vi "Autonomous Independent.vi"() -> ()   [LabVIEW 2016]
doc: "This VI is called when autonomous begins, and will automatically be terminated when autonomous ends. You can carry out timed or sensor driven robot movement independently without needing to return to the caller."
uses:
  <vilib>/Rock Robotics/WPI/Solenoid/WPI_SolenoidValue.ctl
  <vilib>/Rock Robotics/WPI/ThirdParty/CanMotor/TalonSRX/WPI_CANTalonSRX_APIControlMode.ctl
  <vilib>/Rock Robotics/Network Tables/NT Read String.vi
  <vilib>/Rock Robotics/WPI/Utilities/WPI_GetSetVariantRefNum.vi
  <vilib>/Rock Robotics/WPI/Solenoid/WPI_SolenoidSetEnum.vi
  <vilib>/Rock Robotics/Network Tables/NT Read Number.vi
  <vilib>/addons/control/pid/pid.llb/PID (DBL).vi
  Robot Global Data.vi
  <vilib>/Rock Robotics/Network Tables/NT Read Boolean.vi
  <vilib>/addons/control/pid/NI_PID_pid.lvlib
  navX Library v2/navX Library v2.lvlib
panel:
  out "DriveStraight 11":T1(graph)
  in  "ForwardPID 9":T2={"proportional gain (Kc)"=0.001, "integral time (Ti, min)"=0.1, "derivative time (Td, min)"=0.0}
  out "DriveStraight 10":T1(graph)
  in  "ForwardPID 8":T2={"proportional gain (Kc)"=0.001, "integral time (Ti, min)"=0.1, "derivative time (Td, min)"=0.0}
  out "DriveStraight 5":T1(graph)
  in  "ForwardPID 5":T2={"proportional gain (Kc)"=0.001, "integral time (Ti, min)"=0.1, "derivative time (Td, min)"=0.0}
  out "DriveStraight 4":T1(graph)
  in  "ForwardPID 4":T2={"proportional gain (Kc)"=0.001, "integral time (Ti, min)"=0.1, "derivative time (Td, min)"=0.0}
  in  "PID gains R 5":T2={"proportional gain (Kc)"=0.65, "integral time (Ti, min)"=0.01, "derivative time (Td, min)"=0.0} {"derivative time (Td, min)" format="%.3f"; "integral time (Ti, min)" format="%.6f"; "proportional gain (Kc)" format="%.6f"}
  in  "Range 5":cluster{"output high":dbl, "output low":dbl}={"output high"=1.0, "output low"=-0.5} {"output low" format="%.2f"; "output high" format="%.2f"}
  in  "PID gains L 5":T2={"proportional gain (Kc)"=0.65, "integral time (Ti, min)"=0.01, "derivative time (Td, min)"=0.0} {"derivative time (Td, min)" format="%.3f"; "integral time (Ti, min)" format="%.6f"; "proportional gain (Kc)" format="%.6f"}
  in  "PID gains R 4":T2={"proportional gain (Kc)"=0.65, "integral time (Ti, min)"=0.01, "derivative time (Td, min)"=0.0} {"derivative time (Td, min)" format="%.3f"; "integral time (Ti, min)" format="%.6f"; "proportional gain (Kc)" format="%.6f"}
  in  "Range 4":cluster{"output high":dbl, "output low":dbl}={"output high"=1.0, "output low"=-0.5} {"output low" format="%.2f"; "output high" format="%.2f"}
  in  "PID gains L 4":T2={"proportional gain (Kc)"=0.65, "integral time (Ti, min)"=0.01, "derivative time (Td, min)"=0.0} {"derivative time (Td, min)" format="%.3f"; "integral time (Ti, min)" format="%.6f"; "proportional gain (Kc)" format="%.6f"}
  in  "PID gains R 3":T2={"proportional gain (Kc)"=0.65, "integral time (Ti, min)"=0.01, "derivative time (Td, min)"=0.0} {"derivative time (Td, min)" format="%.3f"; "integral time (Ti, min)" format="%.6f"; "proportional gain (Kc)" format="%.6f"}
  in  "Range 3":cluster{"output high":dbl, "output low":dbl}={"output high"=1.0, "output low"=-0.5} {"output low" format="%.2f"; "output high" format="%.2f"}
  in  "PID gains L 3":T2={"proportional gain (Kc)"=0.65, "integral time (Ti, min)"=0.01, "derivative time (Td, min)"=0.0} {"derivative time (Td, min)" format="%.3f"; "integral time (Ti, min)" format="%.6f"; "proportional gain (Kc)" format="%.6f"}
  in  "PID gains R 2":T2={"proportional gain (Kc)"=0.65, "integral time (Ti, min)"=0.01, "derivative time (Td, min)"=0.0} {"derivative time (Td, min)" format="%.3f"; "integral time (Ti, min)" format="%.6f"; "proportional gain (Kc)" format="%.6f"}
  in  "Range 2":cluster{"output high":dbl, "output low":dbl}={"output high"=1.0, "output low"=-0.5} {"output low" format="%.2f"; "output high" format="%.2f"}
  in  "PID gains L 2":T2={"proportional gain (Kc)"=0.65, "integral time (Ti, min)"=0.01, "derivative time (Td, min)"=0.0} {"derivative time (Td, min)" format="%.3f"; "integral time (Ti, min)" format="%.6f"; "proportional gain (Kc)" format="%.6f"}
  in  "Fizone":dbl=3000.0
  in  "FI":dbl=0.001
  in  "FP":dbl=0.2
  in  "FrontSpeed":dbl=-22000.0
  out "DriveStraight 7":T1(graph)
  out "DriveStraight 6":T1(graph)
  in  "ForwardPID 3":T2={"proportional gain (Kc)"=0.001, "integral time (Ti, min)"=0.1, "derivative time (Td, min)"=0.0}
  in  "Hizone":dbl=3000.0
  in  "sizone":dbl=3000.0
  in  "ShootSpeed":dbl=-20000.0
  in  "SI":dbl=0.001
  in  "SP":dbl=0.2
  in  "HI":dbl=0.001
  in  "HP":dbl=0.2
  in  "HopperSpeed":dbl=-22000.0
  out "DriveStraight 3":T1(graph)
  out "DriveStraight 2":T1(graph)
  in  "ForwardPID 2":T2={"proportional gain (Kc)"=0.001, "integral time (Ti, min)"=0.1, "derivative time (Td, min)"=0.0}
  in  "RightPID":T2
  in  "ForwardPID":T2={"proportional gain (Kc)"=0.001, "integral time (Ti, min)"=0.1, "derivative time (Td, min)"=0.0}
  out "DriveStraight":T1(graph)
  in  "Center":dbl=160.0 format="%#_13g"
  in  "MOE":dbl=25.0 format="%#_13g"
  in  "Speed 2":dbl=0.45 format="%#_13g"
  in  "PID gains L":T2={"proportional gain (Kc)"=0.65, "integral time (Ti, min)"=0.01, "derivative time (Td, min)"=0.0} {"derivative time (Td, min)" format="%.3f"; "integral time (Ti, min)" format="%.6f"; "proportional gain (Kc)" format="%.6f"}
  in  "PID gains R":T2={"proportional gain (Kc)"=0.65, "integral time (Ti, min)"=0.01, "derivative time (Td, min)"=0.0} {"derivative time (Td, min)" format="%.3f"; "integral time (Ti, min)" format="%.6f"; "proportional gain (Kc)" format="%.6f"}
  in  "Range":cluster{"output high":dbl, "output low":dbl}={"output high"=1.0, "output low"=-0.5} {"output low" format="%.2f"; "output high" format="%.2f"}
  in  "Speed":dbl=1.0 format="%#_13g"
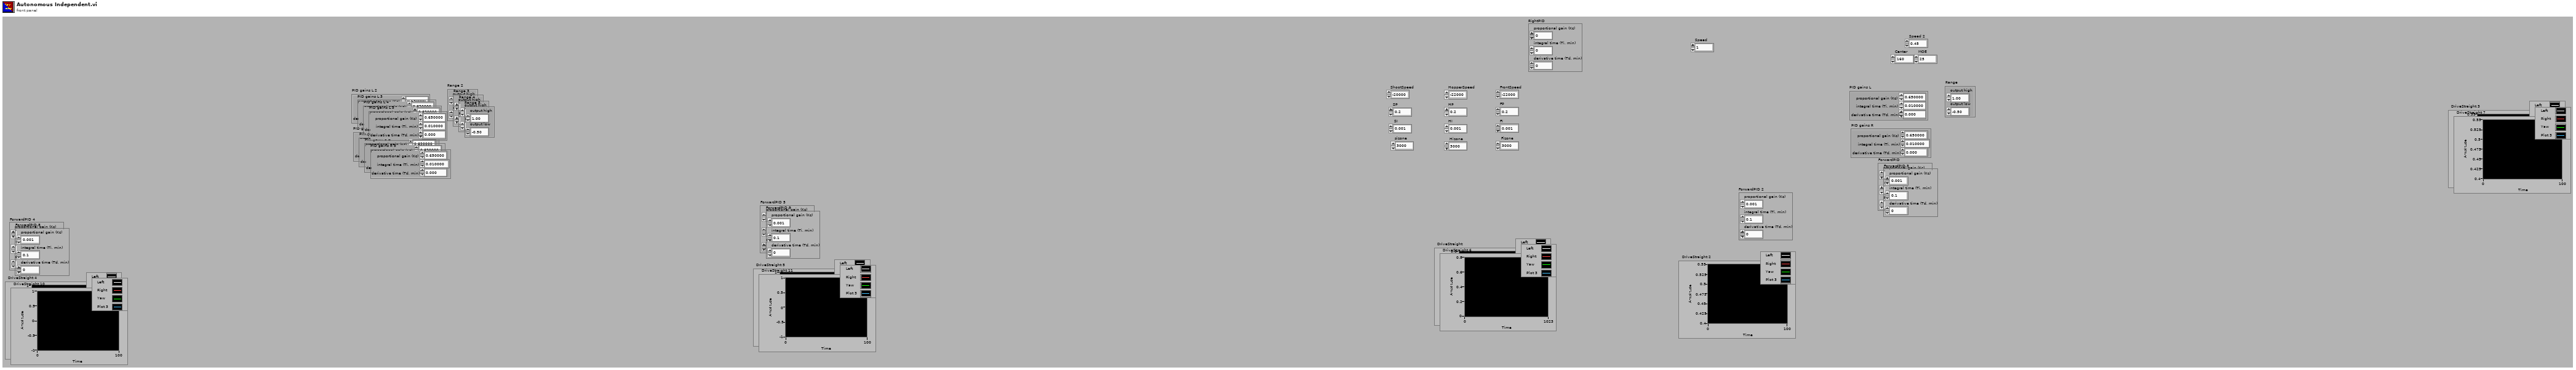
[diagram p1: front panel]
types:
  T1 = cluster{"[0]":dbl, "[1]":dbl, "[2]":dbl, "[3]":dbl, "[4]":dbl, "[5]":dbl, "[6]":dbl, "[7]":dbl, "[8]":dbl}
  T2 = cluster{"proportional gain (Kc)":dbl, "integral time (Ti, min)":dbl, "derivative time (Td, min)":dbl}
  T3 = typedef "WPI_SolenoidValue.ctl" = enum16{"Off", "On", "Forward", "Reverse"}
  T4 = typedef "WPI_CANTalonSRX_APIControlMode.ctl" = enum8{"Percent VBus", "Speed", "Position", "Slave", "Unchanged / Invalid", "Voltage Compensation", "Current", "Motion Profile", "Motion Magic"}
  T5 = typedef "WPI_RobotDriveDevRef.ctl" = cluster{"DevStatus":errorcluster, "Motors[]":T6[], "Square Inputs":bool, "Max Output":dbl}
  T6 = typedef "WPI_MotorControlDeviceRef.ctl" = cluster{"DeviceStatus":errorcluster, "Type":T7, "PWM":cluster{"PWM Channel":T8, "DeadBand":T9}, "CAN":cluster{"Device Number":u8, "SetOutput VI Ref":variant, "GetOutput VI Ref":variant, "Enable VI Ref":variant, "Disable VI Ref":variant, "Data":variant}, "Invert":bool}
  T7 = typedef "WPI_MotorControlType.ctl" = enum16{"PWM", "CAN"}
  T8 = typedef "FPGA_DIOPWMChannel.ctl" = enum8{"PWM 0", "PWM 1", "PWM 2", "PWM 3", "PWM 4", "PWM 5", "PWM 6", "PWM 7", "PWM 8", "PWM 9", "PWM MXP 0", "PWM MXP 1", "PWM MXP 2", "PWM MXP 3", "PWM MXP 4", "PWM MXP 5", "PWM MXP 6", "PWM MXP 7", "PWM MXP 8", "PWM MXP 9", "Invalid"}
  T9 = typedef "WPI_PWMDeadband.ctl" = cluster{"Name":string, "maxPositivePwm":i32, "minPositivePwm":i32, "centerPwm":i32, "maxNegativePwm":i32, "minNegativePwm":i32, "angularRange":u16}
  T10 = typedef "WPI_SolenoidDevRef.ctl" = cluster{"DevStatus":errorcluster, "Pneumatics Control Module":u8, "Forward Solenoid Channel":T11, "Reverse Solenoid Channel":T11}
  T11 = typedef "WPI_SolenoidChannel.ctl" = enum8{"Solenoid 0", "Solenoid 1", "Solenoid 2", "Solenoid 3", "Solenoid 4", "Solenoid 5", "Solenoid 6", "Solenoid 7", "Invalid"}
  T12 = typedef "navX Library v2.lvlib/Z900_navX_DeviceTypeDef.ctl" = cluster{"Interface":cluster{"Protocol":T13, "Update Rate (4Hz-100Hz)":u8, "navX Open TypeDef":variant}, "Notify Packet":refnum<notifier>, "Loop VI Refnum":refnum<vi>, "Ready to Close Occurrence Refnum":refnum<k4>}
  T13 = typedef "navX Library v2.lvlib/Z900_navX_ProtocolTypeDef.ctl" = enum16{"SERIAL", "I2C", "SPI"}
  T14 = typedef "WPI_EncoderDevRef.ctl" = cluster{"DevStatus":errorcluster, "EncoderIndex":T15, "CounterIndex":T16, "DistancePerCount":dbl, "Decoding Type":T17}
  T15 = typedef "FPGA_EncoderIdx.ctl" = enum8{"Enc 0", "Enc 1", "Enc 2", "Enc 3", "Enc 4", "Enc 5", "Enc 6", "Enc 7", "Invalid"}
  T16 = typedef "FPGA_CounterCtrSystemIndex.ctl" = enum8{"Ctr 0", "Ctr 1", "Ctr 2", "Ctr 3", "Ctr 4", "Ctr 5", "Ctr 6", "Ctr 7", "Invalid"}
  T17 = typedef "WPI_EncoderType.ctl" = enum16{"1x", "2x", "4x"}
  T18 = cluster{"Yaw":dbl, "Roll":dbl, "Pitch":dbl, "Heading":dbl, "Fused Heading":dbl}
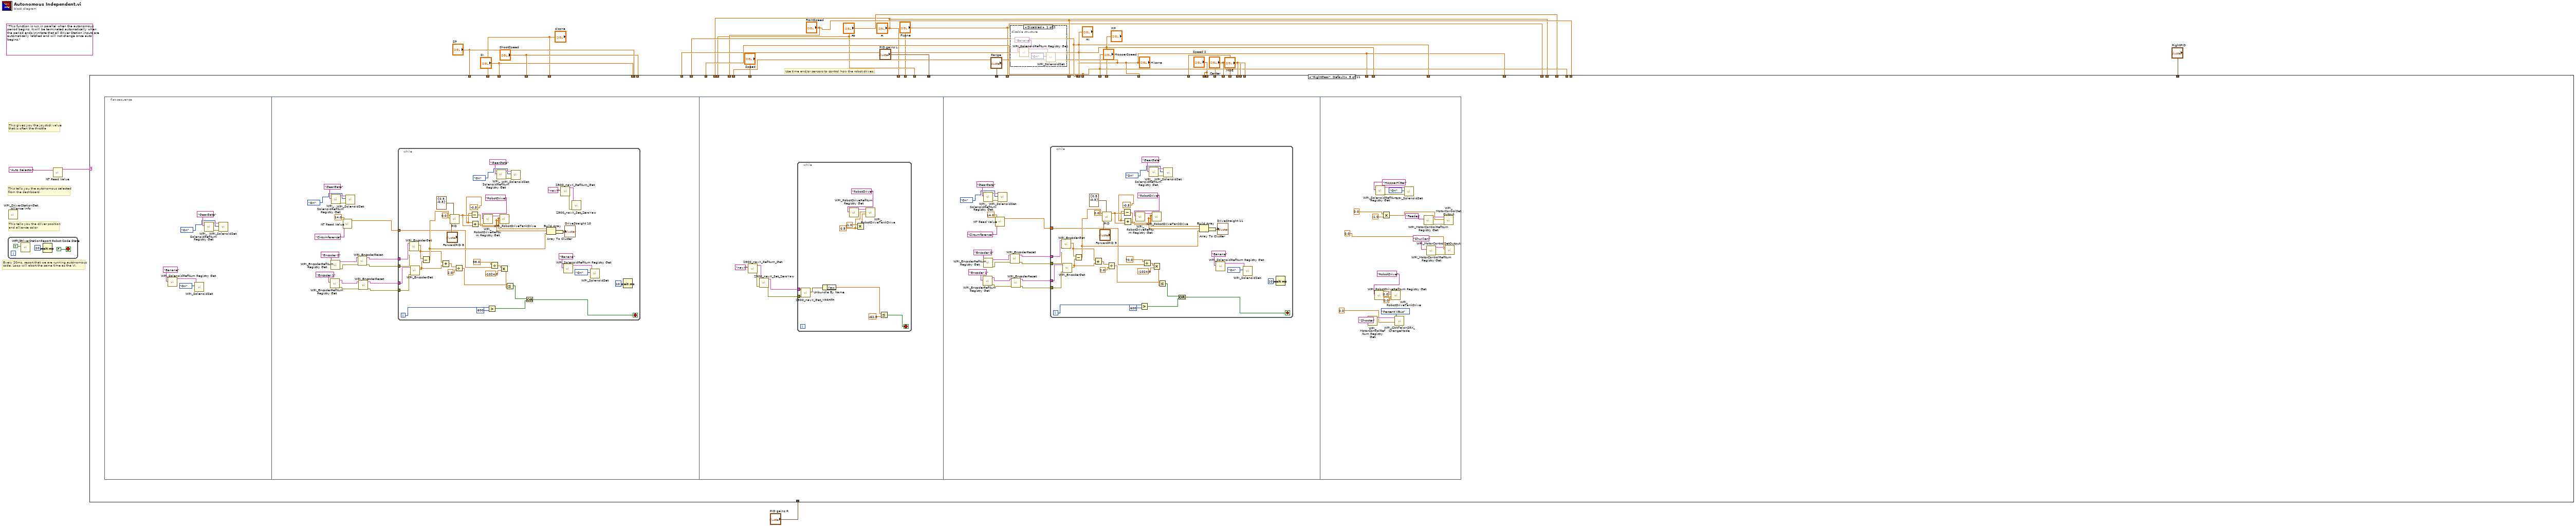
[diagram p0: block diagram]
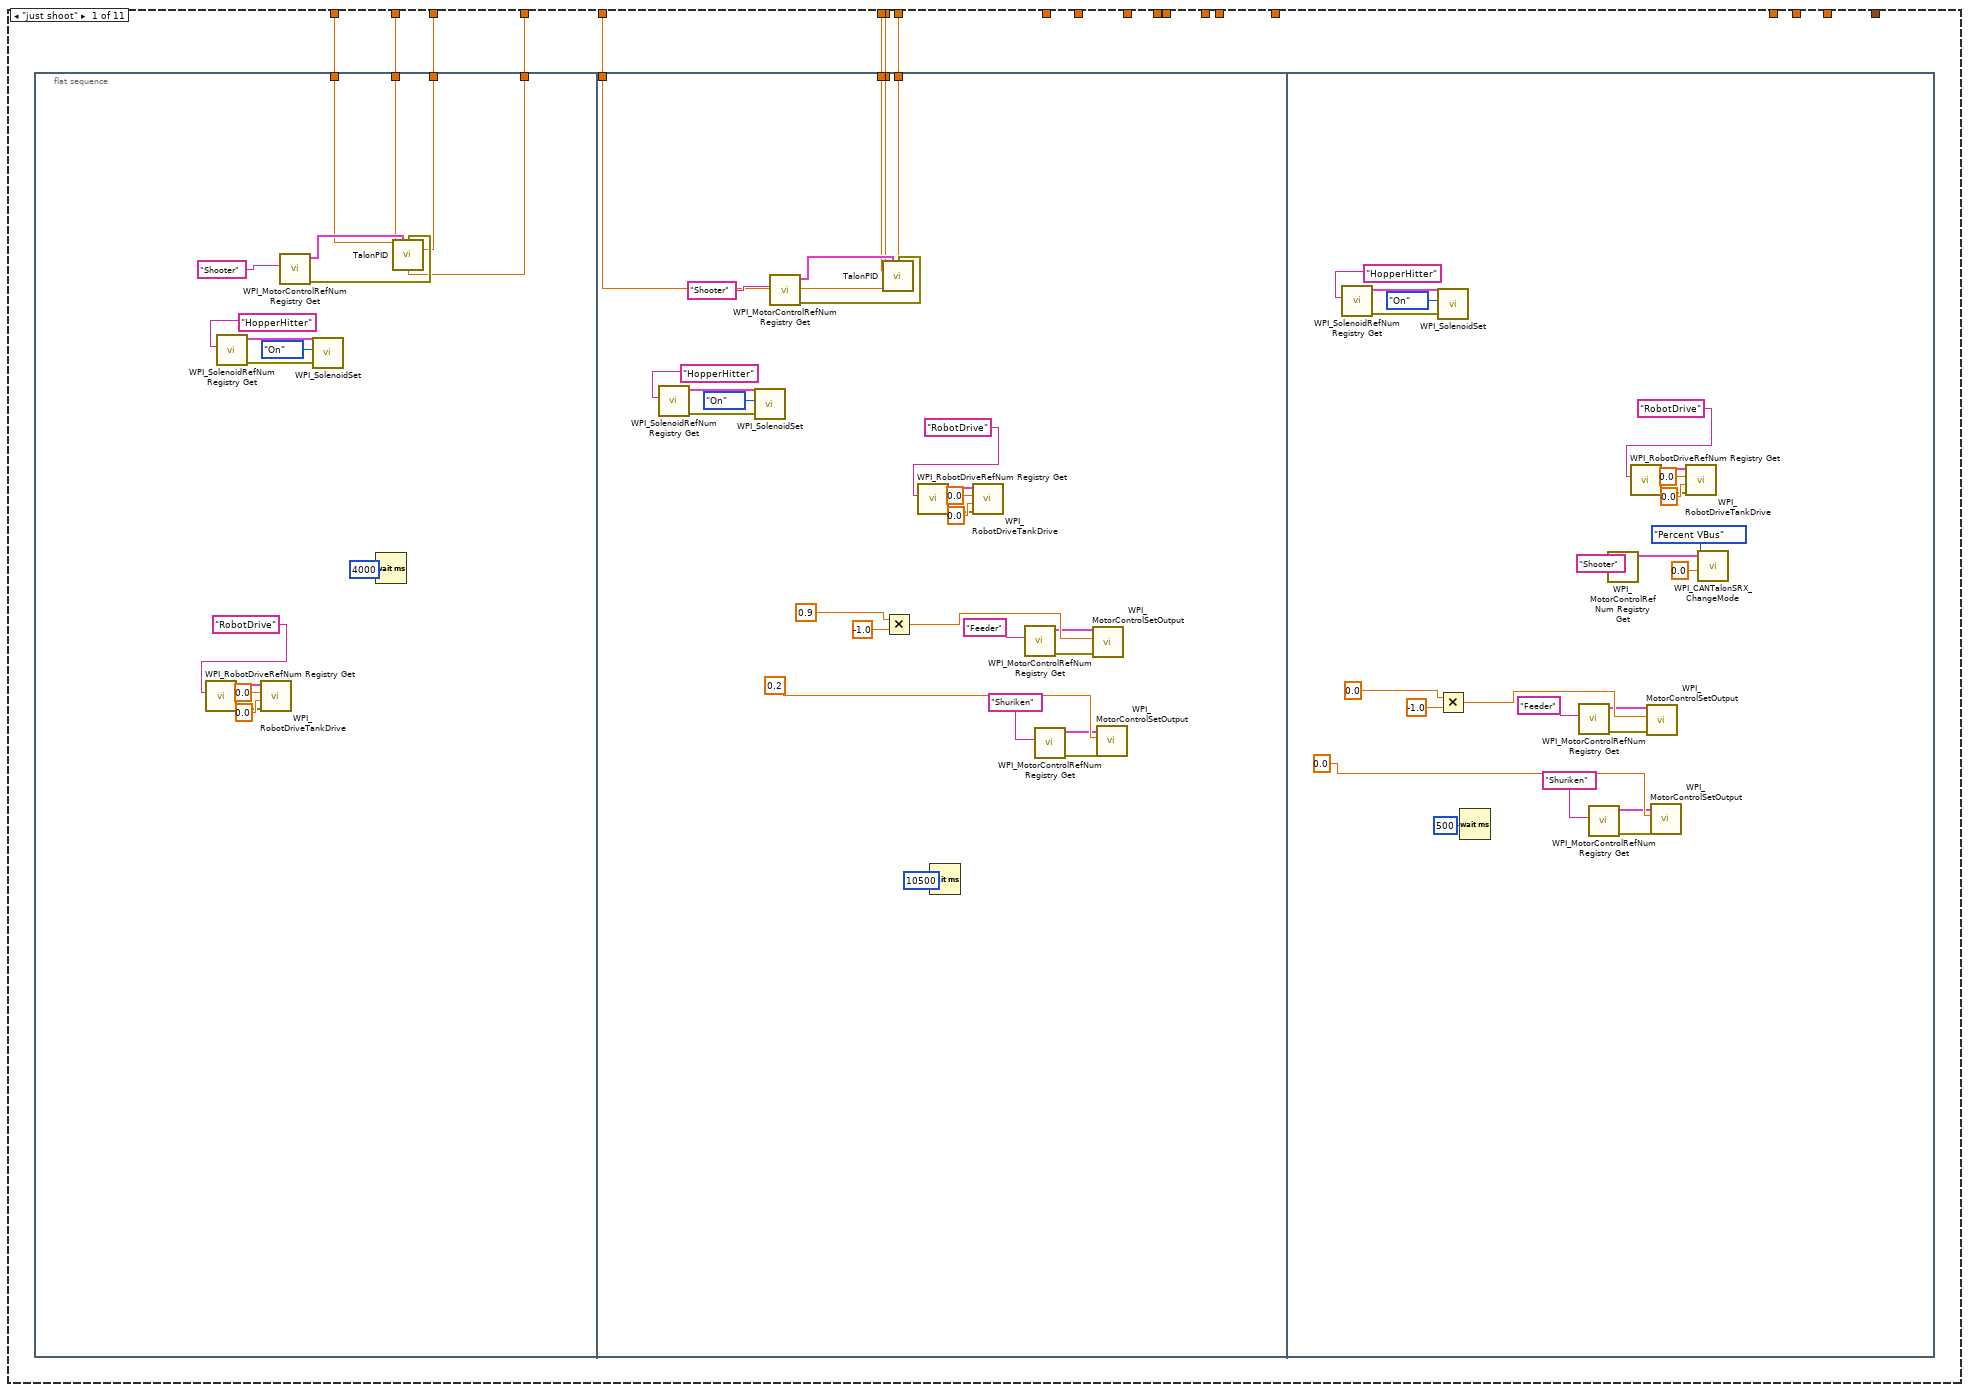
[diagram p3: hidden frame]
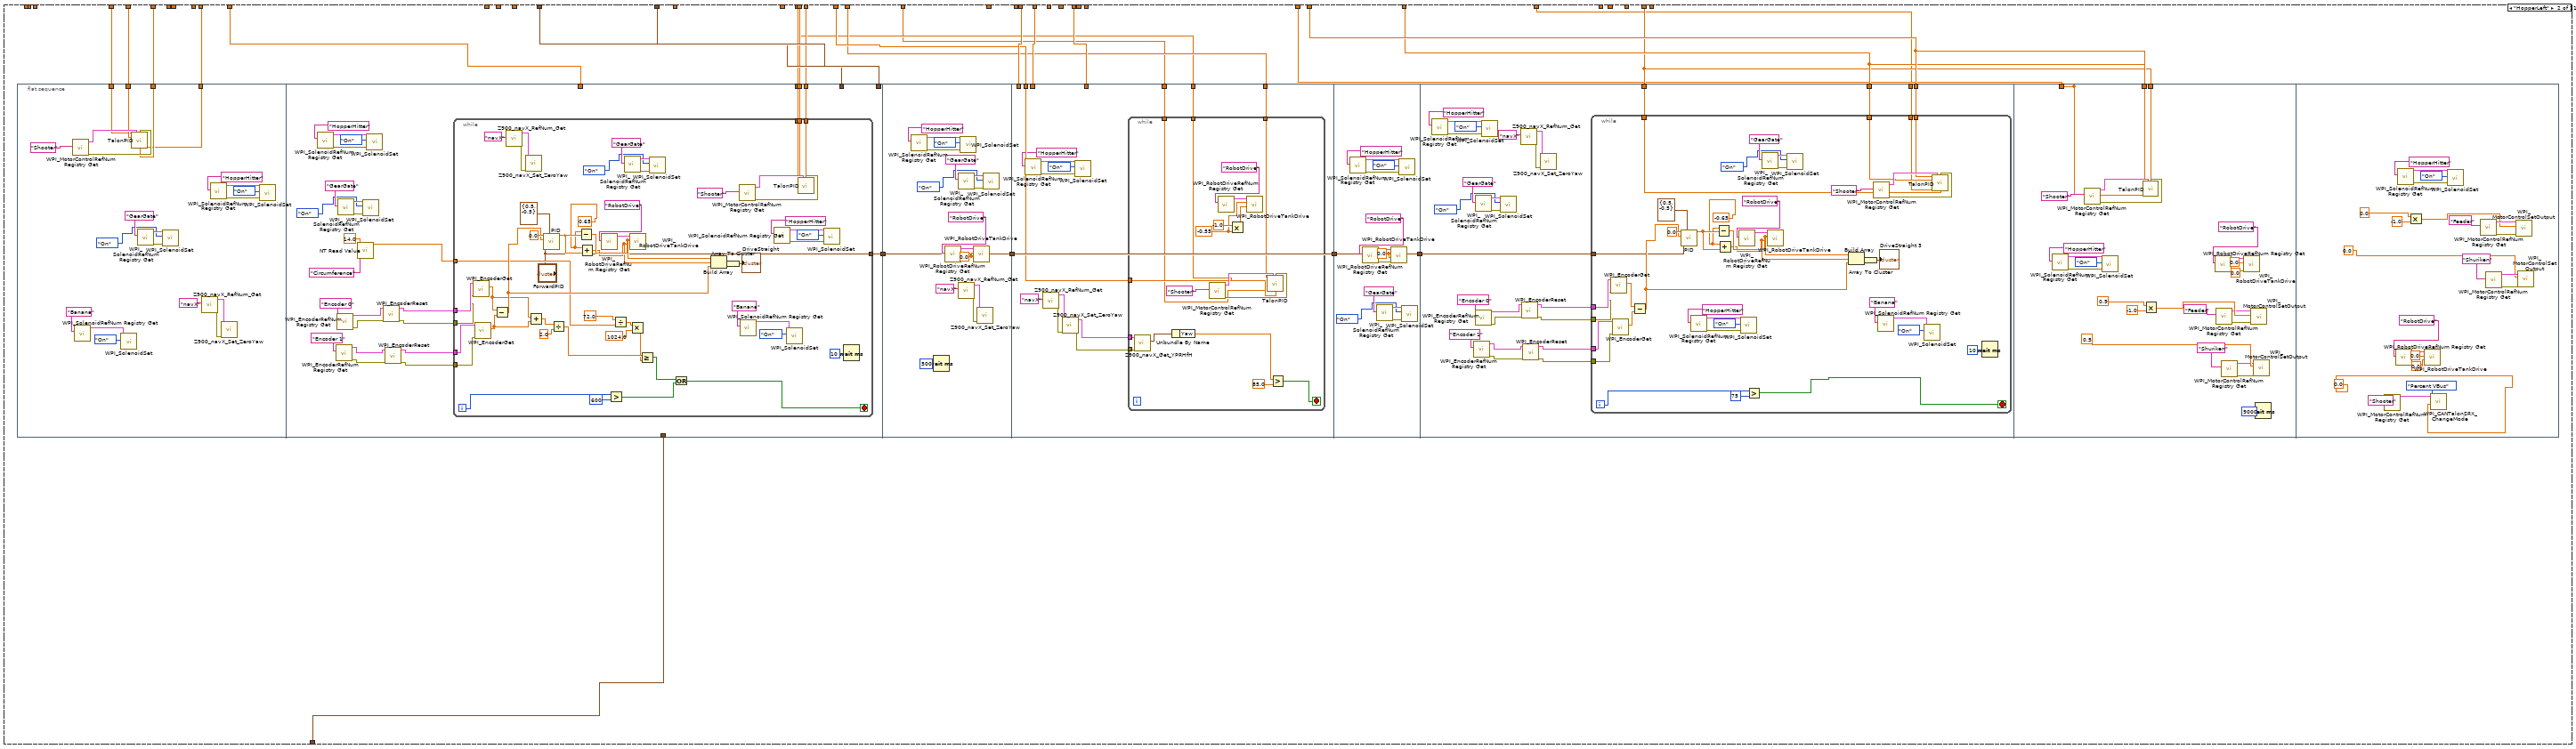
[diagram p4: hidden frame]
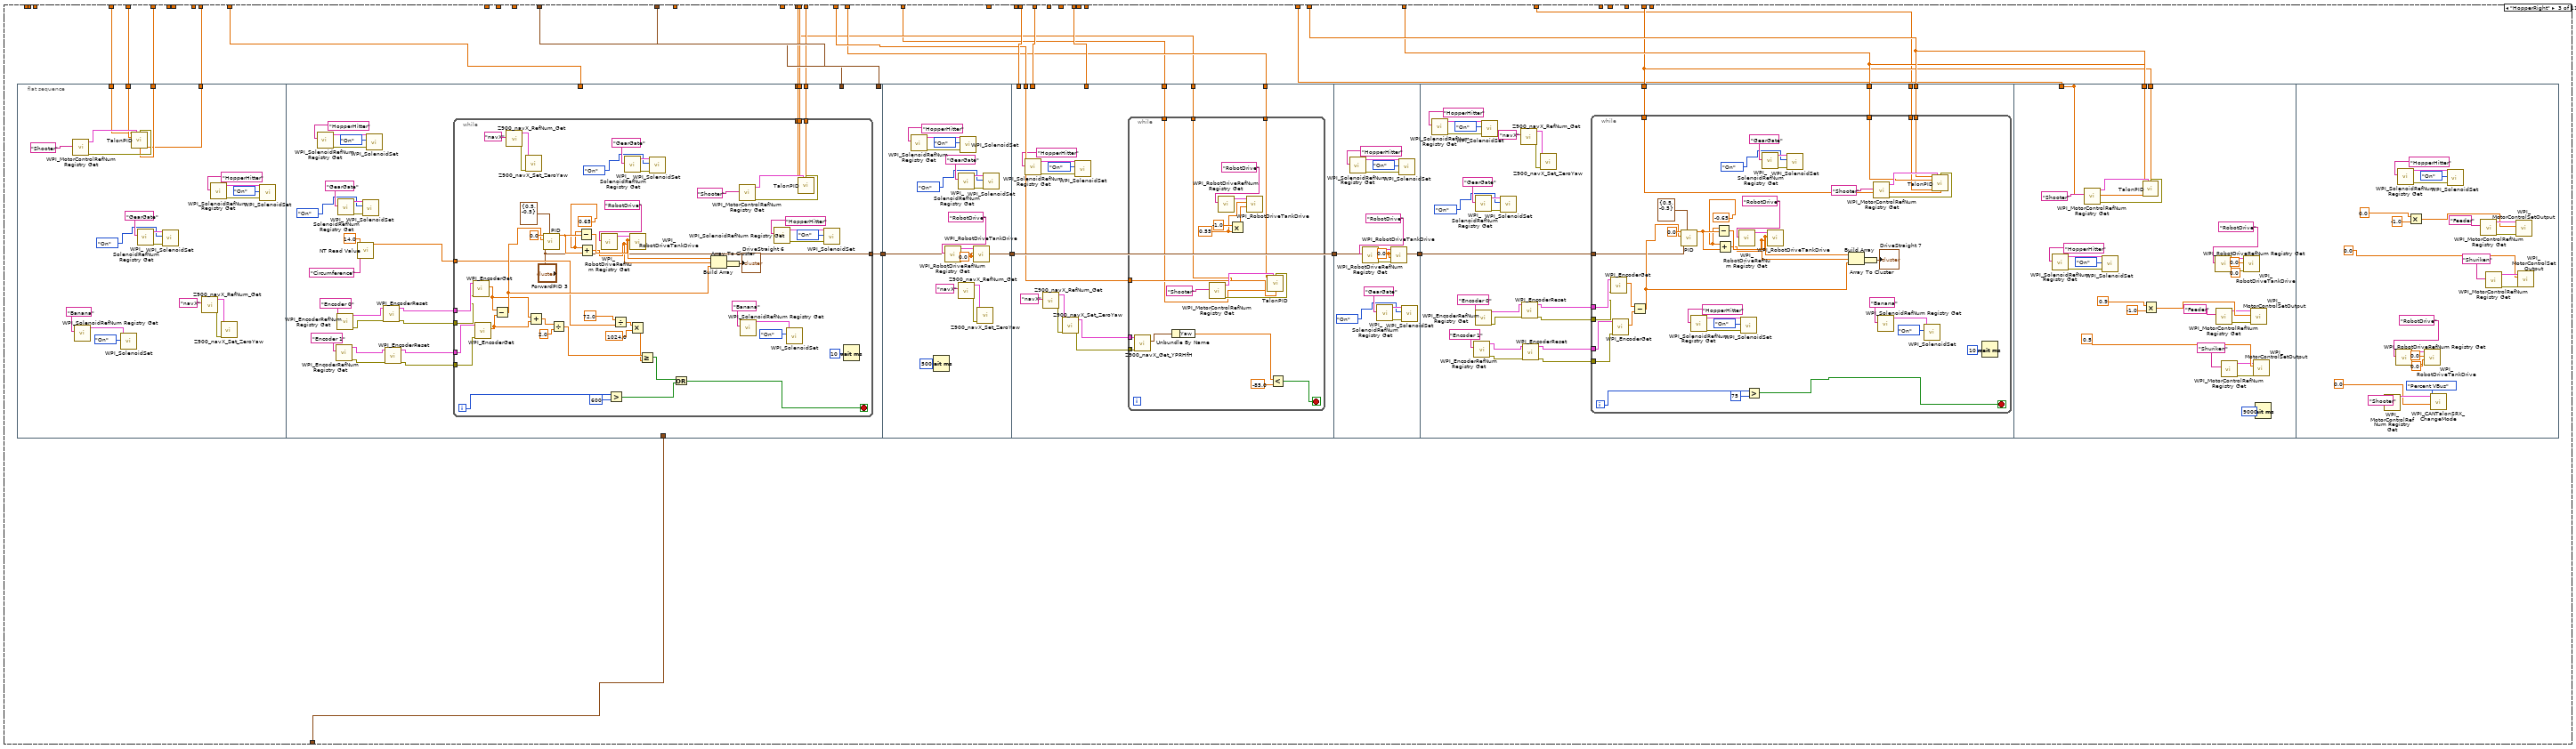
[diagram p5: hidden frame]
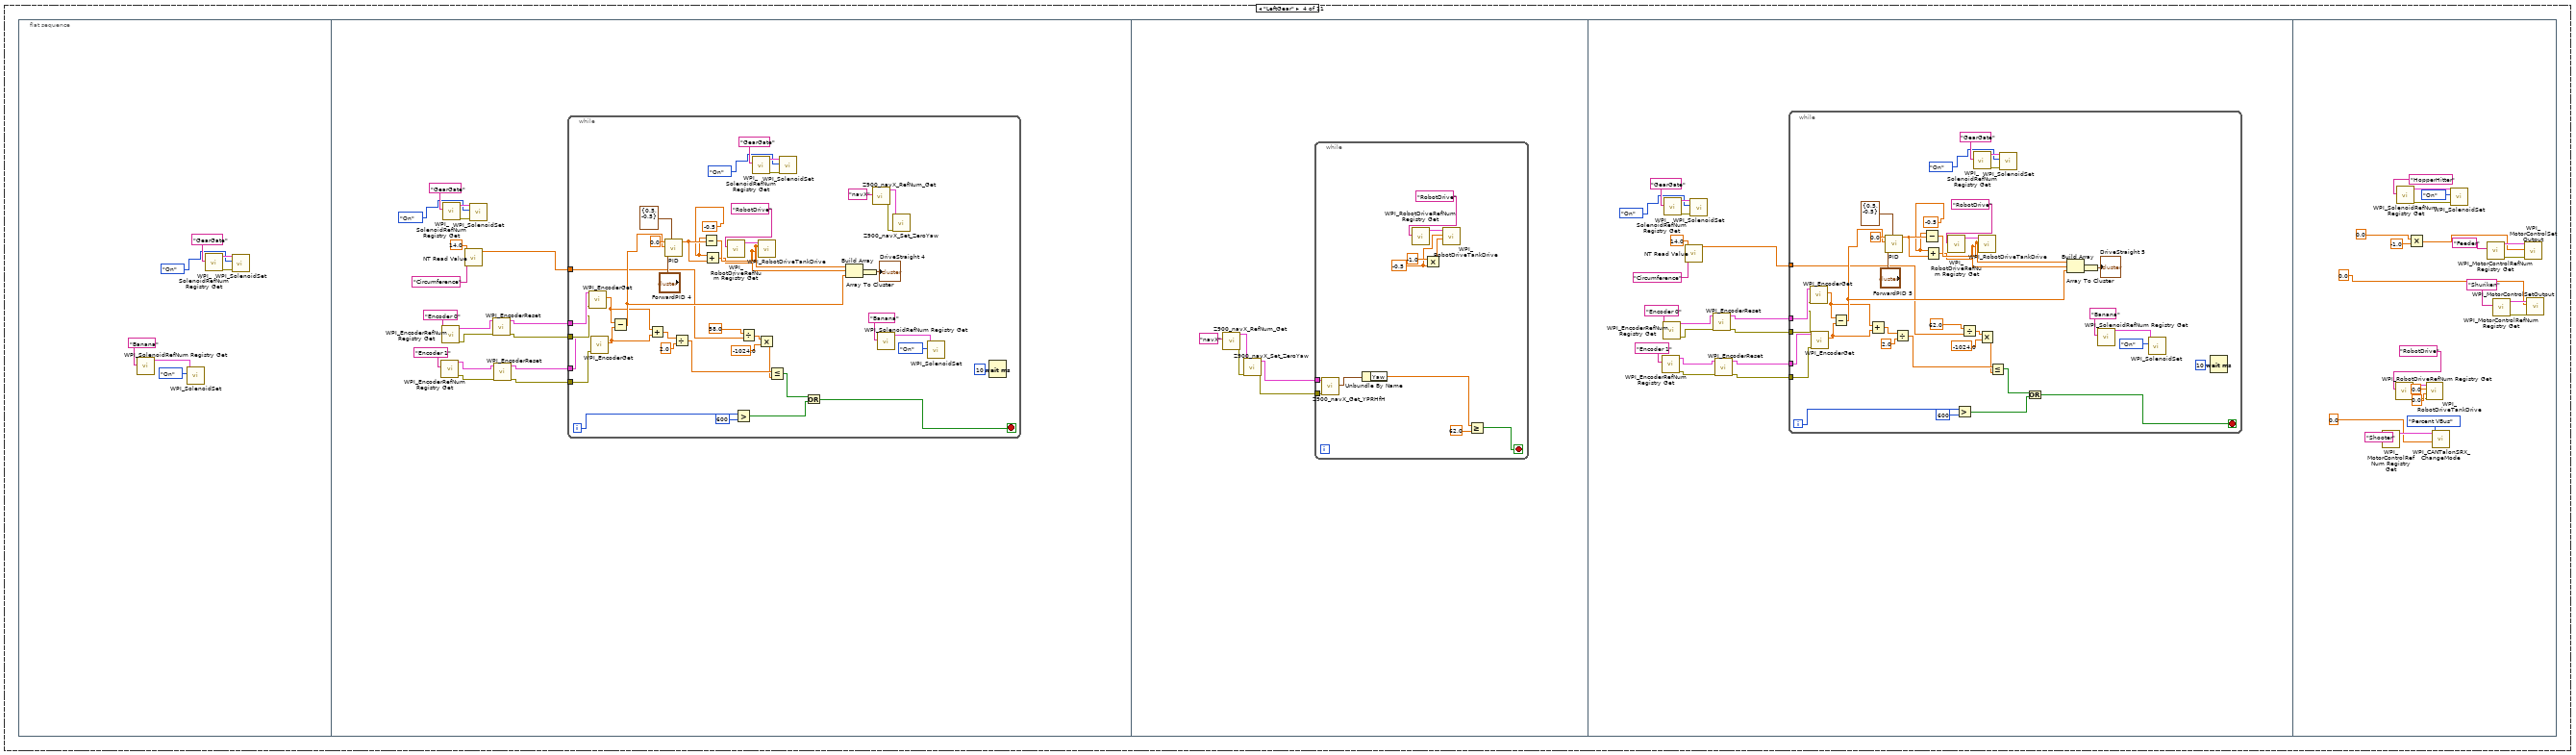
[diagram p6: hidden frame]
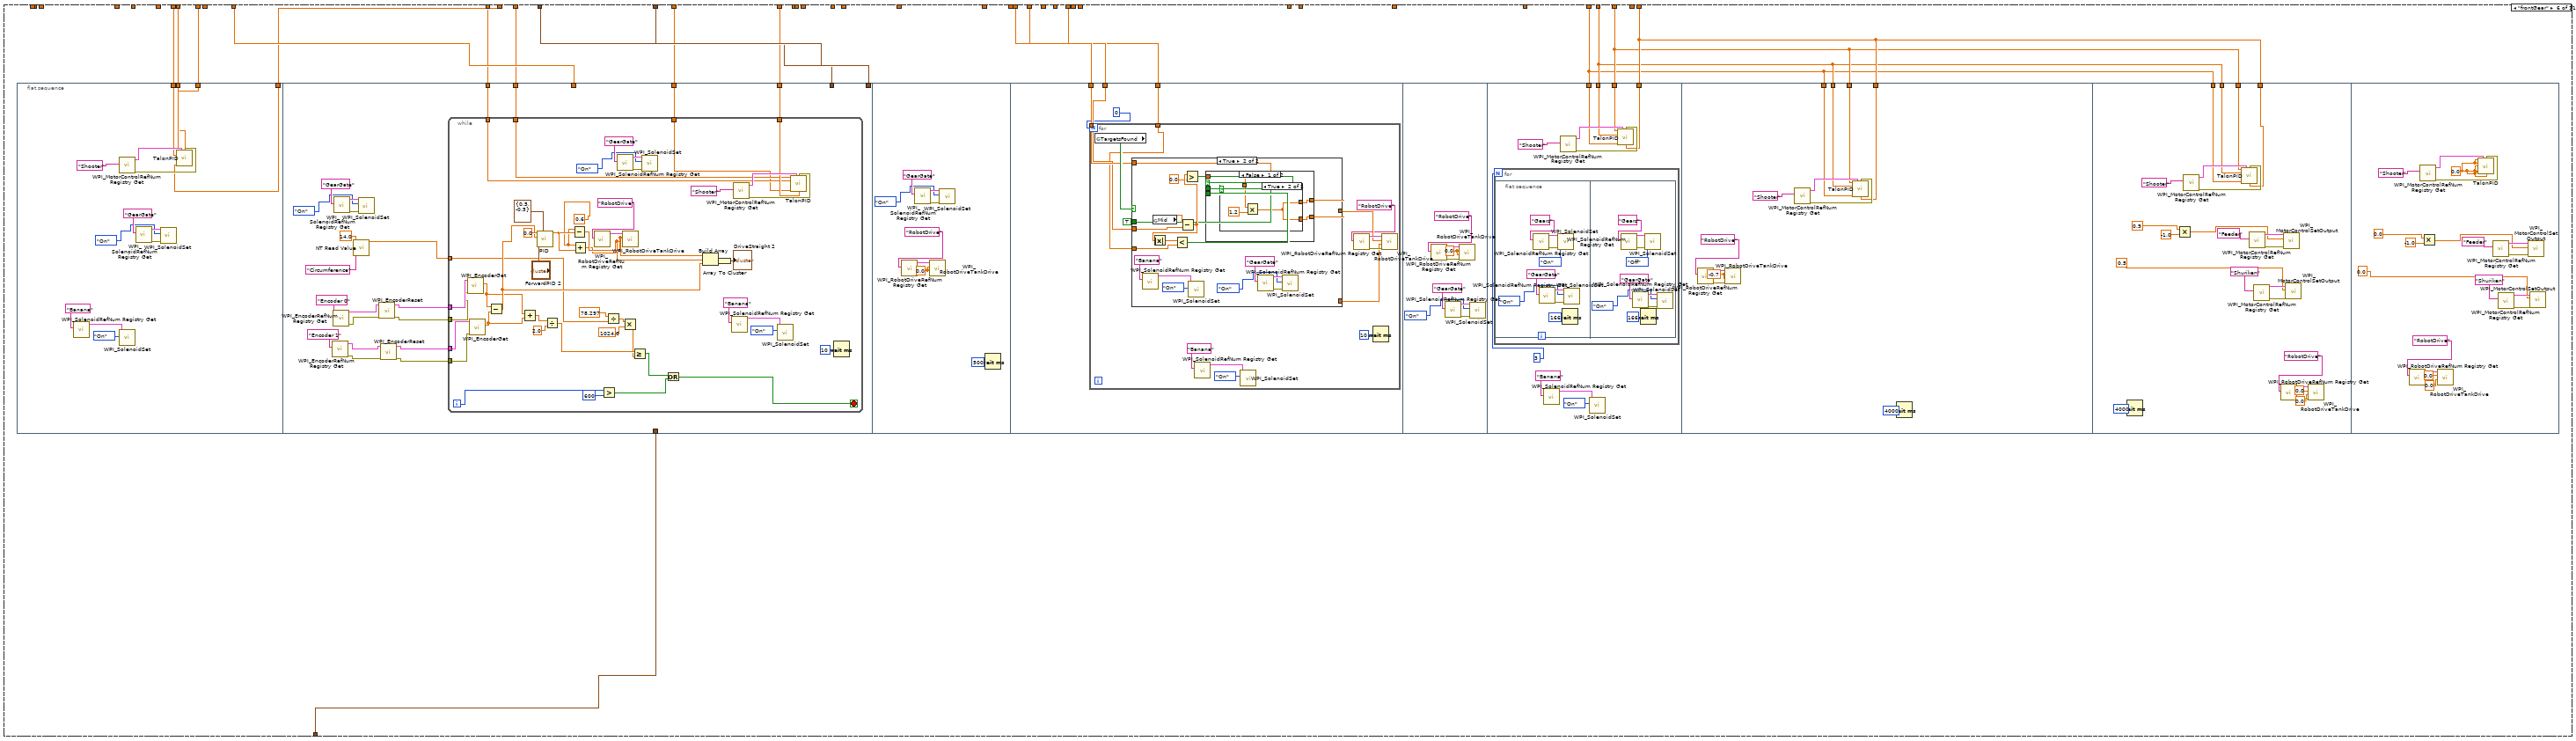
[diagram p7: hidden frame]
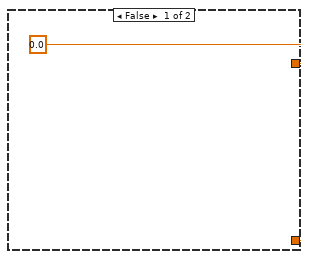
[diagram p8: hidden frame]
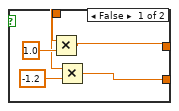
[diagram p9: hidden frame]
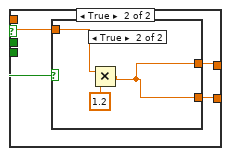
[diagram p10: hidden frame]
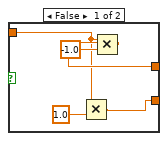
[diagram p11: hidden frame]
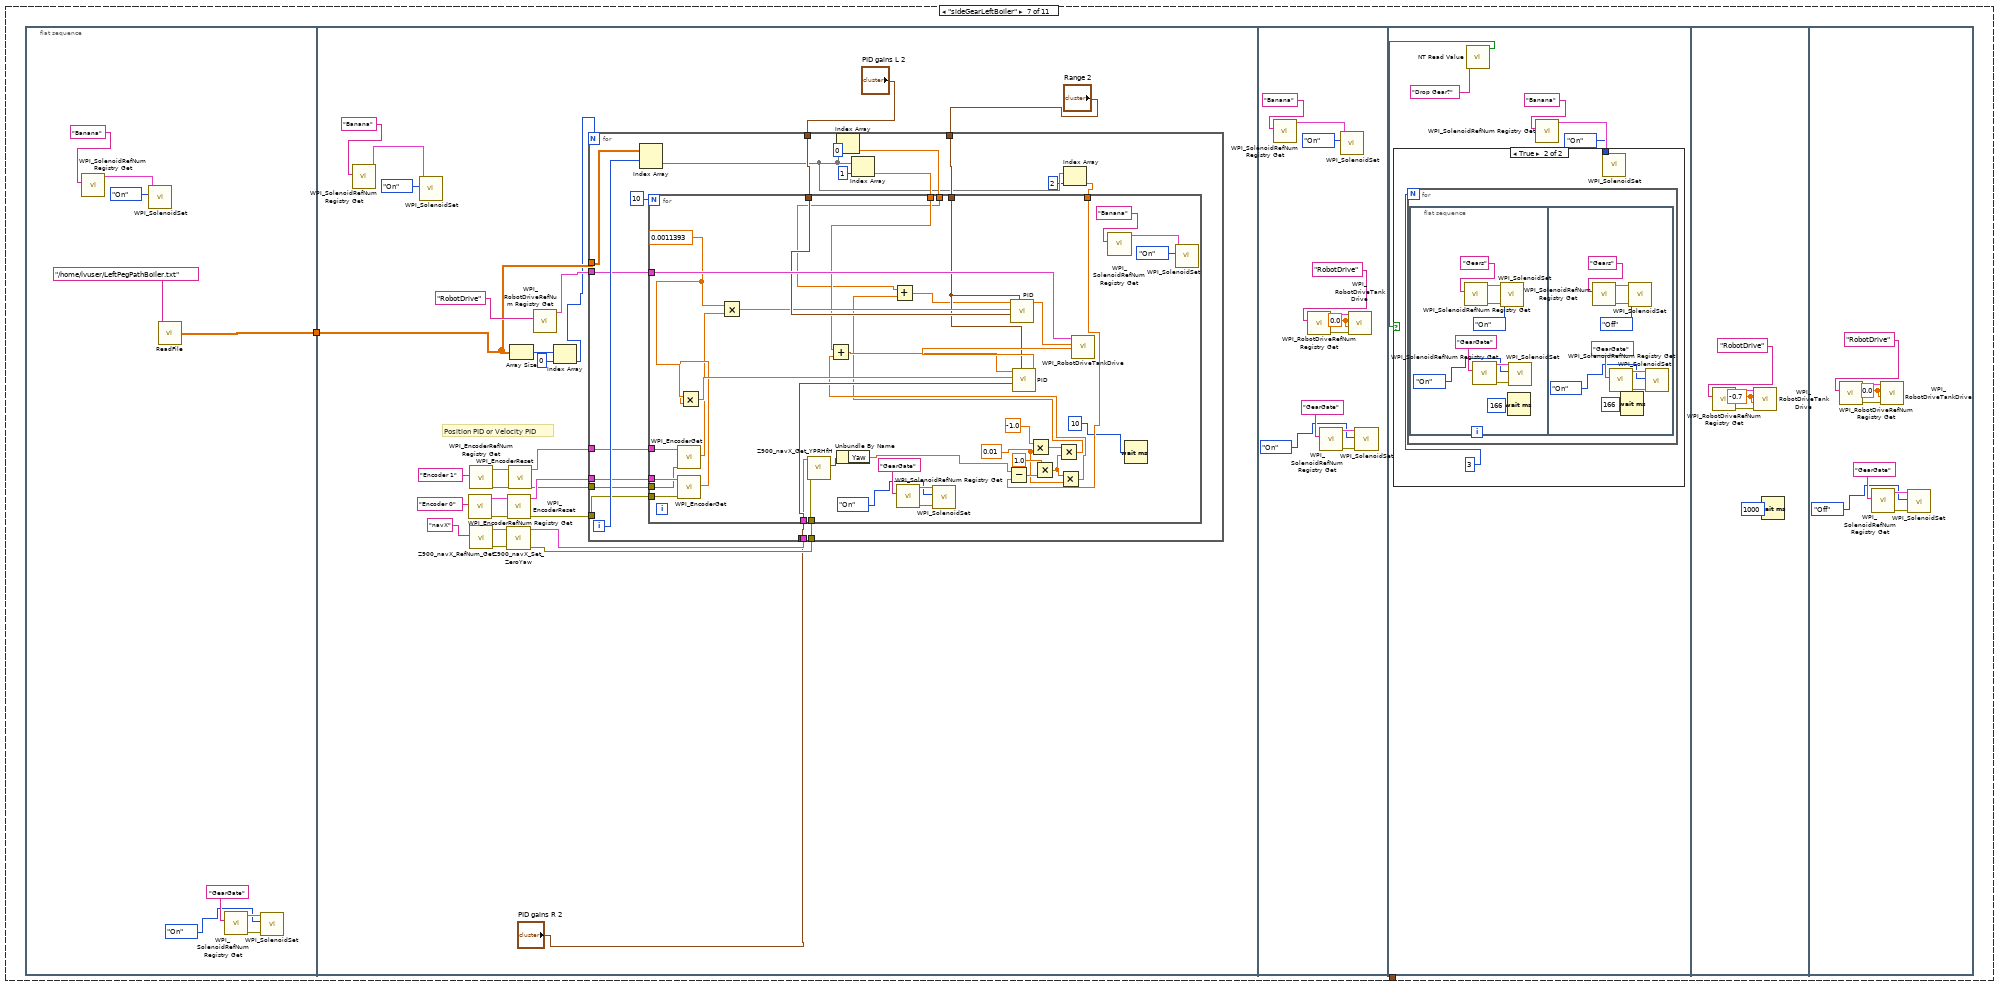
[diagram p12: hidden frame]
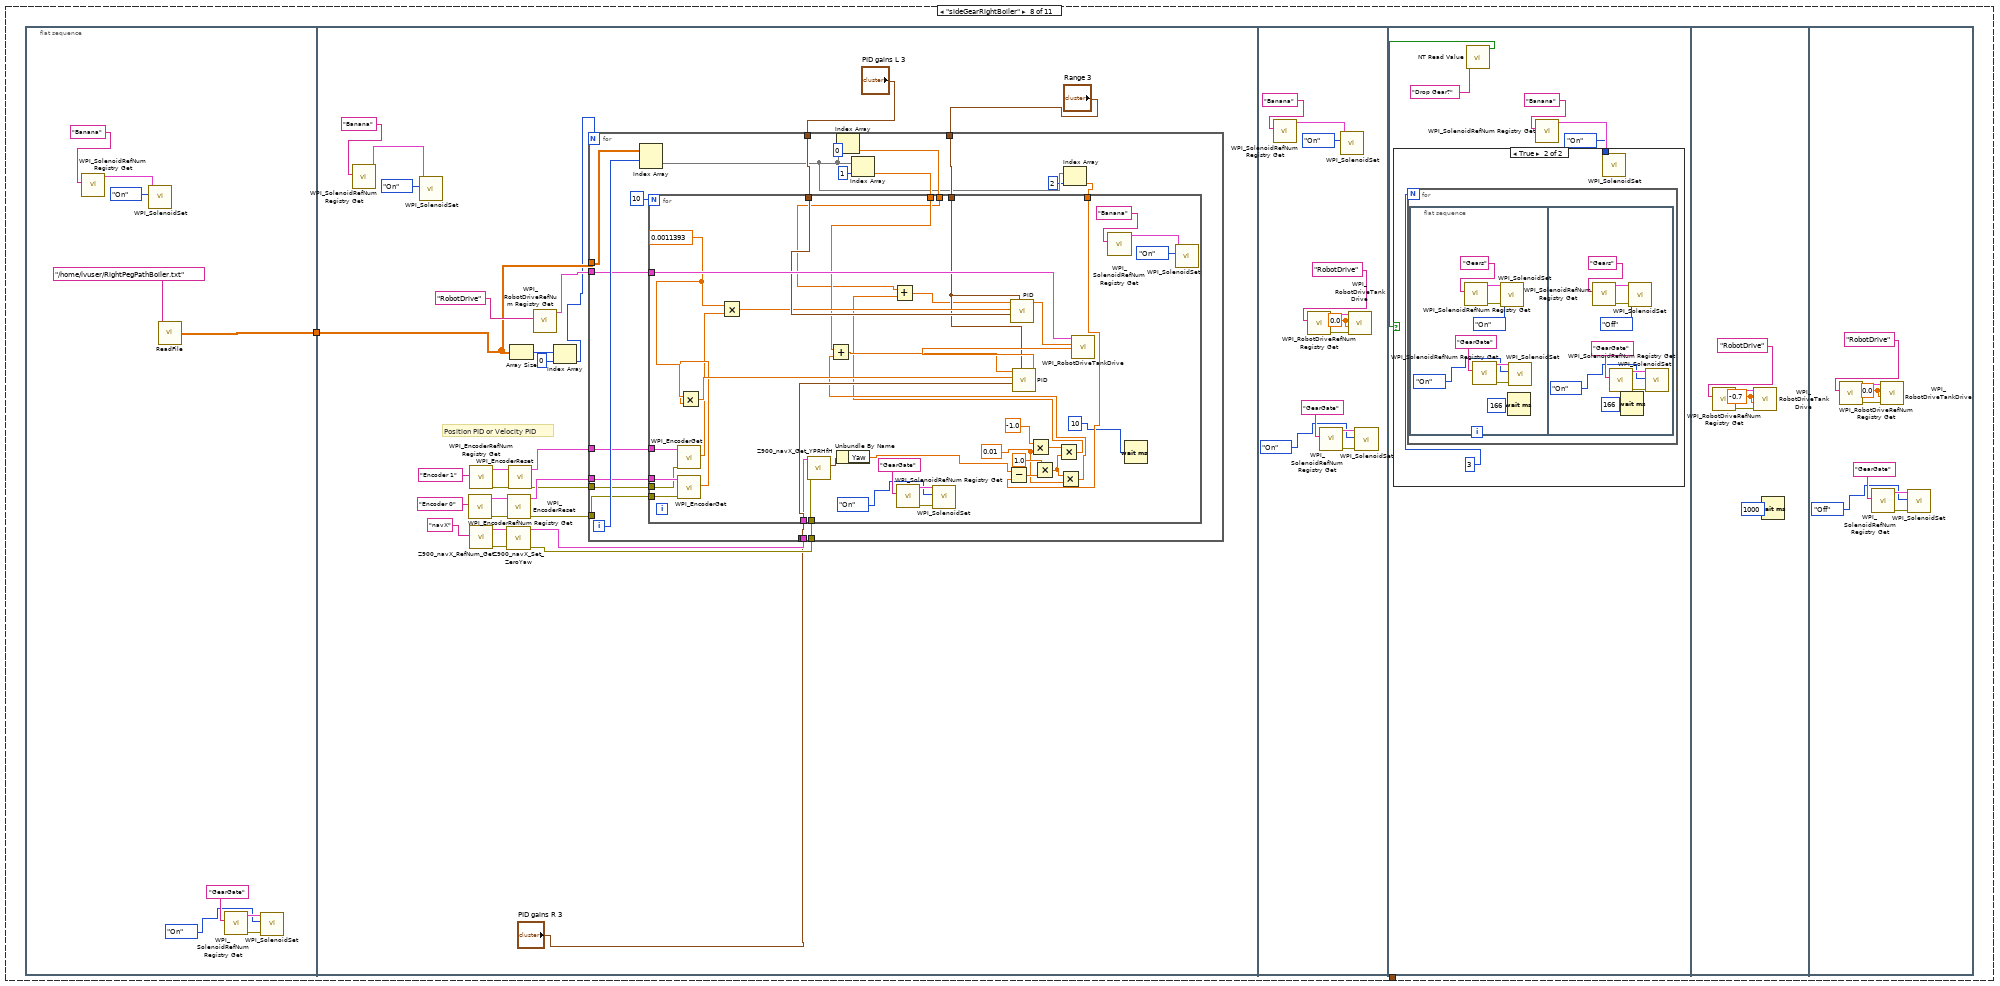
[diagram p14: hidden frame]
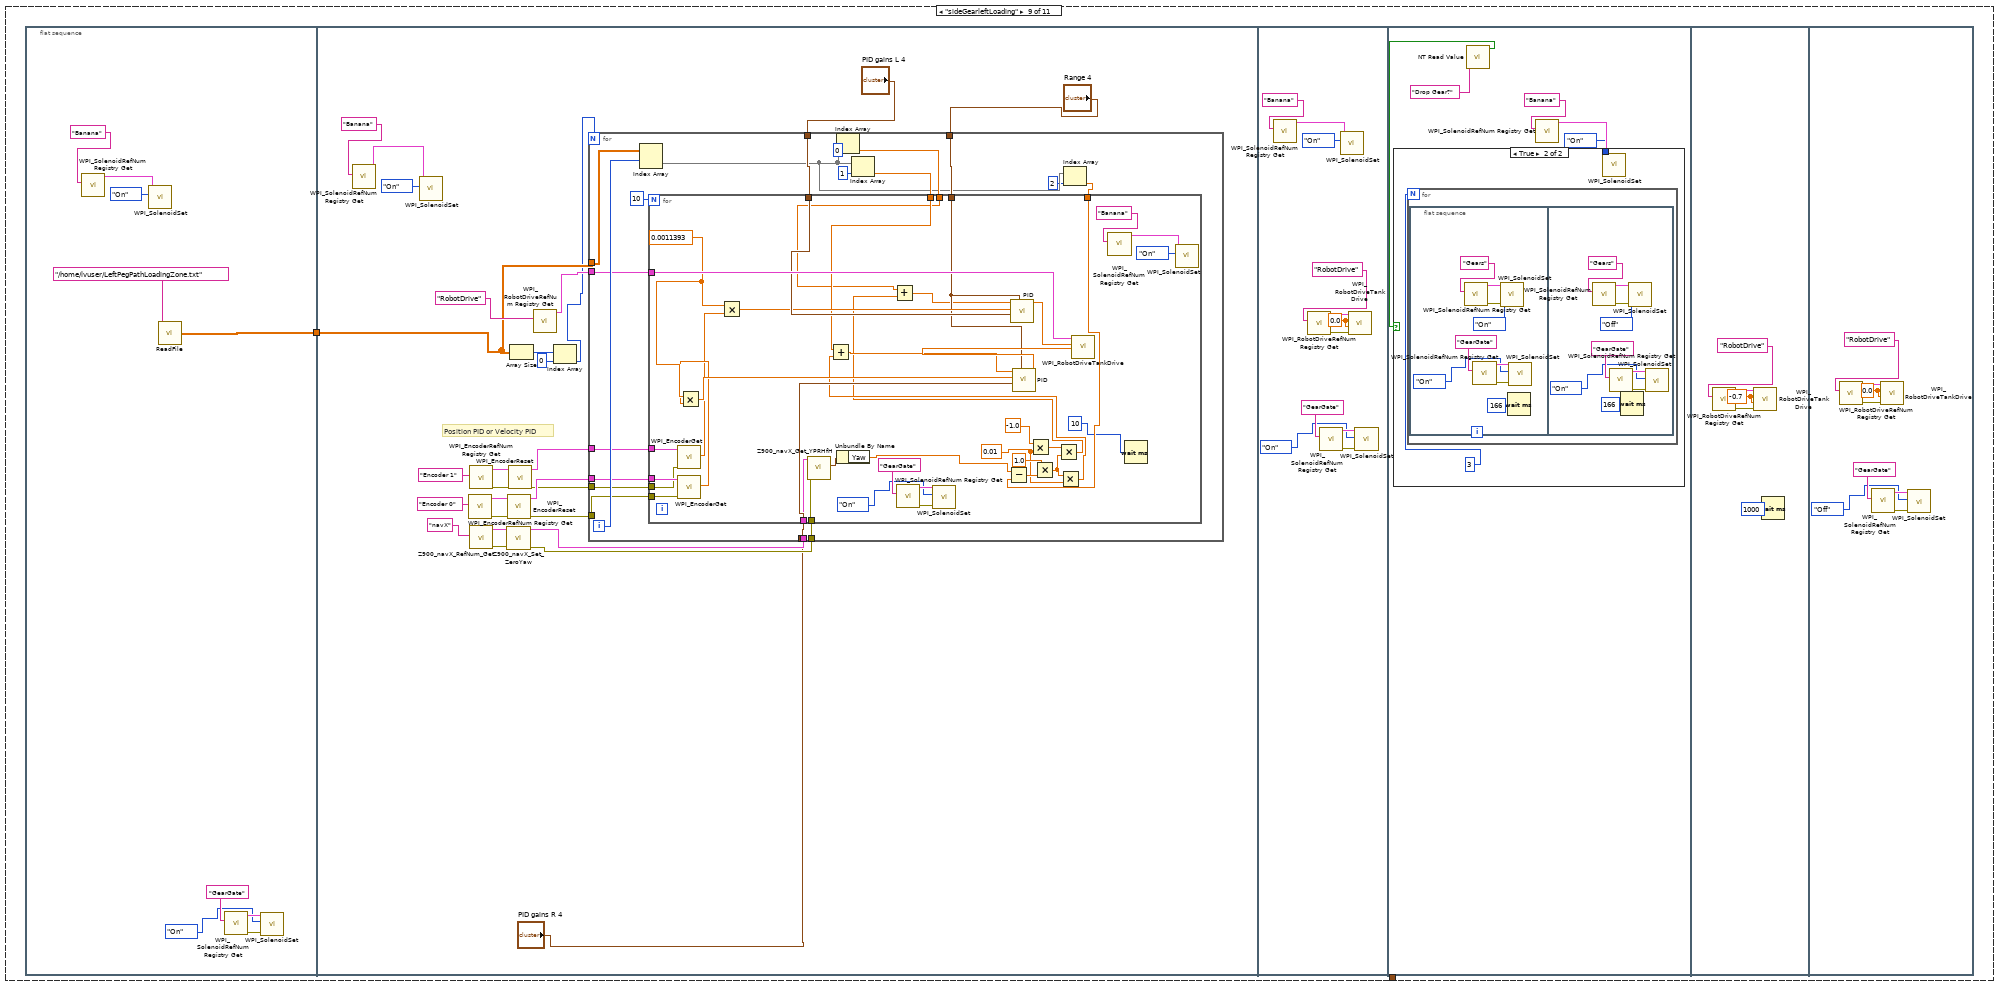
[diagram p16: hidden frame]
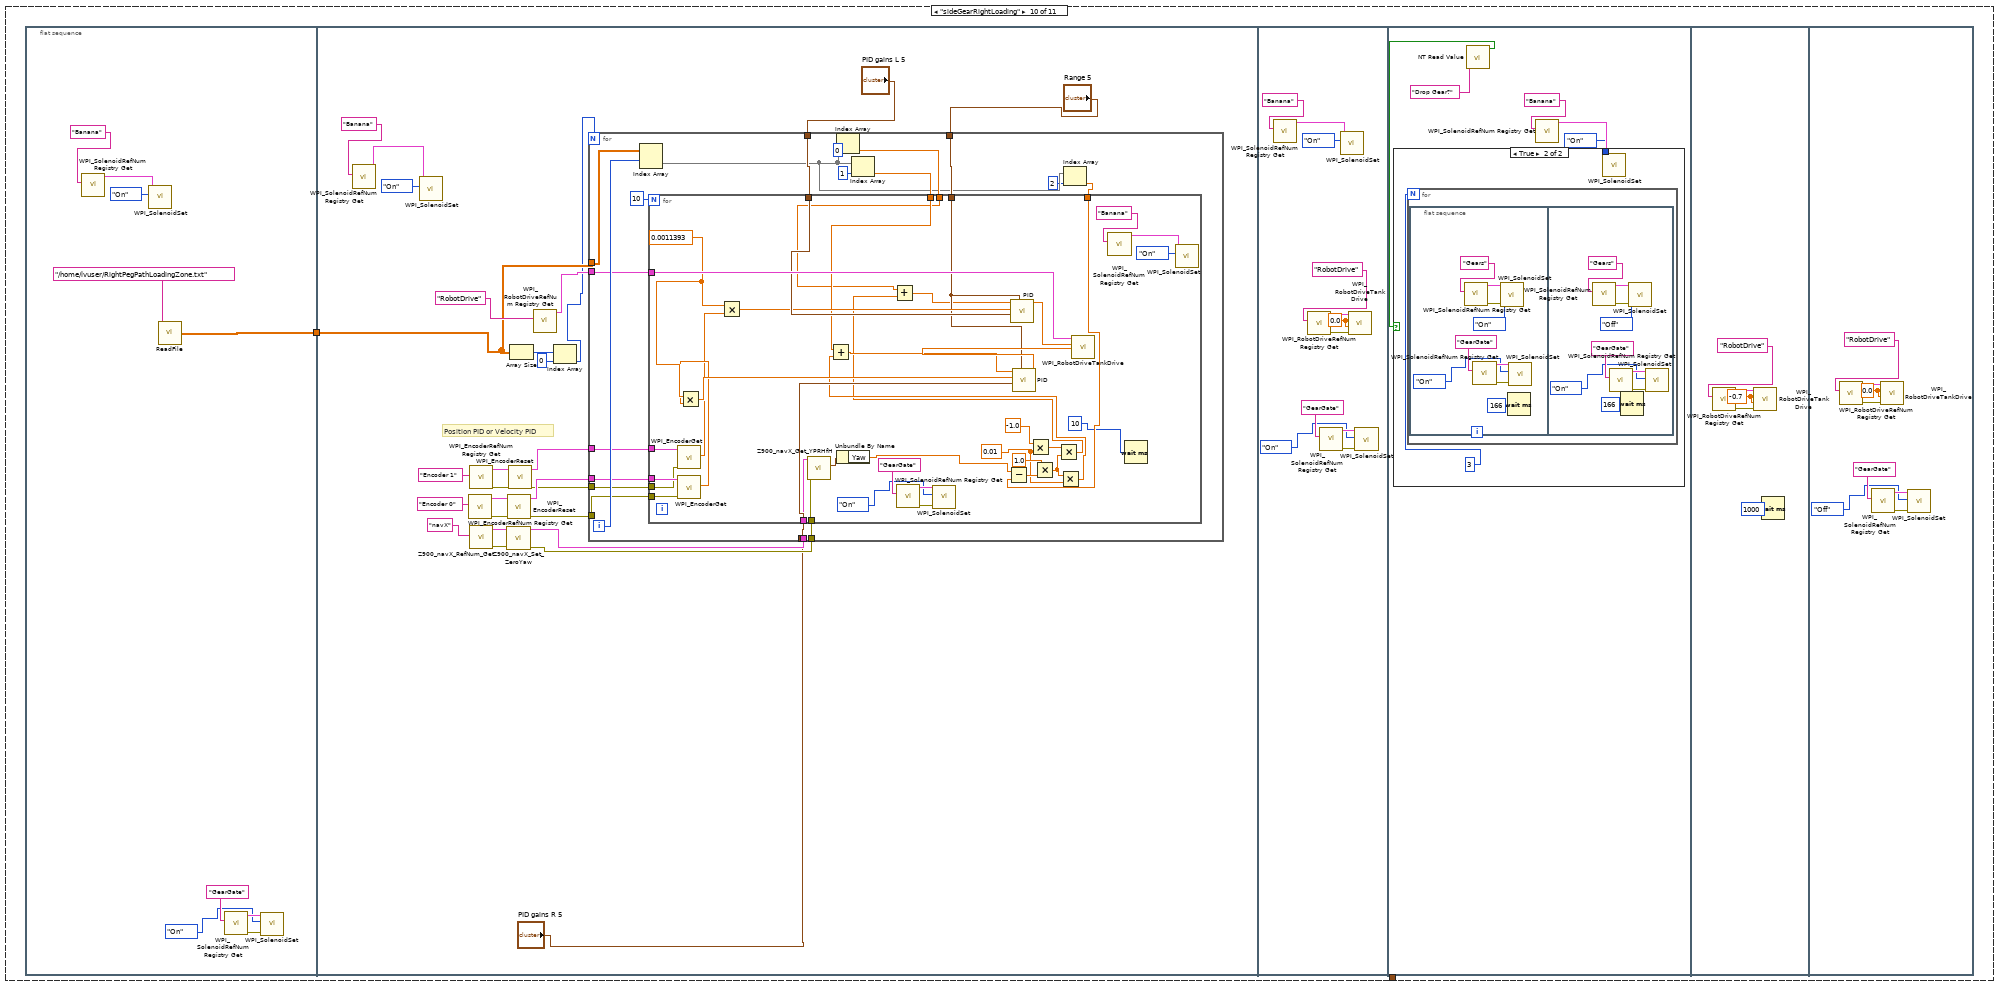
[diagram p18: hidden frame]
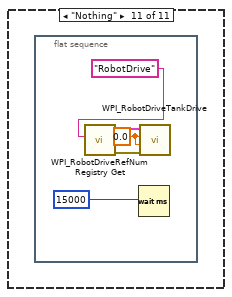
[diagram p20: hidden frame]
diagram:
  (unwired) "This function is run in parallel when the autonomous period begins. It will be terminated automatically when the period ends.\n\nNote that all Driver Station inputs are automatically latched and will not change once auto begins."
  # "This tells you the autonomous selected\nfrom the dashboard"
  # "Every 20ms, report that we are running autonomous\ncode. Loop will abort the same time as the VI."
  # "This gives you the joystick value\nthat is often the throttle"
  # "Use time and/or sensors to control how the robot drives."
  # "This tells you the driver position\nand alliance color"
  n1 = while {
    stop <- FALSE stop-if-true
    n2 = call <vilib>:"WPI_DriverStationReport Robot Code State.vi"("Autonomous"=TRUE) -> ()  [unwired: 10 in, 1 out]
    n3 = Wait (ms)(milliseconds to wait=u32 20) -> ()  [unwired: 1 out]
  }
  n4 = call <vilib>:"WPI_DriverStationGet Alliance Info.vi"() -> ()  [unwired: 12 out]
  n5 = call-poly <vilib>:"NT Read Value.vi"("Name"="Auto Selector") -> ("String"=w21:string)  [unwired: 9 in, 1 out]
  n6 = case shown="\"RightGear\", Default" w21 {
    tunnel: "Range" -> [_ w129 w433 _ _ w1050 _ _ _ _ _]
    tunnel: "PID gains L" -> [_ w128 w432 _ _ w1049 _ _ _ _ _]
    tunnel: "Speed 2" -> [_ w127 w431 _ _ w1048 _ _ _ _ _]
    tunnel: "Center" -> [_ _ _ _ _ _ _ _ _ _ _]
    tunnel: "MOE" -> [_ _ _ _ _ _ _ _ _ _ _]
    tunnel: "Speed" -> [_ w124 w428 _ _ w1045 _ _ _ _ _]
    tunnel: "Center" -> [_ _ _ _ _ _ _ _ _ _ _]
    tunnel: "MOE" -> [_ _ _ _ _ _ _ _ _ _ _]
    tunnel: "Center" -> [_ w126 w430 _ _ w1047 _ _ _ _ _]
    tunnel: "MOE" -> [_ w125 w429 _ _ w1046 _ _ _ _ _]
    tunnel: "PID gains R" -> [_ w123 w427 _ _ w1044 _ _ _ _ _]
    tunnel: "Speed 2" -> [_ _ _ _ _ _ _ _ _ _ _]
    tunnel: "MOE" -> [_ _ _ _ _ _ _ _ _ _ _]
    tunnel: "RightPID" -> [_ _ _ _ _ _ _ _ _ _ _]
    tunnel: "HopperSpeed" -> [_ w118 w422 _ _ _ _ _ _ _ _]
    tunnel: "HI" -> [_ w117 w421 _ _ _ _ _ _ _ _]
    tunnel: "HP" -> [_ w116 w420 _ _ _ _ _ _ _ _]
    tunnel: "HI" -> [_ w115 w419 _ _ _ _ _ _ _ _]
    tunnel: "HP" -> [_ w114 w418 _ _ _ _ _ _ _ _]
    tunnel: "HopperSpeed" -> [_ w113 w417 _ _ _ _ _ _ _ _]
    tunnel: "HP" -> [_ w112 w416 _ _ _ _ _ _ _ _]
    tunnel: "HI" -> [_ w111 w415 _ _ _ _ _ _ _ _]
    tunnel: "HopperSpeed" -> [_ w110 w414 _ _ _ _ _ _ _ _]
    tunnel: "SP" -> [w33 _ _ _ _ _ _ _ _ _ _]
    tunnel: "SI" -> [w32 _ _ _ _ _ _ _ _ _ _]
    tunnel: "ShootSpeed" -> [w31 _ _ _ _ _ _ _ _ _ _]
    tunnel: "ShootSpeed" -> [w30 _ _ _ _ _ _ _ _ _ _]
    tunnel: "SI" -> [w29 _ _ _ _ _ _ _ _ _ _]
    tunnel: "SP" -> [w28 _ _ _ _ _ _ _ _ _ _]
    tunnel: "sizone" -> [w27 _ _ _ _ _ _ _ _ _ _]
    tunnel: "sizone" -> [w26 _ _ _ _ _ _ _ _ _ _]
    tunnel: "Hizone" -> [_ w109 w413 _ _ _ _ _ _ _ _]
    tunnel: "Hizone" -> [_ w108 w412 _ _ _ _ _ _ _ _]
    tunnel: "HopperSpeed" -> [_ w107 w411 _ _ _ _ _ _ _ _]
    tunnel: "HP" -> [_ w106 w410 _ _ _ _ _ _ _ _]
    tunnel: "HI" -> [_ w105 w409 _ _ _ _ _ _ _ _]
    tunnel: "Hizone" -> [_ w104 w408 _ _ _ _ _ _ _ _]
    tunnel: "Hizone" -> [_ w103 w407 _ _ _ _ _ _ _ _]
    tunnel: "Hizone" -> [_ w102 w406 _ _ _ _ _ _ _ _]
    tunnel: "FrontSpeed" -> [_ _ _ _ _ w1043 _ _ _ _ _]
    tunnel: "FP" -> [_ _ _ _ _ w1042 _ _ _ _ _]
    tunnel: "FI" -> [_ _ _ _ _ w1041 _ _ _ _ _]
    tunnel: "Fizone" -> [_ _ _ _ _ w1040 _ _ _ _ _]
    tunnel: "FrontSpeed" -> [_ _ _ _ _ w1039 _ _ _ _ _]
    tunnel: "FP" -> [_ _ _ _ _ w1038 _ _ _ _ _]
    tunnel: "FI" -> [_ _ _ _ _ w1037 _ _ _ _ _]
    tunnel: "Fizone" -> [_ _ _ _ _ w1036 _ _ _ _ _]
    tunnel: "FrontSpeed" -> [_ _ _ _ _ w1035 _ _ _ _ _]
    tunnel: "FP" -> [_ _ _ _ _ w1034 _ _ _ _ _]
    tunnel: "FI" -> [_ _ _ _ _ w1033 _ _ _ _ _]
    tunnel: "Fizone" -> [_ _ _ _ _ w1032 _ _ _ _ _]
    frame "just shoot" {
      n7 = flat-sequence {
        tunnel: w30 -> [w41]
        tunnel: w29 -> [w40]
        tunnel: w28 -> [w39]
        tunnel: w27 -> [w38]
        tunnel: w33 -> [w58]
        tunnel: w32 -> [w57]
        tunnel: w31 -> [w56]
        tunnel: w26 -> [w55]
        frame #0 {
          n8 = call <vilib>:"WPI_RobotDriveRefNum Registry Get.vi"("refnum name"="RobotDrive") -> ("error out"=w46:errorcluster, "RobotDriveDevRef"=w45:T5)  [unwired: 9 in]
          n9 = call <vilib>:"WPI_SolenoidRefNum Registry Get.vi"("refnum name"="HopperHitter") -> ("error out"=w35:errorcluster, "SolenoidDevRef"=w36:T10)  [unwired: 9 in]
          n10 = call <vilib>:"WPI_RobotDriveTankDrive.vi"("error in (no error)"=w46, "Right axis value"=0.0, "Left axis value"=0.0, "RobotDriveDevRef"=w45) -> ()  [unwired: 5 in, 3 out]
          n11 = call <vilib>:"WPI_MotorControlRefNum Registry Get.vi"("refnum name"="Shooter" ("Name")) -> ("error out"=w42:errorcluster, "MotorControlDevRef"=w43:T6)  [unwired: 9 in]
          n12 = call-poly <vilib>:"WPI_SolenoidSet.vi"("error in (no error)"=w35, "Value"=WPI_SolenoidValue."On", "SolenoidDevRef"=w36) -> ()  [unwired: 7 in, 2 out]
          n13 = Wait (ms)(milliseconds to wait=4000) -> ()  [unwired: 1 out]
          n14 = call "TalonPID.vi"("P"=w39, "Ref In"=w43, "Error in"=w42, "I"=w40, "I Zone"=w38, "Output"=w41) -> ()  [unwired: 8 in, 2 out]
        }
        frame #1 {
          n15 = call <vilib>:"WPI_SolenoidRefNum Registry Get.vi"("refnum name"="HopperHitter") -> ("error out"=w52:errorcluster, "SolenoidDevRef"=w53:T10)  [unwired: 9 in]
          n16 = call-poly <vilib>:"WPI_SolenoidSet.vi"("error in (no error)"=w52, "Value"=WPI_SolenoidValue."On", "SolenoidDevRef"=w53) -> ()  [unwired: 7 in, 2 out]
          n17 = call <vilib>:"WPI_MotorControlRefNum Registry Get.vi"("refnum name"="Shooter" ("Name")) -> ("error out"=w75:errorcluster, "MotorControlDevRef"=w76:T6)  [unwired: 9 in]
          n18 = call "TalonPID.vi"("P"=w58, "Ref In"=w76, "Error in"=w75, "I"=w57, "I Zone"=w55, "Output"=w56) -> ()  [unwired: 8 in, 2 out]
          n19 = Multiply(x=0.9, y=-1.0) -> (x*y=w72:dbl)
          n20 = call <vilib>:"WPI_RobotDriveRefNum Registry Get.vi"("refnum name"="RobotDrive") -> ("error out"=w60:errorcluster, "RobotDriveDevRef"=w59:T5)  [unwired: 9 in]
          n21 = Wait (ms)(milliseconds to wait=10500) -> ()  [unwired: 1 out]
          n22 = call <vilib>:"WPI_RobotDriveTankDrive.vi"("error in (no error)"=w60, "Right axis value"=0.0, "Left axis value"=0.0, "RobotDriveDevRef"=w59) -> ()  [unwired: 5 in, 3 out]
          n23 = call <vilib>:"WPI_MotorControlRefNum Registry Get.vi"("refnum name"="Feeder") -> ("error out"=w70:errorcluster, "MotorControlDevRef"=w69:T6)  [unwired: 9 in]
          n24 = call <vilib>:"WPI_MotorControlRefNum Registry Get.vi"("refnum name"="Shuriken") -> ("error out"=w68:errorcluster, "MotorControlDevRef"=w67:T6)  [unwired: 9 in]
          n25 = call <vilib>:"WPI_MotorControlSetOutput.vi"("error in (no error)"=w70, "Output"=w72, "MotorControlDevRef"=w69) -> ()  [unwired: 6 in, 3 out]
          n26 = call <vilib>:"WPI_MotorControlSetOutput.vi"("error in (no error)"=w68, "Output"=0.2, "MotorControlDevRef"=w67) -> ()  [unwired: 6 in, 3 out]
        }
        frame #2 {
          n27 = call <vilib>:"WPI_SolenoidRefNum Registry Get.vi"("refnum name"="HopperHitter") -> ("error out"=w80:errorcluster, "SolenoidDevRef"=w81:T10)  [unwired: 9 in]
          n28 = call-poly <vilib>:"WPI_SolenoidSet.vi"("error in (no error)"=w80, "Value"=WPI_SolenoidValue."On", "SolenoidDevRef"=w81) -> ()  [unwired: 7 in, 2 out]
          n29 = Multiply(x=0.0, y=-1.0) -> (x*y=w99:dbl)
          n30 = Wait (ms)(milliseconds to wait=500) -> ()  [unwired: 1 out]
          n31 = call <vilib>:"WPI_MotorControlRefNum Registry Get.vi"("refnum name"="Feeder") -> ("error out"=w97:errorcluster, "MotorControlDevRef"=w96:T6)  [unwired: 9 in]
          n32 = call <vilib>:"WPI_MotorControlRefNum Registry Get.vi"("refnum name"="Shuriken") -> ("error out"=w95:errorcluster, "MotorControlDevRef"=w94:T6)  [unwired: 9 in]
          n33 = call <vilib>:"WPI_MotorControlRefNum Registry Get.vi"("refnum name"="Shooter") -> ("MotorControlDevRef"=w90:T6)  [unwired: 9 in, 1 out]
          n34 = call <vilib>:"WPI_RobotDriveRefNum Registry Get.vi"("refnum name"="RobotDrive") -> ("error out"=w85:errorcluster, "RobotDriveDevRef"=w84:T5)  [unwired: 9 in]
          n35 = call <vilib>:"WPI_MotorControlSetOutput.vi"("error in (no error)"=w97, "Output"=w99, "MotorControlDevRef"=w96) -> ()  [unwired: 6 in, 3 out]
          n36 = call <vilib>:"WPI_MotorControlSetOutput.vi"("error in (no error)"=w95, "Output"=0.0, "MotorControlDevRef"=w94) -> ()  [unwired: 6 in, 3 out]
          n37 = call <vilib>:"WPI_RobotDriveTankDrive.vi"("error in (no error)"=w85, "Right axis value"=0.0, "Left axis value"=0.0, "RobotDriveDevRef"=w84) -> ()  [unwired: 5 in, 3 out]
          n38 = call <vilib>:"WPI_CANTalonSRX_ChangeMode.vi"("Output"=0.0, "Control Mode"=WPI_CANTalonSRX_APIControlMode."Percent VBus", "CAN Talon SRX Ref"=w90) -> ()  [unwired: 7 in, 2 out]
        }
      }
    }
    frame "HopperLeft" {
      n39 = flat-sequence {
        tunnel: w115 -> [w137]
        tunnel: w114 -> [w136]
        tunnel: w113 -> [w135]
        tunnel: w108 -> [w134]
        tunnel: w129 -> [_]
        tunnel: w128 -> [_]
        tunnel: w124 -> [_]
        tunnel: w123 -> [_]
        tunnel: [w159] -> w119
        tunnel: w118 -> [w158]
        tunnel: w117 -> [w157]
        tunnel: w116 -> [w156]
        tunnel: w109 -> [w155]
        tunnel: [w237] -> w120
        tunnel: w119 -> [w237]
        tunnel: w127 -> [_]
        tunnel: w126 -> [_]
        tunnel: w125 -> [_]
        tunnel: [w256] -> w121
        tunnel: w120 -> [w256]
        tunnel: w107 -> [w253]
        tunnel: w106 -> [w252]
        tunnel: w105 -> [w251]
        tunnel: w104 -> [w250]
        tunnel: [w282] -> w122
        tunnel: w121 -> [w282]
        tunnel: w122 -> [w302]
        tunnel: w112 -> [w298]
        tunnel: w111 -> [w297]
        tunnel: w110 -> [w296]
        tunnel: w102 -> [w295]
        tunnel: w112 -> [w364]
        tunnel: w111 -> [w363]
        tunnel: w110 -> [w362]
        tunnel: [w361] -> _
        tunnel: w103 -> [w361]
        frame #0 {
          n40 = call <vilib>:"WPI_MotorControlRefNum Registry Get.vi"("refnum name"="Shooter" ("Name")) -> ("error out"=w141:errorcluster, "MotorControlDevRef"=w142:T6)  [unwired: 9 in]
          n41 = call <vilib>:"WPI_SolenoidRefNum Registry Get.vi"("refnum name"="Banana") -> ("SolenoidDevRef"=w146:T10)  [unwired: 9 in, 1 out]
          n42 = call-poly <vilib>:"WPI_SolenoidSet.vi"("Value"=WPI_SolenoidValue."On", "SolenoidDevRef"=w146) -> ()  [unwired: 8 in, 2 out]
          n43 = call "TalonPID.vi"("P"=w136, "Ref In"=w142, "Error in"=w141, "I"=w137, "I Zone"=w134, "Output"=w135) -> ()  [unwired: 8 in, 2 out]
          n44 = call <vilib>:"WPI_SolenoidRefNum Registry Get.vi"("refnum name"="GearGate") -> ("error out"=w150:errorcluster, "SolenoidDevRef"=w149:T10)  [unwired: 9 in]
          n45 = call-poly <vilib>:"WPI_SolenoidSet.vi"("error in (no error)"=w150, "Value"=WPI_SolenoidValue."On", "SolenoidDevRef"=w149) -> ()  [unwired: 7 in, 2 out]
          n46 = call "Z900_navX_RefNum_Get.vi"("refnum name"="navX") -> ("error out"=w139:errorcluster, "navX Device"=w140:T12)  [unwired: 9 in]
          n47 = call <vilib>:"WPI_SolenoidRefNum Registry Get.vi"("refnum name"="HopperHitter") -> ("error out"=w131:errorcluster, "SolenoidDevRef"=w132:T10)  [unwired: 9 in]
          n48 = call "Z900_navX_Set_ZeroYaw.vi"("error in (no error)"=w139, "navX Device"=w140) -> ()  [unwired: 8 in, 2 out]
          n49 = call-poly <vilib>:"WPI_SolenoidSet.vi"("error in (no error)"=w131, "Value"=WPI_SolenoidValue."On", "SolenoidDevRef"=w132) -> ()  [unwired: 7 in, 2 out]
        }
        frame #1 {
          n50 = call <vilib>:"WPI_SolenoidRefNum Registry Get.vi"("refnum name"="HopperHitter") -> ("error out"=w152:errorcluster, "SolenoidDevRef"=w153:T10)  [unwired: 9 in]
          n51 = call <vilib>:"WPI_EncoderRefNum Registry Get.vi"("refnum name"="Encoder 1") -> ("error out"=w171:errorcluster, "EncoderDevRef"=w173:T14)  [unwired: 9 in]
          n52 = call <vilib>:"WPI_EncoderRefNum Registry Get.vi"("refnum name"="Encoder 0") -> ("error out"=w172:errorcluster, "EncoderDevRef"=w174:T14)  [unwired: 9 in]
          n53 = call <vilib>:"WPI_SolenoidRefNum Registry Get.vi"("refnum name"="GearGate") -> ("error out"=w170:errorcluster, "SolenoidDevRef"=w169:T10)  [unwired: 9 in]
          n54 = call-poly <vilib>:"NT Read Value.vi"("Default Value"=14.0, "Name"="Circumference") -> ("Numeric"=w160:dbl)  [unwired: 8 in, 1 out]
          n55 = call-poly <vilib>:"WPI_SolenoidSet.vi"("error in (no error)"=w170, "Value"=WPI_SolenoidValue."On", "SolenoidDevRef"=w169) -> ()  [unwired: 7 in, 2 out]
          n56 = call-poly <vilib>:"WPI_SolenoidSet.vi"("error in (no error)"=w152, "Value"=WPI_SolenoidValue."On", "SolenoidDevRef"=w153) -> ()  [unwired: 7 in, 2 out]
          n57 = call <vilib>:"WPI_EncoderReset.vi"("error in (no error)"=w172, "EncoderDevRef"=w174) -> ("error out"=w165:errorcluster, "EncoderDevRef"=w166:T14)  [unwired: 8 in]
          n58 = call <vilib>:"WPI_EncoderReset.vi"("error in (no error)"=w171, "EncoderDevRef"=w173) -> ("error out"=w163:errorcluster, "EncoderDevRef"=w164:T14)  [unwired: 8 in]
          n59 = while {
            tunnel: w166 -> [w211]
            tunnel: w165 -> [w210]
            tunnel: w164 -> [w209]
            tunnel: w163 -> [w208]
            tunnel: w160 -> [w193]
            tunnel: ["ForwardPID"] -> w159
            tunnel: w158 -> [w184]
            tunnel: w157 -> [w183]
            tunnel: w156 -> [w182]
            tunnel: w155 -> [w181]
            i -> [w198]
            stop <- w194 stop-if-true
            w192 = 0.65 ("x")
            n60 = call <vilib>:"WPI_EncoderGet.vi"("error in (no error)"=w210, "EncoderDevRef"=w211) -> ("Distance"=w207:dbl)  [unwired: 4 in, 5 out]
            n61 = call <vilib>:"WPI_EncoderGet.vi"("error in (no error)"=w208, "EncoderDevRef"=w209) -> ("Distance"=w206:dbl)  [unwired: 4 in, 5 out]
            n62 = Subtract(x=w207, y=w206) -> (x-y=w221:dbl)
            n63 = call "Z900_navX_RefNum_Get.vi"("refnum name"="navX") -> ("error out"=w186:errorcluster, "navX Device"=w187:T12)  [unwired: 9 in]
            n64 = call "Z900_navX_Set_ZeroYaw.vi"("error in (no error)"=w186, "navX Device"=w187) -> ()  [unwired: 8 in, 2 out]
            n65 = Add(x=w207, y=w206) -> (x+y=w205:dbl)
            n66 = call-poly <vilib>:"PID.vi"("output range"=cluster{"output high":dbl, "output low":dbl} {"output high"=0.5, "output low"=-0.5}, "PID gains"="ForwardPID", "process variable"=w221, "setpoint"=0.0) -> ("output"=w227:dbl)  [unwired: 6 in, 1 out]
            n67 = Divide(x=w205, y=2.0) -> (x/y=w200:dbl)
            n68 = Subtract(x=w192, y=w227) -> (x-y=w223:dbl)
            n69 = Add(x=w192, y=w227) -> (x+y=w222:dbl)
            n70 = call <vilib>:"WPI_RobotDriveRefNum Registry Get.vi"("refnum name"="RobotDrive") -> ("RobotDriveDevRef"=w229:T5)  [unwired: 9 in, 1 out]
            n71 = Greater?(x=w198, y=600) -> (0:w195:bool)
            n72 = Divide(x=72.0, y=w193) -> (x/y=w202:dbl)
            n73 = call <vilib>:"WPI_SolenoidRefNum Registry Get.vi"("refnum name"="GearGate") -> ("error out"=w218:errorcluster, "SolenoidDevRef"=w217:T10)  [unwired: 9 in]
            n74 = call <vilib>:"WPI_RobotDriveTankDrive.vi"("Right axis value"=w222, "Left axis value"=w223, "RobotDriveDevRef"=w229) -> ()  [unwired: 6 in, 3 out]
            n75 = Multiply(x=w202, y=1024.0) -> (x*y=w199:dbl)
            n76 = Greater Or Equal?(x=w200, y=w199) -> (x >= y?=w196:bool)
            n77 = call-poly <vilib>:"WPI_SolenoidSet.vi"("error in (no error)"=w218, "Value"=WPI_SolenoidValue."On", "SolenoidDevRef"=w217) -> ()  [unwired: 7 in, 2 out]
            n78 = Or(x=w196, y=w195) -> (x .or. y?=w194:bool)
            n79 = Build Array(w223, w222, w221) -> (w219:dbl[])
            n80 = Array To Cluster(array=w219) -> (cluster=→"DriveStraight":T1)
            n81 = call <vilib>:"WPI_MotorControlRefNum Registry Get.vi"("refnum name"="Shooter" ("Name")) -> ("error out"=w188:errorcluster, "MotorControlDevRef"=w189:T6)  [unwired: 9 in]
            n82 = call <vilib>:"WPI_SolenoidRefNum Registry Get.vi"("refnum name"="Banana") -> ("SolenoidDevRef"=w214:T10)  [unwired: 9 in, 1 out]
            n83 = call <vilib>:"WPI_SolenoidRefNum Registry Get.vi"("refnum name"="HopperHitter") -> ("error out"=w178:errorcluster, "SolenoidDevRef"=w179:T10)  [unwired: 9 in]
            n84 = call-poly <vilib>:"WPI_SolenoidSet.vi"("Value"=WPI_SolenoidValue."On", "SolenoidDevRef"=w214) -> ()  [unwired: 8 in, 2 out]
            n85 = call "TalonPID.vi"("P"=w182, "Ref In"=w189, "Error in"=w188, "I"=w183, "I Zone"=w181, "Output"=w184) -> ()  [unwired: 8 in, 2 out]
            n86 = call-poly <vilib>:"WPI_SolenoidSet.vi"("error in (no error)"=w178, "Value"=WPI_SolenoidValue."On", "SolenoidDevRef"=w179) -> ()  [unwired: 7 in, 2 out]
            n87 = Wait (ms)(milliseconds to wait=10) -> ()  [unwired: 1 out]
          }
        }
        frame #2 {
          w244 = 0.0 ("Right axis value")
          n88 = call <vilib>:"WPI_SolenoidRefNum Registry Get.vi"("refnum name"="HopperHitter") -> ("error out"=w231:errorcluster, "SolenoidDevRef"=w232:T10)  [unwired: 9 in]
          n89 = Wait (ms)(milliseconds to wait=500) -> ()  [unwired: 1 out]
          n90 = call <vilib>:"WPI_RobotDriveRefNum Registry Get.vi"("refnum name"="RobotDrive") -> ("RobotDriveDevRef"=w245:T5)  [unwired: 9 in, 1 out]
          n91 = call <vilib>:"WPI_SolenoidRefNum Registry Get.vi"("refnum name"="GearGate") -> ("error out"=w242:errorcluster, "SolenoidDevRef"=w241:T10)  [unwired: 9 in]
          n92 = call "Z900_navX_RefNum_Get.vi"("refnum name"="navX") -> ("error out"=w235:errorcluster, "navX Device"=w236:T12)  [unwired: 9 in]
          n93 = call-poly <vilib>:"WPI_SolenoidSet.vi"("error in (no error)"=w231, "Value"=WPI_SolenoidValue."On", "SolenoidDevRef"=w232) -> ()  [unwired: 7 in, 2 out]
          n94 = call <vilib>:"WPI_RobotDriveTankDrive.vi"("Right axis value"=w244, "Left axis value"=w244, "RobotDriveDevRef"=w245) -> ()  [unwired: 6 in, 3 out]
          n95 = call "Z900_navX_Set_ZeroYaw.vi"("error in (no error)"=w235, "navX Device"=w236) -> ()  [unwired: 8 in, 2 out]
          n96 = call-poly <vilib>:"WPI_SolenoidSet.vi"("error in (no error)"=w242, "Value"=WPI_SolenoidValue."On", "SolenoidDevRef"=w241) -> ()  [unwired: 7 in, 2 out]
        }
        frame #3 {
          n97 = call <vilib>:"WPI_SolenoidRefNum Registry Get.vi"("refnum name"="HopperHitter") -> ("error out"=w247:errorcluster, "SolenoidDevRef"=w248:T10)  [unwired: 9 in]
          n98 = call "Z900_navX_RefNum_Get.vi"("refnum name"="navX") -> ("error out"=w258:errorcluster, "navX Device"=w259:T12)  [unwired: 9 in]
          n99 = call "Z900_navX_Set_ZeroYaw.vi"("error in (no error)"=w258, "navX Device"=w259) -> ("error out"=w254:errorcluster, "navX Device"=w255:T12)  [unwired: 8 in]
          n100 = call-poly <vilib>:"WPI_SolenoidSet.vi"("error in (no error)"=w247, "Value"=WPI_SolenoidValue."On", "SolenoidDevRef"=w248) -> ()  [unwired: 7 in, 2 out]
          n101 = while {
            tunnel: w255 -> [w265]
            tunnel: w254 -> [w264]
            tunnel: w253 -> [w263]
            tunnel: w252 -> [w262]
            tunnel: w251 -> [w261]
            tunnel: w250 -> [w260]
            stop <- w266 stop-if-true
            w272 = -0.55 ("Right axis value")
            n102 = call "Z900_navX_Get_YPRHfH.vi"("error in (no error)"=w264, "navX Device"=w265) -> ("YRPHfH"=w268:T18)  [unwired: 6 in, 3 out]
            n103 = Unbundle By Name(w268) -> ("Yaw"=w267:dbl)
            n104 = call <vilib>:"WPI_MotorControlRefNum Registry Get.vi"("refnum name"="Shooter" ("Name")) -> ("error out"=w269:errorcluster, "MotorControlDevRef"=w270:T6)  [unwired: 9 in]
            n105 = call <vilib>:"WPI_RobotDriveRefNum Registry Get.vi"("refnum name"="RobotDrive") -> ("RobotDriveDevRef"=w276:T5)  [unwired: 9 in, 1 out]
            n106 = Multiply(x=-1.0, y=w272) -> (x*y=w273:dbl)
            n107 = call <vilib>:"WPI_RobotDriveTankDrive.vi"("Right axis value"=w273, "Left axis value"=w272, "RobotDriveDevRef"=w276) -> ()  [unwired: 6 in, 3 out]
            n108 = call "TalonPID.vi"("P"=w262, "Ref In"=w270, "Error in"=w269, "I"=w261, "I Zone"=w260, "Output"=w263) -> ()  [unwired: 8 in, 2 out]
            n109 = Greater?(x=w267, y=85.0) -> (0:w266:bool)
          }
        }
        frame #4 {
          w288 = 0.0 ("Left axis value")
          n110 = call <vilib>:"WPI_SolenoidRefNum Registry Get.vi"("refnum name"="HopperHitter") -> ("error out"=w279:errorcluster, "SolenoidDevRef"=w280:T10)  [unwired: 9 in]
          n111 = call <vilib>:"WPI_RobotDriveRefNum Registry Get.vi"("refnum name"="RobotDrive") -> ("error out"=w289:errorcluster, "RobotDriveDevRef"=w290:T5)  [unwired: 9 in]
          n112 = call <vilib>:"WPI_SolenoidRefNum Registry Get.vi"("refnum name"="GearGate") -> ("error out"=w286:errorcluster, "SolenoidDevRef"=w285:T10)  [unwired: 9 in]
          n113 = call <vilib>:"WPI_RobotDriveTankDrive.vi"("error in (no error)"=w289, "Right axis value"=w288, "Left axis value"=w288, "RobotDriveDevRef"=w290) -> ()  [unwired: 5 in, 3 out]
          n114 = call-poly <vilib>:"WPI_SolenoidSet.vi"("error in (no error)"=w279, "Value"=WPI_SolenoidValue."On", "SolenoidDevRef"=w280) -> ()  [unwired: 7 in, 2 out]
          n115 = call-poly <vilib>:"WPI_SolenoidSet.vi"("error in (no error)"=w286, "Value"=WPI_SolenoidValue."On", "SolenoidDevRef"=w285) -> ()  [unwired: 7 in, 2 out]
        }
        frame #5 {
          n116 = call <vilib>:"WPI_SolenoidRefNum Registry Get.vi"("refnum name"="HopperHitter") -> ("error out"=w292:errorcluster, "SolenoidDevRef"=w293:T10)  [unwired: 9 in]
          n117 = call <vilib>:"WPI_EncoderRefNum Registry Get.vi"("refnum name"="Encoder 1") -> ("error out"=w311:errorcluster, "EncoderDevRef"=w313:T14)  [unwired: 9 in]
          n118 = call <vilib>:"WPI_EncoderRefNum Registry Get.vi"("refnum name"="Encoder 0") -> ("error out"=w312:errorcluster, "EncoderDevRef"=w314:T14)  [unwired: 9 in]
          n119 = call <vilib>:"WPI_SolenoidRefNum Registry Get.vi"("refnum name"="GearGate") -> ("error out"=w310:errorcluster, "SolenoidDevRef"=w309:T10)  [unwired: 9 in]
          n120 = call-poly <vilib>:"WPI_SolenoidSet.vi"("error in (no error)"=w292, "Value"=WPI_SolenoidValue."On", "SolenoidDevRef"=w293) -> ()  [unwired: 7 in, 2 out]
          n121 = call-poly <vilib>:"WPI_SolenoidSet.vi"("error in (no error)"=w310, "Value"=WPI_SolenoidValue."On", "SolenoidDevRef"=w309) -> ()  [unwired: 7 in, 2 out]
          n122 = call "Z900_navX_RefNum_Get.vi"("refnum name"="navX") -> ("error out"=w300:errorcluster, "navX Device"=w301:T12)  [unwired: 9 in]
          n123 = call <vilib>:"WPI_EncoderReset.vi"("error in (no error)"=w312, "EncoderDevRef"=w314) -> ("error out"=w305:errorcluster, "EncoderDevRef"=w306:T14)  [unwired: 8 in]
          n124 = call <vilib>:"WPI_EncoderReset.vi"("error in (no error)"=w311, "EncoderDevRef"=w313) -> ("error out"=w303:errorcluster, "EncoderDevRef"=w304:T14)  [unwired: 8 in]
          n125 = call "Z900_navX_Set_ZeroYaw.vi"("error in (no error)"=w300, "navX Device"=w301) -> ()  [unwired: 8 in, 2 out]
          n126 = while {
            tunnel: w306 -> [w338]
            tunnel: w305 -> [w337]
            tunnel: w304 -> [w336]
            tunnel: w303 -> [w335]
            tunnel: w302 -> [w329]
            tunnel: w298 -> [w324]
            tunnel: w297 -> [w323]
            tunnel: w296 -> [w322]
            tunnel: w295 -> [w321]
            i -> [w332]
            stop <- w325 stop-if-true
            w330 = -0.65 ("x")
            n127 = call <vilib>:"WPI_EncoderGet.vi"("error in (no error)"=w337, "EncoderDevRef"=w338) -> ("Distance"=w334:dbl)  [unwired: 4 in, 5 out]
            n128 = call <vilib>:"WPI_EncoderGet.vi"("error in (no error)"=w335, "EncoderDevRef"=w336) -> ("Distance"=w333:dbl)  [unwired: 4 in, 5 out]
            n129 = Subtract(x=w334, y=w333) -> (x-y=w348:dbl)
            n130 = call-poly <vilib>:"PID.vi"("output range"=cluster{"output high":dbl, "output low":dbl} {"output high"=0.5, "output low"=-0.5}, "PID gains"=w329, "process variable"=w348, "setpoint"=0.0) -> ("output"=w354:dbl)  [unwired: 6 in, 1 out]
            n131 = call <vilib>:"WPI_SolenoidRefNum Registry Get.vi"("refnum name"="HopperHitter") -> ("error out"=w318:errorcluster, "SolenoidDevRef"=w319:T10)  [unwired: 9 in]
            n132 = Subtract(x=w330, y=w354) -> (x-y=w350:dbl)
            n133 = Add(x=w330, y=w354) -> (x+y=w349:dbl)
            n134 = call <vilib>:"WPI_RobotDriveRefNum Registry Get.vi"("refnum name"="RobotDrive") -> ("RobotDriveDevRef"=w356:T5)  [unwired: 9 in, 1 out]
            n135 = call-poly <vilib>:"WPI_SolenoidSet.vi"("error in (no error)"=w318, "Value"=WPI_SolenoidValue."On", "SolenoidDevRef"=w319) -> ()  [unwired: 7 in, 2 out]
            n136 = Greater?(x=w332, y=75) -> (0:w325:bool)
            n137 = call <vilib>:"WPI_SolenoidRefNum Registry Get.vi"("refnum name"="GearGate") -> ("error out"=w345:errorcluster, "SolenoidDevRef"=w344:T10)  [unwired: 9 in]
            n138 = call <vilib>:"WPI_RobotDriveTankDrive.vi"("Right axis value"=w349, "Left axis value"=w350, "RobotDriveDevRef"=w356) -> ()  [unwired: 6 in, 3 out]
            n139 = call-poly <vilib>:"WPI_SolenoidSet.vi"("error in (no error)"=w345, "Value"=WPI_SolenoidValue."On", "SolenoidDevRef"=w344) -> ()  [unwired: 7 in, 2 out]
            n140 = Build Array(w350, w349, w348) -> (w346:dbl[])
            n141 = Array To Cluster(array=w346) -> (cluster=→"DriveStraight 3":T1)
            n142 = call <vilib>:"WPI_MotorControlRefNum Registry Get.vi"("refnum name"="Shooter" ("Name")) -> ("error out"=w326:errorcluster, "MotorControlDevRef"=w327:T6)  [unwired: 9 in]
            n143 = call <vilib>:"WPI_SolenoidRefNum Registry Get.vi"("refnum name"="Banana") -> ("SolenoidDevRef"=w341:T10)  [unwired: 9 in, 1 out]
            n144 = call-poly <vilib>:"WPI_SolenoidSet.vi"("Value"=WPI_SolenoidValue."On", "SolenoidDevRef"=w341) -> ()  [unwired: 8 in, 2 out]
            n145 = call "TalonPID.vi"("P"=w324, "Ref In"=w327, "Error in"=w326, "I"=w323, "I Zone"=w321, "Output"=w322) -> ()  [unwired: 8 in, 2 out]
            n146 = Wait (ms)(milliseconds to wait=10) -> ()  [unwired: 1 out]
          }
        }
        frame #6 {
          (unwired) 0.0 ("Right axis value")
          n147 = call <vilib>:"WPI_SolenoidRefNum Registry Get.vi"("refnum name"="HopperHitter") -> ("error out"=w358:errorcluster, "SolenoidDevRef"=w359:T10)  [unwired: 9 in]
          n148 = call <vilib>:"WPI_MotorControlRefNum Registry Get.vi"("refnum name"="Shooter" ("Name")) -> ("error out"=w365:errorcluster, "MotorControlDevRef"=w366:T6)  [unwired: 9 in]
          n149 = call-poly <vilib>:"WPI_SolenoidSet.vi"("error in (no error)"=w358, "Value"=WPI_SolenoidValue."On", "SolenoidDevRef"=w359) -> ()  [unwired: 7 in, 2 out]
          n150 = call "TalonPID.vi"("P"=w364, "Ref In"=w366, "Error in"=w365, "I"=w363, "I Zone"=w361, "Output"=w362) -> ()  [unwired: 8 in, 2 out]
          n151 = Multiply(x=0.9, y=-1.0) -> (x*y=w379:dbl)
          n152 = call <vilib>:"WPI_RobotDriveRefNum Registry Get.vi"("refnum name"="RobotDrive") -> ("error out"=w369:errorcluster, "RobotDriveDevRef"=w368:T5)  [unwired: 9 in]
          n153 = call <vilib>:"WPI_MotorControlRefNum Registry Get.vi"("refnum name"="Feeder") -> ("error out"=w377:errorcluster, "MotorControlDevRef"=w376:T6)  [unwired: 9 in]
          n154 = call <vilib>:"WPI_MotorControlRefNum Registry Get.vi"("refnum name"="Shuriken") -> ("error out"=w375:errorcluster, "MotorControlDevRef"=w374:T6)  [unwired: 9 in]
          n155 = call <vilib>:"WPI_RobotDriveTankDrive.vi"("error in (no error)"=w369, "Left axis value"=0.0, "RobotDriveDevRef"=w368) -> ()  [unwired: 6 in, 3 out]
          n156 = call <vilib>:"WPI_MotorControlSetOutput.vi"("error in (no error)"=w377, "Output"=w379, "MotorControlDevRef"=w376) -> ()  [unwired: 6 in, 3 out]
          n157 = call <vilib>:"WPI_MotorControlSetOutput.vi"("error in (no error)"=w375, "Output"=0.5, "MotorControlDevRef"=w374) -> ()  [unwired: 6 in, 3 out]
          n158 = Wait (ms)(milliseconds to wait=9000) -> ()  [unwired: 1 out]
        }
        frame #7 {
          n159 = call <vilib>:"WPI_MotorControlRefNum Registry Get.vi"("refnum name"="Shooter") -> ("MotorControlDevRef"=w404:T6)  [unwired: 9 in, 1 out]
          n160 = call <vilib>:"WPI_RobotDriveRefNum Registry Get.vi"("refnum name"="RobotDrive") -> ("error out"=w389:errorcluster, "RobotDriveDevRef"=w388:T5)  [unwired: 9 in]
          n161 = call <vilib>:"WPI_SolenoidRefNum Registry Get.vi"("refnum name"="HopperHitter") -> ("error out"=w385:errorcluster, "SolenoidDevRef"=w386:T10)  [unwired: 9 in]
          n162 = Multiply(x=0.0, y=-1.0) -> (x*y=w395:dbl)
          n163 = call <vilib>:"WPI_RobotDriveTankDrive.vi"("error in (no error)"=w389, "Right axis value"=0.0, "Left axis value"=0.0, "RobotDriveDevRef"=w388) -> ()  [unwired: 5 in, 3 out]
          n164 = call <vilib>:"WPI_CANTalonSRX_ChangeMode.vi"("Output"=0.0, "Control Mode"=WPI_CANTalonSRX_APIControlMode."Percent VBus", "CAN Talon SRX Ref"=w404) -> ()  [unwired: 7 in, 2 out]
          n165 = call-poly <vilib>:"WPI_SolenoidSet.vi"("error in (no error)"=w385, "Value"=WPI_SolenoidValue."On", "SolenoidDevRef"=w386) -> ()  [unwired: 7 in, 2 out]
          n166 = call <vilib>:"WPI_MotorControlRefNum Registry Get.vi"("refnum name"="Feeder") -> ("error out"=w397:errorcluster, "MotorControlDevRef"=w398:T6)  [unwired: 9 in]
          n167 = call <vilib>:"WPI_MotorControlRefNum Registry Get.vi"("refnum name"="Shuriken") -> ("error out"=w399:errorcluster, "MotorControlDevRef"=w400:T6)  [unwired: 9 in]
          n168 = call <vilib>:"WPI_MotorControlSetOutput.vi"("error in (no error)"=w397, "Output"=w395, "MotorControlDevRef"=w398) -> ()  [unwired: 6 in, 3 out]
          n169 = call <vilib>:"WPI_MotorControlSetOutput.vi"("error in (no error)"=w399, "Output"=0.0, "MotorControlDevRef"=w400) -> ()  [unwired: 6 in, 3 out]
        }
      }
    }
    frame "HopperRight" {
      n170 = flat-sequence {
        tunnel: w419 -> [w441]
        tunnel: w418 -> [w440]
        tunnel: w417 -> [w439]
        tunnel: w412 -> [w438]
        tunnel: w433 -> [_]
        tunnel: w432 -> [_]
        tunnel: w428 -> [_]
        tunnel: w427 -> [_]
        tunnel: [w463] -> w423
        tunnel: w422 -> [w462]
        tunnel: w421 -> [w461]
        tunnel: w420 -> [w460]
        tunnel: w413 -> [w459]
        tunnel: [w541] -> w424
        tunnel: w423 -> [w541]
        tunnel: w431 -> [_]
        tunnel: w430 -> [_]
        tunnel: w429 -> [_]
        tunnel: [w560] -> w425
        tunnel: w424 -> [w560]
        tunnel: w411 -> [w557]
        tunnel: w410 -> [w556]
        tunnel: w409 -> [w555]
        tunnel: w408 -> [w554]
        tunnel: [w586] -> w426
        tunnel: w425 -> [w586]
        tunnel: w426 -> [w606]
        tunnel: w416 -> [w602]
        tunnel: w415 -> [w601]
        tunnel: w414 -> [w600]
        tunnel: w406 -> [w599]
        tunnel: w416 -> [w668]
        tunnel: w415 -> [w667]
        tunnel: w414 -> [w666]
        tunnel: [w665] -> _
        tunnel: w407 -> [w665]
        frame #0 {
          n171 = call <vilib>:"WPI_MotorControlRefNum Registry Get.vi"("refnum name"="Shooter" ("Name")) -> ("error out"=w445:errorcluster, "MotorControlDevRef"=w446:T6)  [unwired: 9 in]
          n172 = call <vilib>:"WPI_SolenoidRefNum Registry Get.vi"("refnum name"="Banana") -> ("SolenoidDevRef"=w450:T10)  [unwired: 9 in, 1 out]
          n173 = call-poly <vilib>:"WPI_SolenoidSet.vi"("Value"=WPI_SolenoidValue."On", "SolenoidDevRef"=w450) -> ()  [unwired: 8 in, 2 out]
          n174 = call "TalonPID.vi"("P"=w440, "Ref In"=w446, "Error in"=w445, "I"=w441, "I Zone"=w438, "Output"=w439) -> ()  [unwired: 8 in, 2 out]
          n175 = call <vilib>:"WPI_SolenoidRefNum Registry Get.vi"("refnum name"="GearGate") -> ("error out"=w454:errorcluster, "SolenoidDevRef"=w453:T10)  [unwired: 9 in]
          n176 = call-poly <vilib>:"WPI_SolenoidSet.vi"("error in (no error)"=w454, "Value"=WPI_SolenoidValue."On", "SolenoidDevRef"=w453) -> ()  [unwired: 7 in, 2 out]
          n177 = call "Z900_navX_RefNum_Get.vi"("refnum name"="navX") -> ("error out"=w443:errorcluster, "navX Device"=w444:T12)  [unwired: 9 in]
          n178 = call <vilib>:"WPI_SolenoidRefNum Registry Get.vi"("refnum name"="HopperHitter") -> ("error out"=w435:errorcluster, "SolenoidDevRef"=w436:T10)  [unwired: 9 in]
          n179 = call "Z900_navX_Set_ZeroYaw.vi"("error in (no error)"=w443, "navX Device"=w444) -> ()  [unwired: 8 in, 2 out]
          n180 = call-poly <vilib>:"WPI_SolenoidSet.vi"("error in (no error)"=w435, "Value"=WPI_SolenoidValue."On", "SolenoidDevRef"=w436) -> ()  [unwired: 7 in, 2 out]
        }
        frame #1 {
          n181 = call <vilib>:"WPI_SolenoidRefNum Registry Get.vi"("refnum name"="HopperHitter") -> ("error out"=w456:errorcluster, "SolenoidDevRef"=w457:T10)  [unwired: 9 in]
          n182 = call <vilib>:"WPI_EncoderRefNum Registry Get.vi"("refnum name"="Encoder 1") -> ("error out"=w475:errorcluster, "EncoderDevRef"=w477:T14)  [unwired: 9 in]
          n183 = call <vilib>:"WPI_EncoderRefNum Registry Get.vi"("refnum name"="Encoder 0") -> ("error out"=w476:errorcluster, "EncoderDevRef"=w478:T14)  [unwired: 9 in]
          n184 = call <vilib>:"WPI_SolenoidRefNum Registry Get.vi"("refnum name"="GearGate") -> ("error out"=w474:errorcluster, "SolenoidDevRef"=w473:T10)  [unwired: 9 in]
          n185 = call-poly <vilib>:"NT Read Value.vi"("Default Value"=14.0, "Name"="Circumference") -> ("Numeric"=w464:dbl)  [unwired: 8 in, 1 out]
          n186 = call-poly <vilib>:"WPI_SolenoidSet.vi"("error in (no error)"=w474, "Value"=WPI_SolenoidValue."On", "SolenoidDevRef"=w473) -> ()  [unwired: 7 in, 2 out]
          n187 = call-poly <vilib>:"WPI_SolenoidSet.vi"("error in (no error)"=w456, "Value"=WPI_SolenoidValue."On", "SolenoidDevRef"=w457) -> ()  [unwired: 7 in, 2 out]
          n188 = call <vilib>:"WPI_EncoderReset.vi"("error in (no error)"=w476, "EncoderDevRef"=w478) -> ("error out"=w469:errorcluster, "EncoderDevRef"=w470:T14)  [unwired: 8 in]
          n189 = call <vilib>:"WPI_EncoderReset.vi"("error in (no error)"=w475, "EncoderDevRef"=w477) -> ("error out"=w467:errorcluster, "EncoderDevRef"=w468:T14)  [unwired: 8 in]
          n190 = while {
            tunnel: w470 -> [w515]
            tunnel: w469 -> [w514]
            tunnel: w468 -> [w513]
            tunnel: w467 -> [w512]
            tunnel: w464 -> [w497]
            tunnel: ["ForwardPID 3"] -> w463
            tunnel: w462 -> [w488]
            tunnel: w461 -> [w487]
            tunnel: w460 -> [w486]
            tunnel: w459 -> [w485]
            i -> [w502]
            stop <- w498 stop-if-true
            w496 = 0.65 ("x")
            n191 = call <vilib>:"WPI_EncoderGet.vi"("error in (no error)"=w514, "EncoderDevRef"=w515) -> ("Distance"=w511:dbl)  [unwired: 4 in, 5 out]
            n192 = call <vilib>:"WPI_EncoderGet.vi"("error in (no error)"=w512, "EncoderDevRef"=w513) -> ("Distance"=w510:dbl)  [unwired: 4 in, 5 out]
            n193 = Subtract(x=w511, y=w510) -> (x-y=w525:dbl)
            n194 = call "Z900_navX_RefNum_Get.vi"("refnum name"="navX") -> ("error out"=w490:errorcluster, "navX Device"=w491:T12)  [unwired: 9 in]
            n195 = call "Z900_navX_Set_ZeroYaw.vi"("error in (no error)"=w490, "navX Device"=w491) -> ()  [unwired: 8 in, 2 out]
            n196 = Add(x=w511, y=w510) -> (x+y=w509:dbl)
            n197 = call-poly <vilib>:"PID.vi"("output range"=cluster{"output high":dbl, "output low":dbl} {"output high"=0.5, "output low"=-0.5}, "PID gains"="ForwardPID 3", "process variable"=w525, "setpoint"=0.0) -> ("output"=w531:dbl)  [unwired: 6 in, 1 out]
            n198 = Divide(x=w509, y=2.0) -> (x/y=w504:dbl)
            n199 = Subtract(x=w496, y=w531) -> (x-y=w527:dbl)
            n200 = Add(x=w496, y=w531) -> (x+y=w526:dbl)
            n201 = call <vilib>:"WPI_RobotDriveRefNum Registry Get.vi"("refnum name"="RobotDrive") -> ("RobotDriveDevRef"=w533:T5)  [unwired: 9 in, 1 out]
            n202 = Greater?(x=w502, y=600) -> (0:w499:bool)
            n203 = Divide(x=72.0, y=w497) -> (x/y=w506:dbl)
            n204 = call <vilib>:"WPI_SolenoidRefNum Registry Get.vi"("refnum name"="GearGate") -> ("error out"=w522:errorcluster, "SolenoidDevRef"=w521:T10)  [unwired: 9 in]
            n205 = call <vilib>:"WPI_RobotDriveTankDrive.vi"("Right axis value"=w526, "Left axis value"=w527, "RobotDriveDevRef"=w533) -> ()  [unwired: 6 in, 3 out]
            n206 = Multiply(x=w506, y=1024.0) -> (x*y=w503:dbl)
            n207 = Greater Or Equal?(x=w504, y=w503) -> (x >= y?=w500:bool)
            n208 = call-poly <vilib>:"WPI_SolenoidSet.vi"("error in (no error)"=w522, "Value"=WPI_SolenoidValue."On", "SolenoidDevRef"=w521) -> ()  [unwired: 7 in, 2 out]
            n209 = Or(x=w500, y=w499) -> (x .or. y?=w498:bool)
            n210 = Build Array(w527, w526, w525) -> (w523:dbl[])
            n211 = Array To Cluster(array=w523) -> (cluster=→"DriveStraight 6":T1)
            n212 = call <vilib>:"WPI_MotorControlRefNum Registry Get.vi"("refnum name"="Shooter" ("Name")) -> ("error out"=w492:errorcluster, "MotorControlDevRef"=w493:T6)  [unwired: 9 in]
            n213 = call <vilib>:"WPI_SolenoidRefNum Registry Get.vi"("refnum name"="Banana") -> ("SolenoidDevRef"=w518:T10)  [unwired: 9 in, 1 out]
            n214 = call <vilib>:"WPI_SolenoidRefNum Registry Get.vi"("refnum name"="HopperHitter") -> ("error out"=w482:errorcluster, "SolenoidDevRef"=w483:T10)  [unwired: 9 in]
            n215 = call-poly <vilib>:"WPI_SolenoidSet.vi"("Value"=WPI_SolenoidValue."On", "SolenoidDevRef"=w518) -> ()  [unwired: 8 in, 2 out]
            n216 = call "TalonPID.vi"("P"=w486, "Ref In"=w493, "Error in"=w492, "I"=w487, "I Zone"=w485, "Output"=w488) -> ()  [unwired: 8 in, 2 out]
            n217 = call-poly <vilib>:"WPI_SolenoidSet.vi"("error in (no error)"=w482, "Value"=WPI_SolenoidValue."On", "SolenoidDevRef"=w483) -> ()  [unwired: 7 in, 2 out]
            n218 = Wait (ms)(milliseconds to wait=10) -> ()  [unwired: 1 out]
          }
        }
        frame #2 {
          w548 = 0.0 ("Right axis value")
          n219 = call <vilib>:"WPI_SolenoidRefNum Registry Get.vi"("refnum name"="HopperHitter") -> ("error out"=w535:errorcluster, "SolenoidDevRef"=w536:T10)  [unwired: 9 in]
          n220 = Wait (ms)(milliseconds to wait=500) -> ()  [unwired: 1 out]
          n221 = call <vilib>:"WPI_RobotDriveRefNum Registry Get.vi"("refnum name"="RobotDrive") -> ("RobotDriveDevRef"=w549:T5)  [unwired: 9 in, 1 out]
          n222 = call <vilib>:"WPI_SolenoidRefNum Registry Get.vi"("refnum name"="GearGate") -> ("error out"=w546:errorcluster, "SolenoidDevRef"=w545:T10)  [unwired: 9 in]
          n223 = call "Z900_navX_RefNum_Get.vi"("refnum name"="navX") -> ("error out"=w539:errorcluster, "navX Device"=w540:T12)  [unwired: 9 in]
          n224 = call-poly <vilib>:"WPI_SolenoidSet.vi"("error in (no error)"=w535, "Value"=WPI_SolenoidValue."On", "SolenoidDevRef"=w536) -> ()  [unwired: 7 in, 2 out]
          n225 = call <vilib>:"WPI_RobotDriveTankDrive.vi"("Right axis value"=w548, "Left axis value"=w548, "RobotDriveDevRef"=w549) -> ()  [unwired: 6 in, 3 out]
          n226 = call "Z900_navX_Set_ZeroYaw.vi"("error in (no error)"=w539, "navX Device"=w540) -> ()  [unwired: 8 in, 2 out]
          n227 = call-poly <vilib>:"WPI_SolenoidSet.vi"("error in (no error)"=w546, "Value"=WPI_SolenoidValue."On", "SolenoidDevRef"=w545) -> ()  [unwired: 7 in, 2 out]
        }
        frame #3 {
          n228 = call <vilib>:"WPI_SolenoidRefNum Registry Get.vi"("refnum name"="HopperHitter") -> ("error out"=w551:errorcluster, "SolenoidDevRef"=w552:T10)  [unwired: 9 in]
          n229 = call "Z900_navX_RefNum_Get.vi"("refnum name"="navX") -> ("error out"=w562:errorcluster, "navX Device"=w563:T12)  [unwired: 9 in]
          n230 = call "Z900_navX_Set_ZeroYaw.vi"("error in (no error)"=w562, "navX Device"=w563) -> ("error out"=w558:errorcluster, "navX Device"=w559:T12)  [unwired: 8 in]
          n231 = call-poly <vilib>:"WPI_SolenoidSet.vi"("error in (no error)"=w551, "Value"=WPI_SolenoidValue."On", "SolenoidDevRef"=w552) -> ()  [unwired: 7 in, 2 out]
          n232 = while {
            tunnel: w559 -> [w569]
            tunnel: w558 -> [w568]
            tunnel: w557 -> [w567]
            tunnel: w556 -> [w566]
            tunnel: w555 -> [w565]
            tunnel: w554 -> [w564]
            stop <- w570 stop-if-true
            w576 = 0.55 ("Right axis value")
            n233 = call "Z900_navX_Get_YPRHfH.vi"("error in (no error)"=w568, "navX Device"=w569) -> ("YRPHfH"=w572:T18)  [unwired: 6 in, 3 out]
            n234 = Unbundle By Name(w572) -> ("Yaw"=w571:dbl)
            n235 = call <vilib>:"WPI_MotorControlRefNum Registry Get.vi"("refnum name"="Shooter" ("Name")) -> ("error out"=w573:errorcluster, "MotorControlDevRef"=w574:T6)  [unwired: 9 in]
            n236 = call <vilib>:"WPI_RobotDriveRefNum Registry Get.vi"("refnum name"="RobotDrive") -> ("RobotDriveDevRef"=w580:T5)  [unwired: 9 in, 1 out]
            n237 = Multiply(x=-1.0, y=w576) -> (x*y=w577:dbl)
            n238 = call <vilib>:"WPI_RobotDriveTankDrive.vi"("Right axis value"=w577, "Left axis value"=w576, "RobotDriveDevRef"=w580) -> ()  [unwired: 6 in, 3 out]
            n239 = call "TalonPID.vi"("P"=w566, "Ref In"=w574, "Error in"=w573, "I"=w565, "I Zone"=w564, "Output"=w567) -> ()  [unwired: 8 in, 2 out]
            n240 = Less?(x=w571, y=-85.0) -> (x < y?=w570:bool)
          }
        }
        frame #4 {
          w592 = 0.0 ("Left axis value")
          n241 = call <vilib>:"WPI_SolenoidRefNum Registry Get.vi"("refnum name"="HopperHitter") -> ("error out"=w583:errorcluster, "SolenoidDevRef"=w584:T10)  [unwired: 9 in]
          n242 = call <vilib>:"WPI_RobotDriveRefNum Registry Get.vi"("refnum name"="RobotDrive") -> ("error out"=w593:errorcluster, "RobotDriveDevRef"=w594:T5)  [unwired: 9 in]
          n243 = call <vilib>:"WPI_SolenoidRefNum Registry Get.vi"("refnum name"="GearGate") -> ("error out"=w590:errorcluster, "SolenoidDevRef"=w589:T10)  [unwired: 9 in]
          n244 = call <vilib>:"WPI_RobotDriveTankDrive.vi"("error in (no error)"=w593, "Right axis value"=w592, "Left axis value"=w592, "RobotDriveDevRef"=w594) -> ()  [unwired: 5 in, 3 out]
          n245 = call-poly <vilib>:"WPI_SolenoidSet.vi"("error in (no error)"=w583, "Value"=WPI_SolenoidValue."On", "SolenoidDevRef"=w584) -> ()  [unwired: 7 in, 2 out]
          n246 = call-poly <vilib>:"WPI_SolenoidSet.vi"("error in (no error)"=w590, "Value"=WPI_SolenoidValue."On", "SolenoidDevRef"=w589) -> ()  [unwired: 7 in, 2 out]
        }
        frame #5 {
          n247 = call <vilib>:"WPI_SolenoidRefNum Registry Get.vi"("refnum name"="HopperHitter") -> ("error out"=w596:errorcluster, "SolenoidDevRef"=w597:T10)  [unwired: 9 in]
          n248 = call <vilib>:"WPI_EncoderRefNum Registry Get.vi"("refnum name"="Encoder 1") -> ("error out"=w615:errorcluster, "EncoderDevRef"=w617:T14)  [unwired: 9 in]
          n249 = call <vilib>:"WPI_EncoderRefNum Registry Get.vi"("refnum name"="Encoder 0") -> ("error out"=w616:errorcluster, "EncoderDevRef"=w618:T14)  [unwired: 9 in]
          n250 = call <vilib>:"WPI_SolenoidRefNum Registry Get.vi"("refnum name"="GearGate") -> ("error out"=w614:errorcluster, "SolenoidDevRef"=w613:T10)  [unwired: 9 in]
          n251 = call-poly <vilib>:"WPI_SolenoidSet.vi"("error in (no error)"=w596, "Value"=WPI_SolenoidValue."On", "SolenoidDevRef"=w597) -> ()  [unwired: 7 in, 2 out]
          n252 = call-poly <vilib>:"WPI_SolenoidSet.vi"("error in (no error)"=w614, "Value"=WPI_SolenoidValue."On", "SolenoidDevRef"=w613) -> ()  [unwired: 7 in, 2 out]
          n253 = call "Z900_navX_RefNum_Get.vi"("refnum name"="navX") -> ("error out"=w604:errorcluster, "navX Device"=w605:T12)  [unwired: 9 in]
          n254 = call <vilib>:"WPI_EncoderReset.vi"("error in (no error)"=w616, "EncoderDevRef"=w618) -> ("error out"=w609:errorcluster, "EncoderDevRef"=w610:T14)  [unwired: 8 in]
          n255 = call <vilib>:"WPI_EncoderReset.vi"("error in (no error)"=w615, "EncoderDevRef"=w617) -> ("error out"=w607:errorcluster, "EncoderDevRef"=w608:T14)  [unwired: 8 in]
          n256 = call "Z900_navX_Set_ZeroYaw.vi"("error in (no error)"=w604, "navX Device"=w605) -> ()  [unwired: 8 in, 2 out]
          n257 = while {
            tunnel: w610 -> [w642]
            tunnel: w609 -> [w641]
            tunnel: w608 -> [w640]
            tunnel: w607 -> [w639]
            tunnel: w606 -> [w633]
            tunnel: w602 -> [w628]
            tunnel: w601 -> [w627]
            tunnel: w600 -> [w626]
            tunnel: w599 -> [w625]
            i -> [w636]
            stop <- w629 stop-if-true
            w634 = -0.65 ("x")
            n258 = call <vilib>:"WPI_EncoderGet.vi"("error in (no error)"=w641, "EncoderDevRef"=w642) -> ("Distance"=w638:dbl)  [unwired: 4 in, 5 out]
            n259 = call <vilib>:"WPI_EncoderGet.vi"("error in (no error)"=w639, "EncoderDevRef"=w640) -> ("Distance"=w637:dbl)  [unwired: 4 in, 5 out]
            n260 = Subtract(x=w638, y=w637) -> (x-y=w652:dbl)
            n261 = call-poly <vilib>:"PID.vi"("output range"=cluster{"output high":dbl, "output low":dbl} {"output high"=0.5, "output low"=-0.5}, "PID gains"=w633, "process variable"=w652, "setpoint"=0.0) -> ("output"=w658:dbl)  [unwired: 6 in, 1 out]
            n262 = call <vilib>:"WPI_SolenoidRefNum Registry Get.vi"("refnum name"="HopperHitter") -> ("error out"=w622:errorcluster, "SolenoidDevRef"=w623:T10)  [unwired: 9 in]
            n263 = Subtract(x=w634, y=w658) -> (x-y=w654:dbl)
            n264 = Add(x=w634, y=w658) -> (x+y=w653:dbl)
            n265 = call <vilib>:"WPI_RobotDriveRefNum Registry Get.vi"("refnum name"="RobotDrive") -> ("RobotDriveDevRef"=w660:T5)  [unwired: 9 in, 1 out]
            n266 = call-poly <vilib>:"WPI_SolenoidSet.vi"("error in (no error)"=w622, "Value"=WPI_SolenoidValue."On", "SolenoidDevRef"=w623) -> ()  [unwired: 7 in, 2 out]
            n267 = Greater?(x=w636, y=75) -> (0:w629:bool)
            n268 = call <vilib>:"WPI_SolenoidRefNum Registry Get.vi"("refnum name"="GearGate") -> ("error out"=w649:errorcluster, "SolenoidDevRef"=w648:T10)  [unwired: 9 in]
            n269 = call <vilib>:"WPI_RobotDriveTankDrive.vi"("Right axis value"=w653, "Left axis value"=w654, "RobotDriveDevRef"=w660) -> ()  [unwired: 6 in, 3 out]
            n270 = call-poly <vilib>:"WPI_SolenoidSet.vi"("error in (no error)"=w649, "Value"=WPI_SolenoidValue."On", "SolenoidDevRef"=w648) -> ()  [unwired: 7 in, 2 out]
            n271 = Build Array(w654, w653, w652) -> (w650:dbl[])
            n272 = Array To Cluster(array=w650) -> (cluster=→"DriveStraight 7":T1)
            n273 = call <vilib>:"WPI_MotorControlRefNum Registry Get.vi"("refnum name"="Shooter" ("Name")) -> ("error out"=w630:errorcluster, "MotorControlDevRef"=w631:T6)  [unwired: 9 in]
            n274 = call <vilib>:"WPI_SolenoidRefNum Registry Get.vi"("refnum name"="Banana") -> ("SolenoidDevRef"=w645:T10)  [unwired: 9 in, 1 out]
            n275 = call-poly <vilib>:"WPI_SolenoidSet.vi"("Value"=WPI_SolenoidValue."On", "SolenoidDevRef"=w645) -> ()  [unwired: 8 in, 2 out]
            n276 = call "TalonPID.vi"("P"=w628, "Ref In"=w631, "Error in"=w630, "I"=w627, "I Zone"=w625, "Output"=w626) -> ()  [unwired: 8 in, 2 out]
            n277 = Wait (ms)(milliseconds to wait=10) -> ()  [unwired: 1 out]
          }
        }
        frame #6 {
          (unwired) 0.0 ("Right axis value")
          n278 = call <vilib>:"WPI_SolenoidRefNum Registry Get.vi"("refnum name"="HopperHitter") -> ("error out"=w662:errorcluster, "SolenoidDevRef"=w663:T10)  [unwired: 9 in]
          n279 = call <vilib>:"WPI_MotorControlRefNum Registry Get.vi"("refnum name"="Shooter" ("Name")) -> ("error out"=w669:errorcluster, "MotorControlDevRef"=w670:T6)  [unwired: 9 in]
          n280 = call-poly <vilib>:"WPI_SolenoidSet.vi"("error in (no error)"=w662, "Value"=WPI_SolenoidValue."On", "SolenoidDevRef"=w663) -> ()  [unwired: 7 in, 2 out]
          n281 = call "TalonPID.vi"("P"=w668, "Ref In"=w670, "Error in"=w669, "I"=w667, "I Zone"=w665, "Output"=w666) -> ()  [unwired: 8 in, 2 out]
          n282 = Multiply(x=0.9, y=-1.0) -> (x*y=w683:dbl)
          n283 = call <vilib>:"WPI_RobotDriveRefNum Registry Get.vi"("refnum name"="RobotDrive") -> ("error out"=w673:errorcluster, "RobotDriveDevRef"=w672:T5)  [unwired: 9 in]
          n284 = call <vilib>:"WPI_MotorControlRefNum Registry Get.vi"("refnum name"="Feeder") -> ("error out"=w681:errorcluster, "MotorControlDevRef"=w680:T6)  [unwired: 9 in]
          n285 = call <vilib>:"WPI_MotorControlRefNum Registry Get.vi"("refnum name"="Shuriken") -> ("error out"=w679:errorcluster, "MotorControlDevRef"=w678:T6)  [unwired: 9 in]
          n286 = call <vilib>:"WPI_RobotDriveTankDrive.vi"("error in (no error)"=w673, "Left axis value"=0.0, "RobotDriveDevRef"=w672) -> ()  [unwired: 6 in, 3 out]
          n287 = call <vilib>:"WPI_MotorControlSetOutput.vi"("error in (no error)"=w681, "Output"=w683, "MotorControlDevRef"=w680) -> ()  [unwired: 6 in, 3 out]
          n288 = call <vilib>:"WPI_MotorControlSetOutput.vi"("error in (no error)"=w679, "Output"=0.5, "MotorControlDevRef"=w678) -> ()  [unwired: 6 in, 3 out]
          n289 = Wait (ms)(milliseconds to wait=9000) -> ()  [unwired: 1 out]
        }
        frame #7 {
          n290 = call <vilib>:"WPI_MotorControlRefNum Registry Get.vi"("refnum name"="Shooter") -> ("MotorControlDevRef"=w708:T6)  [unwired: 9 in, 1 out]
          n291 = call <vilib>:"WPI_RobotDriveRefNum Registry Get.vi"("refnum name"="RobotDrive") -> ("error out"=w693:errorcluster, "RobotDriveDevRef"=w692:T5)  [unwired: 9 in]
          n292 = call <vilib>:"WPI_SolenoidRefNum Registry Get.vi"("refnum name"="HopperHitter") -> ("error out"=w689:errorcluster, "SolenoidDevRef"=w690:T10)  [unwired: 9 in]
          n293 = Multiply(x=0.0, y=-1.0) -> (x*y=w699:dbl)
          n294 = call <vilib>:"WPI_RobotDriveTankDrive.vi"("error in (no error)"=w693, "Right axis value"=0.0, "Left axis value"=0.0, "RobotDriveDevRef"=w692) -> ()  [unwired: 5 in, 3 out]
          n295 = call <vilib>:"WPI_CANTalonSRX_ChangeMode.vi"("Output"=0.0, "Control Mode"=WPI_CANTalonSRX_APIControlMode."Percent VBus", "CAN Talon SRX Ref"=w708) -> ()  [unwired: 7 in, 2 out]
          n296 = call-poly <vilib>:"WPI_SolenoidSet.vi"("error in (no error)"=w689, "Value"=WPI_SolenoidValue."On", "SolenoidDevRef"=w690) -> ()  [unwired: 7 in, 2 out]
          n297 = call <vilib>:"WPI_MotorControlRefNum Registry Get.vi"("refnum name"="Feeder") -> ("error out"=w701:errorcluster, "MotorControlDevRef"=w702:T6)  [unwired: 9 in]
          n298 = call <vilib>:"WPI_MotorControlRefNum Registry Get.vi"("refnum name"="Shuriken") -> ("error out"=w703:errorcluster, "MotorControlDevRef"=w704:T6)  [unwired: 9 in]
          n299 = call <vilib>:"WPI_MotorControlSetOutput.vi"("error in (no error)"=w701, "Output"=w699, "MotorControlDevRef"=w702) -> ()  [unwired: 6 in, 3 out]
          n300 = call <vilib>:"WPI_MotorControlSetOutput.vi"("error in (no error)"=w703, "Output"=0.0, "MotorControlDevRef"=w704) -> ()  [unwired: 6 in, 3 out]
        }
      }
    }
    frame "LeftGear" {
      n301 = flat-sequence {
        frame #0 {
          n302 = call <vilib>:"WPI_SolenoidRefNum Registry Get.vi"("refnum name"="Banana") -> ("SolenoidDevRef"=w712:T10)  [unwired: 9 in, 1 out]
          n303 = call-poly <vilib>:"WPI_SolenoidSet.vi"("Value"=WPI_SolenoidValue."On", "SolenoidDevRef"=w712) -> ()  [unwired: 8 in, 2 out]
          n304 = call <vilib>:"WPI_SolenoidRefNum Registry Get.vi"("refnum name"="GearGate") -> ("error out"=w716:errorcluster, "SolenoidDevRef"=w715:T10)  [unwired: 9 in]
          n305 = call-poly <vilib>:"WPI_SolenoidSet.vi"("error in (no error)"=w716, "Value"=WPI_SolenoidValue."On", "SolenoidDevRef"=w715) -> ()  [unwired: 7 in, 2 out]
        }
        frame #1 {
          n306 = call <vilib>:"WPI_EncoderRefNum Registry Get.vi"("refnum name"="Encoder 1") -> ("error out"=w728:errorcluster, "EncoderDevRef"=w730:T14)  [unwired: 9 in]
          n307 = call <vilib>:"WPI_EncoderRefNum Registry Get.vi"("refnum name"="Encoder 0") -> ("error out"=w729:errorcluster, "EncoderDevRef"=w731:T14)  [unwired: 9 in]
          n308 = call <vilib>:"WPI_SolenoidRefNum Registry Get.vi"("refnum name"="GearGate") -> ("error out"=w727:errorcluster, "SolenoidDevRef"=w726:T10)  [unwired: 9 in]
          n309 = call-poly <vilib>:"NT Read Value.vi"("Default Value"=14.0, "Name"="Circumference") -> ("Numeric"=w717:dbl)  [unwired: 8 in, 1 out]
          n310 = call-poly <vilib>:"WPI_SolenoidSet.vi"("error in (no error)"=w727, "Value"=WPI_SolenoidValue."On", "SolenoidDevRef"=w726) -> ()  [unwired: 7 in, 2 out]
          n311 = call <vilib>:"WPI_EncoderReset.vi"("error in (no error)"=w729, "EncoderDevRef"=w731) -> ("error out"=w722:errorcluster, "EncoderDevRef"=w723:T14)  [unwired: 8 in]
          n312 = call <vilib>:"WPI_EncoderReset.vi"("error in (no error)"=w728, "EncoderDevRef"=w730) -> ("error out"=w720:errorcluster, "EncoderDevRef"=w721:T14)  [unwired: 8 in]
          n313 = while {
            tunnel: w723 -> [w756]
            tunnel: w722 -> [w755]
            tunnel: w721 -> [w754]
            tunnel: w720 -> [w753]
            tunnel: w717 -> [w738]
            i -> [w743]
            stop <- w739 stop-if-true
            w737 = -0.5 ("x")
            n314 = call <vilib>:"WPI_EncoderGet.vi"("error in (no error)"=w755, "EncoderDevRef"=w756) -> ("Distance"=w752:dbl)  [unwired: 4 in, 5 out]
            n315 = call <vilib>:"WPI_EncoderGet.vi"("error in (no error)"=w753, "EncoderDevRef"=w754) -> ("Distance"=w751:dbl)  [unwired: 4 in, 5 out]
            n316 = Subtract(x=w752, y=w751) -> (x-y=w766:dbl)
            n317 = Add(x=w752, y=w751) -> (x+y=w750:dbl)
            n318 = call-poly <vilib>:"PID.vi"("output range"=cluster{"output high":dbl, "output low":dbl} {"output high"=0.5, "output low"=-0.5}, "PID gains"="ForwardPID 4", "process variable"=w766, "setpoint"=0.0) -> ("output"=w773:dbl)  [unwired: 6 in, 1 out]
            n319 = Divide(x=w750, y=2.0) -> (x/y=w745:dbl)
            n320 = Subtract(x=w737, y=w773) -> (x-y=w768:dbl)
            n321 = Add(x=w737, y=w773) -> (x+y=w767:dbl)
            n322 = call <vilib>:"WPI_RobotDriveRefNum Registry Get.vi"("refnum name"="RobotDrive") -> ("RobotDriveDevRef"=w775:T5)  [unwired: 9 in, 1 out]
            n323 = Greater?(x=w743, y=600) -> (0:w740:bool)
            n324 = Divide(x=58.0, y=w738) -> (x/y=w747:dbl)
            n325 = call <vilib>:"WPI_SolenoidRefNum Registry Get.vi"("refnum name"="GearGate") -> ("error out"=w763:errorcluster, "SolenoidDevRef"=w762:T10)  [unwired: 9 in]
            n326 = call <vilib>:"WPI_RobotDriveTankDrive.vi"("Right axis value"=w767, "Left axis value"=w768, "RobotDriveDevRef"=w775) -> ()  [unwired: 6 in, 3 out]
            n327 = Multiply(x=w747, y=-1024.0) -> (x*y=w744:dbl)
            n328 = Less Or Equal?(x=w745, y=w744) -> (x <= y?=w741:bool)
            n329 = call-poly <vilib>:"WPI_SolenoidSet.vi"("error in (no error)"=w763, "Value"=WPI_SolenoidValue."On", "SolenoidDevRef"=w762) -> ()  [unwired: 7 in, 2 out]
            n330 = Or(x=w741, y=w740) -> (x .or. y?=w739:bool)
            n331 = Build Array(w768, w767, w766) -> (w764:dbl[])
            n332 = Array To Cluster(array=w764) -> (cluster=→"DriveStraight 4":T1)
            n333 = call "Z900_navX_RefNum_Get.vi"("refnum name"="navX") -> ("error out"=w735:errorcluster, "navX Device"=w736:T12)  [unwired: 9 in]
            n334 = call <vilib>:"WPI_SolenoidRefNum Registry Get.vi"("refnum name"="Banana") -> ("SolenoidDevRef"=w759:T10)  [unwired: 9 in, 1 out]
            n335 = call "Z900_navX_Set_ZeroYaw.vi"("error in (no error)"=w735, "navX Device"=w736) -> ()  [unwired: 8 in, 2 out]
            n336 = call-poly <vilib>:"WPI_SolenoidSet.vi"("Value"=WPI_SolenoidValue."On", "SolenoidDevRef"=w759) -> ()  [unwired: 8 in, 2 out]
            n337 = Wait (ms)(milliseconds to wait=10) -> ()  [unwired: 1 out]
          }
        }
        frame #2 {
          n338 = call "Z900_navX_RefNum_Get.vi"("refnum name"="navX") -> ("error out"=w779:errorcluster, "navX Device"=w780:T12)  [unwired: 9 in]
          n339 = call "Z900_navX_Set_ZeroYaw.vi"("error in (no error)"=w779, "navX Device"=w780) -> ("error out"=w776:errorcluster, "navX Device"=w777:T12)  [unwired: 8 in]
          n340 = while {
            tunnel: w777 -> [w782]
            tunnel: w776 -> [w781]
            stop <- w783 stop-if-true
            w786 = -0.5 ("Right axis value")
            n341 = call "Z900_navX_Get_YPRHfH.vi"("error in (no error)"=w781, "navX Device"=w782) -> ("YRPHfH"=w785:T18)  [unwired: 6 in, 3 out]
            n342 = Unbundle By Name(w785) -> ("Yaw"=w784:dbl)
            n343 = call <vilib>:"WPI_RobotDriveRefNum Registry Get.vi"("refnum name"="RobotDrive") -> ("RobotDriveDevRef"=w790:T5)  [unwired: 9 in, 1 out]
            n344 = Multiply(x=-1.0, y=w786) -> (x*y=w787:dbl)
            n345 = call <vilib>:"WPI_RobotDriveTankDrive.vi"("Right axis value"=w787, "Left axis value"=w786, "RobotDriveDevRef"=w790) -> ()  [unwired: 6 in, 3 out]
            n346 = Greater Or Equal?(x=w784, y=62.0) -> (x >= y?=w783:bool)
          }
        }
        frame #3 {
          n347 = call <vilib>:"WPI_EncoderRefNum Registry Get.vi"("refnum name"="Encoder 1") -> ("error out"=w803:errorcluster, "EncoderDevRef"=w805:T14)  [unwired: 9 in]
          n348 = call <vilib>:"WPI_EncoderRefNum Registry Get.vi"("refnum name"="Encoder 0") -> ("error out"=w804:errorcluster, "EncoderDevRef"=w806:T14)  [unwired: 9 in]
          n349 = call <vilib>:"WPI_SolenoidRefNum Registry Get.vi"("refnum name"="GearGate") -> ("error out"=w802:errorcluster, "SolenoidDevRef"=w801:T10)  [unwired: 9 in]
          n350 = call-poly <vilib>:"NT Read Value.vi"("Default Value"=14.0, "Name"="Circumference") -> ("Numeric"=w792:dbl)  [unwired: 8 in, 1 out]
          n351 = call-poly <vilib>:"WPI_SolenoidSet.vi"("error in (no error)"=w802, "Value"=WPI_SolenoidValue."On", "SolenoidDevRef"=w801) -> ()  [unwired: 7 in, 2 out]
          n352 = call <vilib>:"WPI_EncoderReset.vi"("error in (no error)"=w804, "EncoderDevRef"=w806) -> ("error out"=w797:errorcluster, "EncoderDevRef"=w798:T14)  [unwired: 8 in]
          n353 = call <vilib>:"WPI_EncoderReset.vi"("error in (no error)"=w803, "EncoderDevRef"=w805) -> ("error out"=w795:errorcluster, "EncoderDevRef"=w796:T14)  [unwired: 8 in]
          n354 = while {
            tunnel: w798 -> [w828]
            tunnel: w797 -> [w827]
            tunnel: w796 -> [w826]
            tunnel: w795 -> [w825]
            tunnel: w792 -> [w810]
            i -> [w815]
            stop <- w811 stop-if-true
            w809 = -0.5 ("x")
            n355 = call <vilib>:"WPI_EncoderGet.vi"("error in (no error)"=w827, "EncoderDevRef"=w828) -> ("Distance"=w824:dbl)  [unwired: 4 in, 5 out]
            n356 = call <vilib>:"WPI_EncoderGet.vi"("error in (no error)"=w825, "EncoderDevRef"=w826) -> ("Distance"=w823:dbl)  [unwired: 4 in, 5 out]
            n357 = Subtract(x=w824, y=w823) -> (x-y=w838:dbl)
            n358 = Add(x=w824, y=w823) -> (x+y=w822:dbl)
            n359 = call-poly <vilib>:"PID.vi"("output range"=cluster{"output high":dbl, "output low":dbl} {"output high"=0.5, "output low"=-0.5}, "PID gains"="ForwardPID 5", "process variable"=w838, "setpoint"=0.0) -> ("output"=w845:dbl)  [unwired: 6 in, 1 out]
            n360 = Divide(x=w822, y=2.0) -> (x/y=w817:dbl)
            n361 = Subtract(x=w809, y=w845) -> (x-y=w840:dbl)
            n362 = Add(x=w809, y=w845) -> (x+y=w839:dbl)
            n363 = call <vilib>:"WPI_RobotDriveRefNum Registry Get.vi"("refnum name"="RobotDrive") -> ("RobotDriveDevRef"=w847:T5)  [unwired: 9 in, 1 out]
            n364 = Greater?(x=w815, y=600) -> (0:w812:bool)
            n365 = Divide(x=62.0, y=w810) -> (x/y=w819:dbl)
            n366 = call <vilib>:"WPI_SolenoidRefNum Registry Get.vi"("refnum name"="GearGate") -> ("error out"=w835:errorcluster, "SolenoidDevRef"=w834:T10)  [unwired: 9 in]
            n367 = call <vilib>:"WPI_RobotDriveTankDrive.vi"("Right axis value"=w839, "Left axis value"=w840, "RobotDriveDevRef"=w847) -> ()  [unwired: 6 in, 3 out]
            n368 = Multiply(x=w819, y=-1024.0) -> (x*y=w816:dbl)
            n369 = Less Or Equal?(x=w817, y=w816) -> (x <= y?=w813:bool)
            n370 = call-poly <vilib>:"WPI_SolenoidSet.vi"("error in (no error)"=w835, "Value"=WPI_SolenoidValue."On", "SolenoidDevRef"=w834) -> ()  [unwired: 7 in, 2 out]
            n371 = Or(x=w813, y=w812) -> (x .or. y?=w811:bool)
            n372 = Build Array(w840, w839, w838) -> (w836:dbl[])
            n373 = Array To Cluster(array=w836) -> (cluster=→"DriveStraight 5":T1)
            n374 = call <vilib>:"WPI_SolenoidRefNum Registry Get.vi"("refnum name"="Banana") -> ("SolenoidDevRef"=w831:T10)  [unwired: 9 in, 1 out]
            n375 = call-poly <vilib>:"WPI_SolenoidSet.vi"("Value"=WPI_SolenoidValue."On", "SolenoidDevRef"=w831) -> ()  [unwired: 8 in, 2 out]
            n376 = Wait (ms)(milliseconds to wait=10) -> ()  [unwired: 1 out]
          }
        }
        frame #4 {
          n377 = call <vilib>:"WPI_MotorControlRefNum Registry Get.vi"("refnum name"="Shooter") -> ("MotorControlDevRef"=w869:T6)  [unwired: 9 in, 1 out]
          n378 = call <vilib>:"WPI_RobotDriveRefNum Registry Get.vi"("refnum name"="RobotDrive") -> ("error out"=w854:errorcluster, "RobotDriveDevRef"=w853:T5)  [unwired: 9 in]
          n379 = call <vilib>:"WPI_SolenoidRefNum Registry Get.vi"("refnum name"="HopperHitter") -> ("error out"=w850:errorcluster, "SolenoidDevRef"=w851:T10)  [unwired: 9 in]
          n380 = Multiply(x=0.0, y=-1.0) -> (x*y=w860:dbl)
          n381 = call <vilib>:"WPI_RobotDriveTankDrive.vi"("error in (no error)"=w854, "Right axis value"=0.0, "Left axis value"=0.0, "RobotDriveDevRef"=w853) -> ()  [unwired: 5 in, 3 out]
          n382 = call <vilib>:"WPI_CANTalonSRX_ChangeMode.vi"("Output"=0.0, "Control Mode"=WPI_CANTalonSRX_APIControlMode."Percent VBus", "CAN Talon SRX Ref"=w869) -> ()  [unwired: 7 in, 2 out]
          n383 = call-poly <vilib>:"WPI_SolenoidSet.vi"("error in (no error)"=w850, "Value"=WPI_SolenoidValue."On", "SolenoidDevRef"=w851) -> ()  [unwired: 7 in, 2 out]
          n384 = call <vilib>:"WPI_MotorControlRefNum Registry Get.vi"("refnum name"="Feeder") -> ("error out"=w862:errorcluster, "MotorControlDevRef"=w863:T6)  [unwired: 9 in]
          n385 = call <vilib>:"WPI_MotorControlRefNum Registry Get.vi"("refnum name"="Shuriken") -> ("error out"=w864:errorcluster, "MotorControlDevRef"=w865:T6)  [unwired: 9 in]
          n386 = call <vilib>:"WPI_MotorControlSetOutput.vi"("error in (no error)"=w862, "Output"=w860, "MotorControlDevRef"=w863) -> ()  [unwired: 6 in, 3 out]
          n387 = call <vilib>:"WPI_MotorControlSetOutput.vi"("error in (no error)"=w864, "Output"=0.0, "MotorControlDevRef"=w865) -> ()  [unwired: 6 in, 3 out]
        }
      }
    }
    frame "RightGear", Default {
      n388 = flat-sequence {
        frame #0 {
          n389 = call <vilib>:"WPI_SolenoidRefNum Registry Get.vi"("refnum name"="Banana") -> ("SolenoidDevRef"=w873:T10)  [unwired: 9 in, 1 out]
          n390 = call-poly <vilib>:"WPI_SolenoidSet.vi"("Value"=WPI_SolenoidValue."On", "SolenoidDevRef"=w873) -> ()  [unwired: 8 in, 2 out]
          n391 = call <vilib>:"WPI_SolenoidRefNum Registry Get.vi"("refnum name"="GearGate") -> ("error out"=w877:errorcluster, "SolenoidDevRef"=w876:T10)  [unwired: 9 in]
          n392 = call-poly <vilib>:"WPI_SolenoidSet.vi"("error in (no error)"=w877, "Value"=WPI_SolenoidValue."On", "SolenoidDevRef"=w876) -> ()  [unwired: 7 in, 2 out]
        }
        frame #1 {
          n393 = call <vilib>:"WPI_EncoderRefNum Registry Get.vi"("refnum name"="Encoder 1") -> ("error out"=w889:errorcluster, "EncoderDevRef"=w891:T14)  [unwired: 9 in]
          n394 = call <vilib>:"WPI_EncoderRefNum Registry Get.vi"("refnum name"="Encoder 0") -> ("error out"=w890:errorcluster, "EncoderDevRef"=w892:T14)  [unwired: 9 in]
          n395 = call <vilib>:"WPI_SolenoidRefNum Registry Get.vi"("refnum name"="GearGate") -> ("error out"=w888:errorcluster, "SolenoidDevRef"=w887:T10)  [unwired: 9 in]
          n396 = call-poly <vilib>:"NT Read Value.vi"("Default Value"=14.0, "Name"="Circumference") -> ("Numeric"=w878:dbl)  [unwired: 8 in, 1 out]
          n397 = call-poly <vilib>:"WPI_SolenoidSet.vi"("error in (no error)"=w888, "Value"=WPI_SolenoidValue."On", "SolenoidDevRef"=w887) -> ()  [unwired: 7 in, 2 out]
          n398 = call <vilib>:"WPI_EncoderReset.vi"("error in (no error)"=w890, "EncoderDevRef"=w892) -> ("error out"=w883:errorcluster, "EncoderDevRef"=w884:T14)  [unwired: 8 in]
          n399 = call <vilib>:"WPI_EncoderReset.vi"("error in (no error)"=w889, "EncoderDevRef"=w891) -> ("error out"=w881:errorcluster, "EncoderDevRef"=w882:T14)  [unwired: 8 in]
          n400 = while {
            tunnel: w884 -> [w917]
            tunnel: w883 -> [w916]
            tunnel: w882 -> [w915]
            tunnel: w881 -> [w914]
            tunnel: w878 -> [w899]
            i -> [w904]
            stop <- w900 stop-if-true
            w898 = -0.5 ("x")
            n401 = call <vilib>:"WPI_EncoderGet.vi"("error in (no error)"=w916, "EncoderDevRef"=w917) -> ("Distance"=w913:dbl)  [unwired: 4 in, 5 out]
            n402 = call <vilib>:"WPI_EncoderGet.vi"("error in (no error)"=w914, "EncoderDevRef"=w915) -> ("Distance"=w912:dbl)  [unwired: 4 in, 5 out]
            n403 = Subtract(x=w913, y=w912) -> (x-y=w927:dbl)
            n404 = Add(x=w913, y=w912) -> (x+y=w911:dbl)
            n405 = call-poly <vilib>:"PID.vi"("output range"=cluster{"output high":dbl, "output low":dbl} {"output high"=0.5, "output low"=-0.5}, "PID gains"="ForwardPID 8", "process variable"=w927, "setpoint"=0.0) -> ("output"=w934:dbl)  [unwired: 6 in, 1 out]
            n406 = Divide(x=w911, y=2.0) -> (x/y=w906:dbl)
            n407 = Subtract(x=w898, y=w934) -> (x-y=w929:dbl)
            n408 = Add(x=w898, y=w934) -> (x+y=w928:dbl)
            n409 = call <vilib>:"WPI_RobotDriveRefNum Registry Get.vi"("refnum name"="RobotDrive") -> ("RobotDriveDevRef"=w936:T5)  [unwired: 9 in, 1 out]
            n410 = Greater?(x=w904, y=600) -> (0:w901:bool)
            n411 = Divide(x=58.0, y=w899) -> (x/y=w908:dbl)
            n412 = call <vilib>:"WPI_SolenoidRefNum Registry Get.vi"("refnum name"="GearGate") -> ("error out"=w924:errorcluster, "SolenoidDevRef"=w923:T10)  [unwired: 9 in]
            n413 = call <vilib>:"WPI_RobotDriveTankDrive.vi"("Right axis value"=w928, "Left axis value"=w929, "RobotDriveDevRef"=w936) -> ()  [unwired: 6 in, 3 out]
            n414 = Multiply(x=w908, y=-1024.0) -> (x*y=w905:dbl)
            n415 = Less Or Equal?(x=w906, y=w905) -> (x <= y?=w902:bool)
            n416 = call-poly <vilib>:"WPI_SolenoidSet.vi"("error in (no error)"=w924, "Value"=WPI_SolenoidValue."On", "SolenoidDevRef"=w923) -> ()  [unwired: 7 in, 2 out]
            n417 = Or(x=w902, y=w901) -> (x .or. y?=w900:bool)
            n418 = Build Array(w929, w928, w927) -> (w925:dbl[])
            n419 = Array To Cluster(array=w925) -> (cluster=→"DriveStraight 10":T1)
            n420 = call "Z900_navX_RefNum_Get.vi"("refnum name"="navX") -> ("error out"=w896:errorcluster, "navX Device"=w897:T12)  [unwired: 9 in]
            n421 = call <vilib>:"WPI_SolenoidRefNum Registry Get.vi"("refnum name"="Banana") -> ("SolenoidDevRef"=w920:T10)  [unwired: 9 in, 1 out]
            n422 = call "Z900_navX_Set_ZeroYaw.vi"("error in (no error)"=w896, "navX Device"=w897) -> ()  [unwired: 8 in, 2 out]
            n423 = call-poly <vilib>:"WPI_SolenoidSet.vi"("Value"=WPI_SolenoidValue."On", "SolenoidDevRef"=w920) -> ()  [unwired: 8 in, 2 out]
            n424 = Wait (ms)(milliseconds to wait=10) -> ()  [unwired: 1 out]
          }
        }
        frame #2 {
          n425 = call "Z900_navX_RefNum_Get.vi"("refnum name"="navX") -> ("error out"=w940:errorcluster, "navX Device"=w941:T12)  [unwired: 9 in]
          n426 = call "Z900_navX_Set_ZeroYaw.vi"("error in (no error)"=w940, "navX Device"=w941) -> ("error out"=w937:errorcluster, "navX Device"=w938:T12)  [unwired: 8 in]
          n427 = while {
            tunnel: w938 -> [w943]
            tunnel: w937 -> [w942]
            stop <- w944 stop-if-true
            w947 = 0.5 ("Right axis value")
            n428 = call "Z900_navX_Get_YPRHfH.vi"("error in (no error)"=w942, "navX Device"=w943) -> ("YRPHfH"=w946:T18)  [unwired: 6 in, 3 out]
            n429 = Unbundle By Name(w946) -> ("Yaw"=w945:dbl)
            n430 = call <vilib>:"WPI_RobotDriveRefNum Registry Get.vi"("refnum name"="RobotDrive") -> ("RobotDriveDevRef"=w951:T5)  [unwired: 9 in, 1 out]
            n431 = Multiply(x=-1.0, y=w947) -> (x*y=w948:dbl)
            n432 = call <vilib>:"WPI_RobotDriveTankDrive.vi"("Right axis value"=w948, "Left axis value"=w947, "RobotDriveDevRef"=w951) -> ()  [unwired: 6 in, 3 out]
            n433 = Less Or Equal?(x=w945, y=-62.0) -> (x <= y?=w944:bool)
          }
        }
        frame #3 {
          n434 = call <vilib>:"WPI_EncoderRefNum Registry Get.vi"("refnum name"="Encoder 1") -> ("error out"=w964:errorcluster, "EncoderDevRef"=w966:T14)  [unwired: 9 in]
          n435 = call <vilib>:"WPI_EncoderRefNum Registry Get.vi"("refnum name"="Encoder 0") -> ("error out"=w965:errorcluster, "EncoderDevRef"=w967:T14)  [unwired: 9 in]
          n436 = call <vilib>:"WPI_SolenoidRefNum Registry Get.vi"("refnum name"="GearGate") -> ("error out"=w963:errorcluster, "SolenoidDevRef"=w962:T10)  [unwired: 9 in]
          n437 = call-poly <vilib>:"NT Read Value.vi"("Default Value"=14.0, "Name"="Circumference") -> ("Numeric"=w953:dbl)  [unwired: 8 in, 1 out]
          n438 = call-poly <vilib>:"WPI_SolenoidSet.vi"("error in (no error)"=w963, "Value"=WPI_SolenoidValue."On", "SolenoidDevRef"=w962) -> ()  [unwired: 7 in, 2 out]
          n439 = call <vilib>:"WPI_EncoderReset.vi"("error in (no error)"=w965, "EncoderDevRef"=w967) -> ("error out"=w958:errorcluster, "EncoderDevRef"=w959:T14)  [unwired: 8 in]
          n440 = call <vilib>:"WPI_EncoderReset.vi"("error in (no error)"=w964, "EncoderDevRef"=w966) -> ("error out"=w956:errorcluster, "EncoderDevRef"=w957:T14)  [unwired: 8 in]
          n441 = while {
            tunnel: w959 -> [w989]
            tunnel: w958 -> [w988]
            tunnel: w957 -> [w987]
            tunnel: w956 -> [w986]
            tunnel: w953 -> [w971]
            i -> [w976]
            stop <- w972 stop-if-true
            w970 = -0.5 ("x")
            n442 = call <vilib>:"WPI_EncoderGet.vi"("error in (no error)"=w988, "EncoderDevRef"=w989) -> ("Distance"=w985:dbl)  [unwired: 4 in, 5 out]
            n443 = call <vilib>:"WPI_EncoderGet.vi"("error in (no error)"=w986, "EncoderDevRef"=w987) -> ("Distance"=w984:dbl)  [unwired: 4 in, 5 out]
            n444 = Subtract(x=w985, y=w984) -> (x-y=w999:dbl)
            n445 = Add(x=w985, y=w984) -> (x+y=w983:dbl)
            n446 = call-poly <vilib>:"PID.vi"("output range"=cluster{"output high":dbl, "output low":dbl} {"output high"=0.5, "output low"=-0.5}, "PID gains"="ForwardPID 9", "process variable"=w999, "setpoint"=0.0) -> ("output"=w1006:dbl)  [unwired: 6 in, 1 out]
            n447 = Divide(x=w983, y=2.0) -> (x/y=w978:dbl)
            n448 = Subtract(x=w970, y=w1006) -> (x-y=w1001:dbl)
            n449 = Add(x=w970, y=w1006) -> (x+y=w1000:dbl)
            n450 = call <vilib>:"WPI_RobotDriveRefNum Registry Get.vi"("refnum name"="RobotDrive") -> ("RobotDriveDevRef"=w1008:T5)  [unwired: 9 in, 1 out]
            n451 = Greater?(x=w976, y=600) -> (0:w973:bool)
            n452 = Divide(x=70.0, y=w971) -> (x/y=w980:dbl)
            n453 = call <vilib>:"WPI_SolenoidRefNum Registry Get.vi"("refnum name"="GearGate") -> ("error out"=w996:errorcluster, "SolenoidDevRef"=w995:T10)  [unwired: 9 in]
            n454 = call <vilib>:"WPI_RobotDriveTankDrive.vi"("Right axis value"=w1000, "Left axis value"=w1001, "RobotDriveDevRef"=w1008) -> ()  [unwired: 6 in, 3 out]
            n455 = Multiply(x=w980, y=-1024.0) -> (x*y=w977:dbl)
            n456 = Less Or Equal?(x=w978, y=w977) -> (x <= y?=w974:bool)
            n457 = call-poly <vilib>:"WPI_SolenoidSet.vi"("error in (no error)"=w996, "Value"=WPI_SolenoidValue."On", "SolenoidDevRef"=w995) -> ()  [unwired: 7 in, 2 out]
            n458 = Or(x=w974, y=w973) -> (x .or. y?=w972:bool)
            n459 = Build Array(w1001, w1000, w999) -> (w997:dbl[])
            n460 = Array To Cluster(array=w997) -> (cluster=→"DriveStraight 11":T1)
            n461 = call <vilib>:"WPI_SolenoidRefNum Registry Get.vi"("refnum name"="Banana") -> ("SolenoidDevRef"=w992:T10)  [unwired: 9 in, 1 out]
            n462 = call-poly <vilib>:"WPI_SolenoidSet.vi"("Value"=WPI_SolenoidValue."On", "SolenoidDevRef"=w992) -> ()  [unwired: 8 in, 2 out]
            n463 = Wait (ms)(milliseconds to wait=10) -> ()  [unwired: 1 out]
          }
        }
        frame #4 {
          n464 = call <vilib>:"WPI_MotorControlRefNum Registry Get.vi"("refnum name"="Shooter") -> ("MotorControlDevRef"=w1030:T6)  [unwired: 9 in, 1 out]
          n465 = call <vilib>:"WPI_RobotDriveRefNum Registry Get.vi"("refnum name"="RobotDrive") -> ("error out"=w1015:errorcluster, "RobotDriveDevRef"=w1014:T5)  [unwired: 9 in]
          n466 = call <vilib>:"WPI_SolenoidRefNum Registry Get.vi"("refnum name"="HopperHitter") -> ("error out"=w1011:errorcluster, "SolenoidDevRef"=w1012:T10)  [unwired: 9 in]
          n467 = Multiply(x=0.0, y=-1.0) -> (x*y=w1021:dbl)
          n468 = call <vilib>:"WPI_RobotDriveTankDrive.vi"("error in (no error)"=w1015, "Right axis value"=0.0, "Left axis value"=0.0, "RobotDriveDevRef"=w1014) -> ()  [unwired: 5 in, 3 out]
          n469 = call <vilib>:"WPI_CANTalonSRX_ChangeMode.vi"("Output"=0.0, "Control Mode"=WPI_CANTalonSRX_APIControlMode."Percent VBus", "CAN Talon SRX Ref"=w1030) -> ()  [unwired: 7 in, 2 out]
          n470 = call-poly <vilib>:"WPI_SolenoidSet.vi"("error in (no error)"=w1011, "Value"=WPI_SolenoidValue."On", "SolenoidDevRef"=w1012) -> ()  [unwired: 7 in, 2 out]
          n471 = call <vilib>:"WPI_MotorControlRefNum Registry Get.vi"("refnum name"="Feeder") -> ("error out"=w1023:errorcluster, "MotorControlDevRef"=w1024:T6)  [unwired: 9 in]
          n472 = call <vilib>:"WPI_MotorControlRefNum Registry Get.vi"("refnum name"="Shuriken") -> ("error out"=w1025:errorcluster, "MotorControlDevRef"=w1026:T6)  [unwired: 9 in]
          n473 = call <vilib>:"WPI_MotorControlSetOutput.vi"("error in (no error)"=w1023, "Output"=w1021, "MotorControlDevRef"=w1024) -> ()  [unwired: 6 in, 3 out]
          n474 = call <vilib>:"WPI_MotorControlSetOutput.vi"("error in (no error)"=w1025, "Output"=0.0, "MotorControlDevRef"=w1026) -> ()  [unwired: 6 in, 3 out]
        }
      }
    }
    frame "frontGear" {
      n475 = flat-sequence {
        tunnel: w1043 -> [w1052]
        tunnel: w1042 -> [w1051]
        tunnel: w1041 -> [w1054]
        tunnel: w1040 -> [w1053]
        tunnel: w1050 -> [_]
        tunnel: w1049 -> [_]
        tunnel: w1045 -> [_]
        tunnel: w1044 -> [_]
        tunnel: w1039 -> [w1068]
        tunnel: w1038 -> [w1067]
        tunnel: w1037 -> [w1066]
        tunnel: w1036 -> [w1065]
        tunnel: w1048 -> [w1143]
        tunnel: w1047 -> [w1142]
        tunnel: w1046 -> [w1141]
        tunnel: w1035 -> [w1213]
        tunnel: w1034 -> [w1212]
        tunnel: w1033 -> [w1211]
        tunnel: w1032 -> [w1210]
        tunnel: w1035 -> [w1242]
        tunnel: w1034 -> [w1241]
        tunnel: w1033 -> [w1240]
        tunnel: w1032 -> [w1239]
        tunnel: w1035 -> [w1254]
        tunnel: w1034 -> [w1253]
        tunnel: w1033 -> [w1252]
        tunnel: w1032 -> [w1251]
        frame #0 {
          n476 = call <vilib>:"WPI_SolenoidRefNum Registry Get.vi"("refnum name"="Banana") -> ("SolenoidDevRef"=w1060:T10)  [unwired: 9 in, 1 out]
          n477 = call <vilib>:"WPI_MotorControlRefNum Registry Get.vi"("refnum name"="Shooter" ("Name")) -> ("error out"=w1055:errorcluster, "MotorControlDevRef"=w1056:T6)  [unwired: 9 in]
          n478 = call-poly <vilib>:"WPI_SolenoidSet.vi"("Value"=WPI_SolenoidValue."On", "SolenoidDevRef"=w1060) -> ()  [unwired: 8 in, 2 out]
          n479 = call <vilib>:"WPI_SolenoidRefNum Registry Get.vi"("refnum name"="GearGate") -> ("error out"=w1064:errorcluster, "SolenoidDevRef"=w1063:T10)  [unwired: 9 in]
          n480 = call-poly <vilib>:"WPI_SolenoidSet.vi"("error in (no error)"=w1064, "Value"=WPI_SolenoidValue."On", "SolenoidDevRef"=w1063) -> ()  [unwired: 7 in, 2 out]
          n481 = call "TalonPID.vi"("P"=w1052, "Ref In"=w1056, "Error in"=w1055, "I"=w1054, "I Zone"=w1053, "Output"=w1051) -> ()  [unwired: 8 in, 2 out]
        }
        frame #1 {
          n482 = call <vilib>:"WPI_EncoderRefNum Registry Get.vi"("refnum name"="Encoder 1") -> ("error out"=w1080:errorcluster, "EncoderDevRef"=w1082:T14)  [unwired: 9 in]
          n483 = call <vilib>:"WPI_EncoderRefNum Registry Get.vi"("refnum name"="Encoder 0") -> ("error out"=w1081:errorcluster, "EncoderDevRef"=w1083:T14)  [unwired: 9 in]
          n484 = call <vilib>:"WPI_SolenoidRefNum Registry Get.vi"("refnum name"="GearGate") -> ("error out"=w1079:errorcluster, "SolenoidDevRef"=w1078:T10)  [unwired: 9 in]
          n485 = call-poly <vilib>:"NT Read Value.vi"("Default Value"=14.0, "Name"="Circumference") -> ("Numeric"=w1069:dbl)  [unwired: 8 in, 1 out]
          n486 = call-poly <vilib>:"WPI_SolenoidSet.vi"("error in (no error)"=w1079, "Value"=WPI_SolenoidValue."On", "SolenoidDevRef"=w1078) -> ()  [unwired: 7 in, 2 out]
          n487 = call <vilib>:"WPI_EncoderReset.vi"("error in (no error)"=w1081, "EncoderDevRef"=w1083) -> ("error out"=w1074:errorcluster, "EncoderDevRef"=w1075:T14)  [unwired: 8 in]
          n488 = call <vilib>:"WPI_EncoderReset.vi"("error in (no error)"=w1080, "EncoderDevRef"=w1082) -> ("error out"=w1072:errorcluster, "EncoderDevRef"=w1073:T14)  [unwired: 8 in]
          n489 = while {
            tunnel: w1075 -> [w1112]
            tunnel: w1074 -> [w1111]
            tunnel: w1073 -> [w1110]
            tunnel: w1072 -> [w1109]
            tunnel: w1069 -> [w1094]
            tunnel: w1068 -> [w1089]
            tunnel: w1067 -> [w1088]
            tunnel: w1066 -> [w1087]
            tunnel: w1065 -> [w1086]
            i -> [w1099]
            stop <- w1095 stop-if-true
            w1093 = 0.6 ("x")
            n490 = call <vilib>:"WPI_EncoderGet.vi"("error in (no error)"=w1111, "EncoderDevRef"=w1112) -> ("Distance"=w1108:dbl)  [unwired: 4 in, 5 out]
            n491 = call <vilib>:"WPI_EncoderGet.vi"("error in (no error)"=w1109, "EncoderDevRef"=w1110) -> ("Distance"=w1107:dbl)  [unwired: 4 in, 5 out]
            n492 = Subtract(x=w1108, y=w1107) -> (x-y=w1122:dbl)
            n493 = Add(x=w1108, y=w1107) -> (x+y=w1106:dbl)
            n494 = call-poly <vilib>:"PID.vi"("output range"=cluster{"output high":dbl, "output low":dbl} {"output high"=0.5, "output low"=-0.5}, "PID gains"="ForwardPID 2", "process variable"=w1122, "setpoint"=0.0) -> ("output"=w1129:dbl)  [unwired: 6 in, 1 out]
            n495 = Divide(x=w1106, y=2.0) -> (x/y=w1101:dbl)
            n496 = Subtract(x=w1093, y=w1129) -> (x-y=w1124:dbl)
            n497 = Add(x=w1093, y=w1129) -> (x+y=w1123:dbl)
            n498 = call <vilib>:"WPI_RobotDriveRefNum Registry Get.vi"("refnum name"="RobotDrive") -> ("RobotDriveDevRef"=w1131:T5)  [unwired: 9 in, 1 out]
            n499 = Greater?(x=w1099, y=600) -> (0:w1096:bool)
            n500 = Divide(x=78.297, y=w1094) -> (x/y=w1103:dbl)
            n501 = call <vilib>:"WPI_SolenoidRefNum Registry Get.vi"("refnum name"="GearGate") -> ("error out"=w1119:errorcluster, "SolenoidDevRef"=w1118:T10)  [unwired: 9 in]
            n502 = call <vilib>:"WPI_RobotDriveTankDrive.vi"("Right axis value"=w1123, "Left axis value"=w1124, "RobotDriveDevRef"=w1131) -> ()  [unwired: 6 in, 3 out]
            n503 = Multiply(x=w1103, y=1024.0) -> (x*y=w1100:dbl)
            n504 = Greater Or Equal?(x=w1101, y=w1100) -> (x >= y?=w1097:bool)
            n505 = call-poly <vilib>:"WPI_SolenoidSet.vi"("error in (no error)"=w1119, "Value"=WPI_SolenoidValue."On", "SolenoidDevRef"=w1118) -> ()  [unwired: 7 in, 2 out]
            n506 = Or(x=w1097, y=w1096) -> (x .or. y?=w1095:bool)
            n507 = Build Array(w1124, w1123, w1122) -> (w1120:dbl[])
            n508 = Array To Cluster(array=w1120) -> (cluster=→"DriveStraight 2":T1)
            n509 = call <vilib>:"WPI_SolenoidRefNum Registry Get.vi"("refnum name"="Banana") -> ("SolenoidDevRef"=w1115:T10)  [unwired: 9 in, 1 out]
            n510 = call <vilib>:"WPI_MotorControlRefNum Registry Get.vi"("refnum name"="Shooter" ("Name")) -> ("error out"=w1090:errorcluster, "MotorControlDevRef"=w1091:T6)  [unwired: 9 in]
            n511 = call-poly <vilib>:"WPI_SolenoidSet.vi"("Value"=WPI_SolenoidValue."On", "SolenoidDevRef"=w1115) -> ()  [unwired: 8 in, 2 out]
            n512 = call "TalonPID.vi"("P"=w1088, "Ref In"=w1091, "Error in"=w1090, "I"=w1087, "I Zone"=w1086, "Output"=w1089) -> ()  [unwired: 8 in, 2 out]
            n513 = Wait (ms)(milliseconds to wait=10) -> ()  [unwired: 1 out]
          }
        }
        frame #2 {
          w1138 = 0.0 ("Right axis value")
          n514 = call <vilib>:"WPI_RobotDriveRefNum Registry Get.vi"("refnum name"="RobotDrive") -> ("RobotDriveDevRef"=w1139:T5)  [unwired: 9 in, 1 out]
          n515 = call <vilib>:"WPI_SolenoidRefNum Registry Get.vi"("refnum name"="GearGate") -> ("error out"=w1136:errorcluster, "SolenoidDevRef"=w1135:T10)  [unwired: 9 in]
          n516 = call <vilib>:"WPI_RobotDriveTankDrive.vi"("Right axis value"=w1138, "Left axis value"=w1138, "RobotDriveDevRef"=w1139) -> ()  [unwired: 6 in, 3 out]
          n517 = call-poly <vilib>:"WPI_SolenoidSet.vi"("error in (no error)"=w1136, "Value"=WPI_SolenoidValue."On", "SolenoidDevRef"=w1135) -> ()  [unwired: 7 in, 2 out]
          n518 = Wait (ms)(milliseconds to wait=500) -> ()  [unwired: 1 out]
        }
        frame #3 {
          n519 = for {
            N: 0 -> [_]
            tunnel: w1143 -> [w1149]
            tunnel: w1142 -> [w1148]
            tunnel: w1141 -> [w1147]
            n520 = global read "Robot Global Data.vi" "TargetsFound"() -> (w1150:bool)
            n521 = case shown="True" w1150 {
              tunnel: [w1158 w1174] -> w1153
              tunnel: [w1158 w1173] -> w1154
              tunnel: TRUE -> [_ w1169]
              tunnel: w1149 -> [_ w1168]
              tunnel: w1148 -> [_ w1167]
              tunnel: w1147 -> [_ w1166]
              frame False {
                w1158 = 0.0
              }
              frame True {
                n522 = call <vilib>:"WPI_SolenoidRefNum Registry Get.vi"("refnum name"="Banana") -> ("SolenoidDevRef"=w1161:T10)  [unwired: 9 in, 1 out]
                n523 = global read "Robot Global Data.vi" "Mid"() -> (w1177:dbl)
                n524 = Subtract(x=w1177, y=w1167) -> (x-y=w1171:dbl)
                n525 = Absolute Value(x=w1171) -> (abs(x)=w1176:dbl)
                n526 = Less?(x=w1176, y=w1166) -> (x < y?=w1175:bool)
                n527 = Greater?(x=w1171, y=0.0) -> (0:w1172:bool)
                n528 = call-poly <vilib>:"WPI_SolenoidSet.vi"("Value"=WPI_SolenoidValue."On", "SolenoidDevRef"=w1161) -> ()  [unwired: 8 in, 2 out]
                n529 = case shown="False" w1172 {
                  tunnel: w1175 -> [w1178 w1193]
                  tunnel: [w1179 w1191] -> w1174
                  tunnel: [w1180 w1192] -> w1173
                  tunnel: w1169 -> [_ _]
                  tunnel: w1168 -> [w1181 w1190]
                  frame False {
                    n530 = case shown="True" w1178 {
                      tunnel: [w1186 w1189] -> w1180
                      tunnel: [w1184 w1189] -> w1179
                      tunnel: w1181 -> [w1182 w1187]
                      frame False {
                        n531 = Multiply(x=w1182, y=1.0) -> (x*y=w1186:dbl)
                        n532 = Multiply(x=w1182, y=-1.2) -> (x*y=w1184:dbl)
                      }
                      frame True {
                        n533 = Multiply(x=w1187, y=1.2) -> (x*y=w1189:dbl)
                      }
                    }
                  }
                  frame True {
                    n534 = case shown="True" w1193 {
                      tunnel: [w1198 w1201] -> w1192
                      tunnel: [w1196 w1201] -> w1191
                      tunnel: w1190 -> [w1194 w1199]
                      frame False {
                        n535 = Multiply(x=w1194, y=1.0) -> (x*y=w1196:dbl)
                        n536 = Multiply(x=w1194, y=-1.0) -> (x*y=w1198:dbl)
                      }
                      frame True {
                        n537 = Multiply(x=w1199, y=1.2) -> (x*y=w1201:dbl)
                      }
                    }
                  }
                }
                n538 = call <vilib>:"WPI_SolenoidRefNum Registry Get.vi"("refnum name"="GearGate") -> ("error out"=w1165:errorcluster, "SolenoidDevRef"=w1164:T10)  [unwired: 9 in]
                n539 = call-poly <vilib>:"WPI_SolenoidSet.vi"("error in (no error)"=w1165, "Value"=WPI_SolenoidValue."On", "SolenoidDevRef"=w1164) -> ()  [unwired: 7 in, 2 out]
              }
            }
            n540 = call <vilib>:"WPI_SolenoidRefNum Registry Get.vi"("refnum name"="Banana") -> ("SolenoidDevRef"=w1146:T10)  [unwired: 9 in, 1 out]
            n541 = call-poly <vilib>:"WPI_SolenoidSet.vi"("Value"=WPI_SolenoidValue."On", "SolenoidDevRef"=w1146) -> ()  [unwired: 8 in, 2 out]
            n542 = call <vilib>:"WPI_RobotDriveRefNum Registry Get.vi"("refnum name"="RobotDrive") -> ("error out"=w1155:errorcluster, "RobotDriveDevRef"=w1156:T5)  [unwired: 9 in]
            n543 = Wait (ms)(milliseconds to wait=10) -> ()  [unwired: 1 out]
            n544 = call <vilib>:"WPI_RobotDriveTankDrive.vi"("error in (no error)"=w1155, "Right axis value"=w1153, "Left axis value"=w1154, "RobotDriveDevRef"=w1156) -> ()  [unwired: 5 in, 3 out]
          }
        }
        frame #4 {
          w1207 = 0.0 ("Left axis value")
          n545 = call <vilib>:"WPI_RobotDriveRefNum Registry Get.vi"("refnum name"="RobotDrive") -> ("error out"=w1208:errorcluster, "RobotDriveDevRef"=w1209:T5)  [unwired: 9 in]
          n546 = call <vilib>:"WPI_SolenoidRefNum Registry Get.vi"("refnum name"="GearGate") -> ("error out"=w1205:errorcluster, "SolenoidDevRef"=w1204:T10)  [unwired: 9 in]
          n547 = call <vilib>:"WPI_RobotDriveTankDrive.vi"("error in (no error)"=w1208, "Right axis value"=w1207, "Left axis value"=w1207, "RobotDriveDevRef"=w1209) -> ()  [unwired: 5 in, 3 out]
          n548 = call-poly <vilib>:"WPI_SolenoidSet.vi"("error in (no error)"=w1205, "Value"=WPI_SolenoidValue."On", "SolenoidDevRef"=w1204) -> ()  [unwired: 7 in, 2 out]
        }
        frame #5 {
          n549 = for {
            N: 3 -> [_]
            n550 = flat-sequence {
              frame #0 {
                n551 = call <vilib>:"WPI_SolenoidRefNum Registry Get.vi"("refnum name"="Gears") -> ("error out"=w1229:errorcluster, "SolenoidDevRef"=w1228:T10)  [unwired: 9 in]
                n552 = call <vilib>:"WPI_SolenoidRefNum Registry Get.vi"("refnum name"="GearGate") -> ("error out"=w1224:errorcluster, "SolenoidDevRef"=w1223:T10)  [unwired: 9 in]
                n553 = call-poly <vilib>:"WPI_SolenoidSet.vi"("error in (no error)"=w1229, "Value"=WPI_SolenoidValue."On", "SolenoidDevRef"=w1228) -> ()  [unwired: 7 in, 2 out]
                n554 = Wait (ms)(milliseconds to wait=166) -> ()  [unwired: 1 out]
                n555 = call-poly <vilib>:"WPI_SolenoidSet.vi"("error in (no error)"=w1224, "Value"=WPI_SolenoidValue."On", "SolenoidDevRef"=w1223) -> ()  [unwired: 7 in, 2 out]
              }
              frame #1 {
                n556 = call <vilib>:"WPI_SolenoidRefNum Registry Get.vi"("refnum name"="Gears") -> ("error out"=w1238:errorcluster, "SolenoidDevRef"=w1237:T10)  [unwired: 9 in]
                n557 = call <vilib>:"WPI_SolenoidRefNum Registry Get.vi"("refnum name"="GearGate") -> ("error out"=w1233:errorcluster, "SolenoidDevRef"=w1232:T10)  [unwired: 9 in]
                n558 = Wait (ms)(milliseconds to wait=166) -> ()  [unwired: 1 out]
                n559 = call-poly <vilib>:"WPI_SolenoidSet.vi"("error in (no error)"=w1238, "Value"=WPI_SolenoidValue."Off", "SolenoidDevRef"=w1237) -> ()  [unwired: 7 in, 2 out]
                n560 = call-poly <vilib>:"WPI_SolenoidSet.vi"("error in (no error)"=w1233, "Value"=WPI_SolenoidValue."On", "SolenoidDevRef"=w1232) -> ()  [unwired: 7 in, 2 out]
              }
            }
          }
          n561 = call <vilib>:"WPI_SolenoidRefNum Registry Get.vi"("refnum name"="Banana") -> ("SolenoidDevRef"=w1219:T10)  [unwired: 9 in, 1 out]
          n562 = call <vilib>:"WPI_MotorControlRefNum Registry Get.vi"("refnum name"="Shooter" ("Name")) -> ("error out"=w1214:errorcluster, "MotorControlDevRef"=w1215:T6)  [unwired: 9 in]
          n563 = call-poly <vilib>:"WPI_SolenoidSet.vi"("Value"=WPI_SolenoidValue."On", "SolenoidDevRef"=w1219) -> ()  [unwired: 8 in, 2 out]
          n564 = call "TalonPID.vi"("P"=w1212, "Ref In"=w1215, "Error in"=w1214, "I"=w1211, "I Zone"=w1210, "Output"=w1213) -> ()  [unwired: 8 in, 2 out]
        }
        frame #6 {
          w1248 = -0.7 ("Left axis value")
          n565 = call <vilib>:"WPI_RobotDriveRefNum Registry Get.vi"("refnum name"="RobotDrive") -> ("error out"=w1249:errorcluster, "RobotDriveDevRef"=w1250:T5)  [unwired: 9 in]
          n566 = call <vilib>:"WPI_RobotDriveTankDrive.vi"("error in (no error)"=w1249, "Right axis value"=w1248, "Left axis value"=w1248, "RobotDriveDevRef"=w1250) -> ()  [unwired: 5 in, 3 out]
          n567 = call <vilib>:"WPI_MotorControlRefNum Registry Get.vi"("refnum name"="Shooter" ("Name")) -> ("error out"=w1243:errorcluster, "MotorControlDevRef"=w1244:T6)  [unwired: 9 in]
          n568 = call "TalonPID.vi"("P"=w1241, "Ref In"=w1244, "Error in"=w1243, "I"=w1240, "I Zone"=w1239, "Output"=w1242) -> ()  [unwired: 8 in, 2 out]
          n569 = Wait (ms)(milliseconds to wait=4000) -> ()  [unwired: 1 out]
        }
        frame #7 {
          n570 = Wait (ms)(milliseconds to wait=4000) -> ()  [unwired: 1 out]
          n571 = Multiply(x=0.9, y=-1.0) -> (x*y=w1261:dbl)
          n572 = call <vilib>:"WPI_MotorControlRefNum Registry Get.vi"("refnum name"="Shooter" ("Name")) -> ("error out"=w1255:errorcluster, "MotorControlDevRef"=w1256:T6)  [unwired: 9 in]
          n573 = call "TalonPID.vi"("P"=w1253, "Ref In"=w1256, "Error in"=w1255, "I"=w1252, "I Zone"=w1251, "Output"=w1254) -> ()  [unwired: 8 in, 2 out]
          n574 = call <vilib>:"WPI_MotorControlRefNum Registry Get.vi"("refnum name"="Feeder") -> ("error out"=w1263:errorcluster, "MotorControlDevRef"=w1264:T6)  [unwired: 9 in]
          n575 = call <vilib>:"WPI_MotorControlRefNum Registry Get.vi"("refnum name"="Shuriken") -> ("error out"=w1265:errorcluster, "MotorControlDevRef"=w1266:T6)  [unwired: 9 in]
          n576 = call <vilib>:"WPI_RobotDriveRefNum Registry Get.vi"("refnum name"="RobotDrive") -> ("error out"=w1272:errorcluster, "RobotDriveDevRef"=w1273:T5)  [unwired: 9 in]
          n577 = call <vilib>:"WPI_MotorControlSetOutput.vi"("error in (no error)"=w1263, "Output"=w1261, "MotorControlDevRef"=w1264) -> ()  [unwired: 6 in, 3 out]
          n578 = call <vilib>:"WPI_MotorControlSetOutput.vi"("error in (no error)"=w1265, "Output"=0.5, "MotorControlDevRef"=w1266) -> ()  [unwired: 6 in, 3 out]
          n579 = call <vilib>:"WPI_RobotDriveTankDrive.vi"("error in (no error)"=w1272, "Right axis value"=0.0, "Left axis value"=0.0, "RobotDriveDevRef"=w1273) -> ()  [unwired: 5 in, 3 out]
        }
        frame #8 {
          w1274 = 0.0
          n580 = call <vilib>:"WPI_RobotDriveRefNum Registry Get.vi"("refnum name"="RobotDrive") -> ("error out"=w1279:errorcluster, "RobotDriveDevRef"=w1278:T5)  [unwired: 9 in]
          n581 = call <vilib>:"WPI_MotorControlRefNum Registry Get.vi"("refnum name"="Shooter" ("Name")) -> ("error out"=w1275:errorcluster, "MotorControlDevRef"=w1276:T6)  [unwired: 9 in]
          n582 = Multiply(x=0.0, y=-1.0) -> (x*y=w1285:dbl)
          n583 = call <vilib>:"WPI_RobotDriveTankDrive.vi"("error in (no error)"=w1279, "Right axis value"=0.0, "Left axis value"=0.0, "RobotDriveDevRef"=w1278) -> ()  [unwired: 5 in, 3 out]
          n584 = call "TalonPID.vi"("P"=w1274, "Ref In"=w1276, "Error in"=w1275, "I"=w1274, "D"=w1274, "F"=w1274, "I Zone"=w1274, "Output"=w1274) -> ()  [unwired: 6 in, 2 out]
          n585 = call <vilib>:"WPI_MotorControlRefNum Registry Get.vi"("refnum name"="Feeder") -> ("error out"=w1287:errorcluster, "MotorControlDevRef"=w1288:T6)  [unwired: 9 in]
          n586 = call <vilib>:"WPI_MotorControlRefNum Registry Get.vi"("refnum name"="Shuriken") -> ("error out"=w1289:errorcluster, "MotorControlDevRef"=w1290:T6)  [unwired: 9 in]
          n587 = call <vilib>:"WPI_MotorControlSetOutput.vi"("error in (no error)"=w1287, "Output"=w1285, "MotorControlDevRef"=w1288) -> ()  [unwired: 6 in, 3 out]
          n588 = call <vilib>:"WPI_MotorControlSetOutput.vi"("error in (no error)"=w1289, "Output"=0.0, "MotorControlDevRef"=w1290) -> ()  [unwired: 6 in, 3 out]
        }
      }
    }
    frame "sideGearLeftBoiler" {
      n589 = flat-sequence {
        tunnel: [w1301] -> w1293
        tunnel: w1293 -> [w1325]
        frame #0 {
          n590 = call <vilib>:"WPI_SolenoidRefNum Registry Get.vi"("refnum name"="Banana") -> ("SolenoidDevRef"=w1296:T10)  [unwired: 9 in, 1 out]
          n591 = call-poly <vilib>:"WPI_SolenoidSet.vi"("Value"=WPI_SolenoidValue."On", "SolenoidDevRef"=w1296) -> ()  [unwired: 8 in, 2 out]
          n592 = call "ReadFile.vi"("Name"="/home/lvuser/LeftPegPathBoiler.txt") -> ("Array - Numeric"=w1301:dbl[][])
          n593 = call <vilib>:"WPI_SolenoidRefNum Registry Get.vi"("refnum name"="GearGate") -> ("error out"=w1300:errorcluster, "SolenoidDevRef"=w1299:T10)  [unwired: 9 in]
          n594 = call-poly <vilib>:"WPI_SolenoidSet.vi"("error in (no error)"=w1300, "Value"=WPI_SolenoidValue."On", "SolenoidDevRef"=w1299) -> ()  [unwired: 7 in, 2 out]
        }
        frame #1 {
          # "Position PID or Velocity PID"
          n595 = call <vilib>:"WPI_SolenoidRefNum Registry Get.vi"("refnum name"="Banana") -> ("SolenoidDevRef"=w1324:T10)  [unwired: 9 in, 1 out]
          n596 = call-poly <vilib>:"WPI_SolenoidSet.vi"("Value"=WPI_SolenoidValue."On", "SolenoidDevRef"=w1324) -> ()  [unwired: 8 in, 2 out]
          n597 = call <vilib>:"WPI_EncoderRefNum Registry Get.vi"("refnum name"="Encoder 0") -> ("error out"=w1318:errorcluster, "EncoderDevRef"=w1317:T14)  [unwired: 9 in]
          n598 = call <vilib>:"WPI_EncoderRefNum Registry Get.vi"("refnum name"="Encoder 1") -> ("error out"=w1320:errorcluster, "EncoderDevRef"=w1319:T14)  [unwired: 9 in]
          n599 = call "Z900_navX_RefNum_Get.vi"("refnum name"="navX") -> ("error out"=w1309:errorcluster, "navX Device"=w1310:T12)  [unwired: 9 in]
          n600 = call "Z900_navX_Set_ZeroYaw.vi"("error in (no error)"=w1309, "navX Device"=w1310) -> ("error out"=w1307:errorcluster, "navX Device"=w1308:T12)  [unwired: 8 in]
          n601 = call <vilib>:"WPI_EncoderReset.vi"("error in (no error)"=w1318, "EncoderDevRef"=w1317) -> ("error out"=w1314:errorcluster, "EncoderDevRef"=w1315:T14)  [unwired: 8 in]
          n602 = call <vilib>:"WPI_EncoderReset.vi"("error in (no error)"=w1320, "EncoderDevRef"=w1319) -> ("error out"=w1313:errorcluster, "EncoderDevRef"=w1316:T14)  [unwired: 8 in]
          n603 = Array Size(array=w1325) -> (size(s)=w1329:i32[])
          n604 = call <vilib>:"WPI_RobotDriveRefNum Registry Get.vi"("refnum name"="RobotDrive") -> ("RobotDriveDevRef"=w1326:T5)  [unwired: 9 in, 1 out]
          n605 = Index Array(array=w1329, index=0) -> (element=w1321:i32)
          n606 = for {
            N: w1321 -> [_]
            tunnel: w1325 -> [w1347]
            tunnel: "PID gains R 2" -> [w1344]
            tunnel: "PID gains L 2" -> [w1343]
            tunnel: "Range 2" -> [w1342]
            tunnel: w1326 -> [w1341]
            tunnel: w1316 -> [w1340]
            tunnel: w1315 -> [w1339]
            tunnel: w1314 -> [w1338]
            tunnel: w1313 -> [w1337]
            tunnel: w1308 -> [w1334]
            tunnel: w1307 -> [w1333]
            i -> [w1346]
            n607 = Index Array(array=w1347, index (row)=w1346) -> (element=w1332:dbl[])  [unwired: 1 in]
            n608 = Index Array(array=w1332, index=0) -> (element=w1335:dbl)
            n609 = Index Array(array=w1332, index=1) -> (element=w1336:dbl)
            n610 = Index Array(array=w1332, index=2) -> (element=w1330:dbl)
            n611 = for {
              N: 10 -> [_]
              tunnel: w1344 -> [w1379]
              tunnel: w1343 -> [w1388]
              tunnel: w1342 -> [w1368]
              tunnel: w1341 -> [w1389]
              tunnel: w1340 -> [w1376]
              tunnel: w1339 -> [w1375]
              tunnel: w1338 -> [w1372]
              tunnel: w1337 -> [w1371]
              tunnel: w1335 -> [w1352]
              tunnel: w1336 -> [w1355]
              tunnel: w1334 -> [w1367]
              tunnel: w1333 -> [w1366]
              tunnel: w1330 -> [w1363]
              w1357 = 0.01
              w1377 = 0.0011393 ("x")
              n612 = call <vilib>:"WPI_EncoderGet.vi"("error in (no error)"=w1371, "EncoderDevRef"=w1376) -> ("Distance"=w1373:dbl)  [unwired: 4 in, 5 out]
              n613 = call <vilib>:"WPI_EncoderGet.vi"("error in (no error)"=w1372, "EncoderDevRef"=w1375) -> ("Distance"=w1374:dbl)  [unwired: 4 in, 5 out]
              n614 = Multiply(x=w1377, y=w1374) -> (x*y=w1378:dbl)
              n615 = Multiply(x=w1377, y=w1373) -> (x*y=w1387:dbl)
              n616 = call "Z900_navX_Get_YPRHfH.vi"("error in (no error)"=w1366, "navX Device"=w1367) -> ("YRPHfH"=w1365:T18)  [unwired: 6 in, 3 out]
              n617 = Unbundle By Name(w1365) -> ("Yaw"=w1364:dbl)
              n618 = call <vilib>:"WPI_SolenoidRefNum Registry Get.vi"("refnum name"="GearGate") -> ("error out"=w1386:errorcluster, "SolenoidDevRef"=w1385:T10)  [unwired: 9 in]
              n619 = call-poly <vilib>:"WPI_SolenoidSet.vi"("error in (no error)"=w1386, "Value"=WPI_SolenoidValue."On", "SolenoidDevRef"=w1385) -> ()  [unwired: 7 in, 2 out]
              n620 = Subtract(x=w1364, y=w1363) -> (x-y=w1362:dbl)
              n621 = Multiply(x=-1.0 ("Speed"), y=w1357) -> (x*y=w1359:dbl)
              n622 = Multiply(x=1.0, y=w1362) -> (x*y=w1360:dbl)
              n623 = Multiply(x=w1359, y=w1360) -> (x*y=w1351:dbl)
              n624 = Add(x=w1352, y=w1351) -> (x+y=w1353:dbl)
              n625 = call-poly <vilib>:"PID.vi"("output range"=w1368, "PID gains"=w1388, "process variable"=w1387, "setpoint"=w1353) -> ("output"=w1369:dbl)  [unwired: 6 in, 1 out]
              n626 = Multiply(x=w1360, y=w1357) -> (x*y=w1354:dbl)
              n627 = Add(x=w1355, y=w1354) -> (x+y=w1356:dbl)
              n628 = call-poly <vilib>:"PID.vi"("output range"=w1368, "PID gains"=w1379, "process variable"=w1378, "setpoint"=w1356) -> ("output"=w1370:dbl)  [unwired: 6 in, 1 out]
              n629 = call <vilib>:"WPI_RobotDriveTankDrive.vi"("Right axis value"=w1370, "Left axis value"=w1369, "RobotDriveDevRef"=w1389) -> ()  [unwired: 6 in, 3 out]
              n630 = call <vilib>:"WPI_SolenoidRefNum Registry Get.vi"("refnum name"="Banana") -> ("SolenoidDevRef"=w1382:T10)  [unwired: 9 in, 1 out]
              n631 = Wait (ms)(milliseconds to wait=10) -> ()  [unwired: 1 out]
              n632 = call-poly <vilib>:"WPI_SolenoidSet.vi"("Value"=WPI_SolenoidValue."On", "SolenoidDevRef"=w1382) -> ()  [unwired: 8 in, 2 out]
            }
          }
        }
        frame #2 {
          w1398 = 0.0 ("Left axis value")
          n633 = call <vilib>:"WPI_SolenoidRefNum Registry Get.vi"("refnum name"="Banana") -> ("SolenoidDevRef"=w1392:T10)  [unwired: 9 in, 1 out]
          n634 = call <vilib>:"WPI_RobotDriveRefNum Registry Get.vi"("refnum name"="RobotDrive") -> ("error out"=w1399:errorcluster, "RobotDriveDevRef"=w1400:T5)  [unwired: 9 in]
          n635 = call <vilib>:"WPI_SolenoidRefNum Registry Get.vi"("refnum name"="GearGate") -> ("error out"=w1396:errorcluster, "SolenoidDevRef"=w1395:T10)  [unwired: 9 in]
          n636 = call-poly <vilib>:"WPI_SolenoidSet.vi"("Value"=WPI_SolenoidValue."On", "SolenoidDevRef"=w1392) -> ()  [unwired: 8 in, 2 out]
          n637 = call <vilib>:"WPI_RobotDriveTankDrive.vi"("error in (no error)"=w1399, "Right axis value"=w1398, "Left axis value"=w1398, "RobotDriveDevRef"=w1400) -> ()  [unwired: 5 in, 3 out]
          n638 = call-poly <vilib>:"WPI_SolenoidSet.vi"("error in (no error)"=w1396, "Value"=WPI_SolenoidValue."On", "SolenoidDevRef"=w1395) -> ()  [unwired: 7 in, 2 out]
        }
        frame #3 {
          n639 = call-poly <vilib>:"NT Read Value.vi"("Name"="Drop Gear?") -> ("Boolean"=w1401:bool)  [unwired: 9 in, 1 out]
          n640 = call <vilib>:"WPI_SolenoidRefNum Registry Get.vi"("refnum name"="Banana") -> ("SolenoidDevRef"=w1405:T10)  [unwired: 9 in, 1 out]
          n641 = case shown="True" w1401 {
            tunnel: w1405 -> [_ w1407]
            tunnel: WPI_SolenoidValue."On" ("Value") -> [_ w1406]
            frame False {
            }
            frame True {
              n642 = for {
                N: 3 -> [_]
                n643 = flat-sequence {
                  frame #0 {
                    n644 = call <vilib>:"WPI_SolenoidRefNum Registry Get.vi"("refnum name"="Gears") -> ("error out"=w1417:errorcluster, "SolenoidDevRef"=w1416:T10)  [unwired: 9 in]
                    n645 = call <vilib>:"WPI_SolenoidRefNum Registry Get.vi"("refnum name"="GearGate") -> ("error out"=w1412:errorcluster, "SolenoidDevRef"=w1411:T10)  [unwired: 9 in]
                    n646 = call-poly <vilib>:"WPI_SolenoidSet.vi"("error in (no error)"=w1417, "Value"=WPI_SolenoidValue."On", "SolenoidDevRef"=w1416) -> ()  [unwired: 7 in, 2 out]
                    n647 = Wait (ms)(milliseconds to wait=166) -> ()  [unwired: 1 out]
                    n648 = call-poly <vilib>:"WPI_SolenoidSet.vi"("error in (no error)"=w1412, "Value"=WPI_SolenoidValue."On", "SolenoidDevRef"=w1411) -> ()  [unwired: 7 in, 2 out]
                  }
                  frame #1 {
                    n649 = call <vilib>:"WPI_SolenoidRefNum Registry Get.vi"("refnum name"="Gears") -> ("error out"=w1426:errorcluster, "SolenoidDevRef"=w1425:T10)  [unwired: 9 in]
                    n650 = call <vilib>:"WPI_SolenoidRefNum Registry Get.vi"("refnum name"="GearGate") -> ("error out"=w1421:errorcluster, "SolenoidDevRef"=w1420:T10)  [unwired: 9 in]
                    n651 = Wait (ms)(milliseconds to wait=166) -> ()  [unwired: 1 out]
                    n652 = call-poly <vilib>:"WPI_SolenoidSet.vi"("error in (no error)"=w1426, "Value"=WPI_SolenoidValue."Off", "SolenoidDevRef"=w1425) -> ()  [unwired: 7 in, 2 out]
                    n653 = call-poly <vilib>:"WPI_SolenoidSet.vi"("error in (no error)"=w1421, "Value"=WPI_SolenoidValue."On", "SolenoidDevRef"=w1420) -> ()  [unwired: 7 in, 2 out]
                  }
                }
              }
              n654 = call-poly <vilib>:"WPI_SolenoidSet.vi"("Value"=w1406, "SolenoidDevRef"=w1407) -> ()  [unwired: 8 in, 2 out]
            }
          }
        }
        frame #4 {
          w1429 = -0.7 ("Left axis value")
          n655 = call <vilib>:"WPI_RobotDriveRefNum Registry Get.vi"("refnum name"="RobotDrive") -> ("error out"=w1430:errorcluster, "RobotDriveDevRef"=w1431:T5)  [unwired: 9 in]
          n656 = call <vilib>:"WPI_RobotDriveTankDrive.vi"("error in (no error)"=w1430, "Right axis value"=w1429, "Left axis value"=w1429, "RobotDriveDevRef"=w1431) -> ()  [unwired: 5 in, 3 out]
          n657 = Wait (ms)(milliseconds to wait=1000) -> ()  [unwired: 1 out]
        }
        frame #5 {
          w1437 = 0.0 ("Left axis value")
          n658 = call <vilib>:"WPI_RobotDriveRefNum Registry Get.vi"("refnum name"="RobotDrive") -> ("error out"=w1438:errorcluster, "RobotDriveDevRef"=w1439:T5)  [unwired: 9 in]
          n659 = call <vilib>:"WPI_SolenoidRefNum Registry Get.vi"("refnum name"="GearGate") -> ("error out"=w1435:errorcluster, "SolenoidDevRef"=w1434:T10)  [unwired: 9 in]
          n660 = call <vilib>:"WPI_RobotDriveTankDrive.vi"("error in (no error)"=w1438, "Right axis value"=w1437, "Left axis value"=w1437, "RobotDriveDevRef"=w1439) -> ()  [unwired: 5 in, 3 out]
          n661 = call-poly <vilib>:"WPI_SolenoidSet.vi"("error in (no error)"=w1435, "Value"=WPI_SolenoidValue."Off", "SolenoidDevRef"=w1434) -> ()  [unwired: 7 in, 2 out]
        }
      }
    }
    frame "sideGearRightBoiler" {
      n662 = flat-sequence {
        tunnel: [w1448] -> w1440
        tunnel: w1440 -> [w1472]
        frame #0 {
          n663 = call <vilib>:"WPI_SolenoidRefNum Registry Get.vi"("refnum name"="Banana") -> ("SolenoidDevRef"=w1443:T10)  [unwired: 9 in, 1 out]
          n664 = call-poly <vilib>:"WPI_SolenoidSet.vi"("Value"=WPI_SolenoidValue."On", "SolenoidDevRef"=w1443) -> ()  [unwired: 8 in, 2 out]
          n665 = call "ReadFile.vi"("Name"="/home/lvuser/RightPegPathBoiler.txt") -> ("Array - Numeric"=w1448:dbl[][])
          n666 = call <vilib>:"WPI_SolenoidRefNum Registry Get.vi"("refnum name"="GearGate") -> ("error out"=w1447:errorcluster, "SolenoidDevRef"=w1446:T10)  [unwired: 9 in]
          n667 = call-poly <vilib>:"WPI_SolenoidSet.vi"("error in (no error)"=w1447, "Value"=WPI_SolenoidValue."On", "SolenoidDevRef"=w1446) -> ()  [unwired: 7 in, 2 out]
        }
        frame #1 {
          # "Position PID or Velocity PID"
          n668 = call <vilib>:"WPI_SolenoidRefNum Registry Get.vi"("refnum name"="Banana") -> ("SolenoidDevRef"=w1471:T10)  [unwired: 9 in, 1 out]
          n669 = call-poly <vilib>:"WPI_SolenoidSet.vi"("Value"=WPI_SolenoidValue."On", "SolenoidDevRef"=w1471) -> ()  [unwired: 8 in, 2 out]
          n670 = call <vilib>:"WPI_EncoderRefNum Registry Get.vi"("refnum name"="Encoder 0") -> ("error out"=w1465:errorcluster, "EncoderDevRef"=w1464:T14)  [unwired: 9 in]
          n671 = call <vilib>:"WPI_EncoderRefNum Registry Get.vi"("refnum name"="Encoder 1") -> ("error out"=w1467:errorcluster, "EncoderDevRef"=w1466:T14)  [unwired: 9 in]
          n672 = call "Z900_navX_RefNum_Get.vi"("refnum name"="navX") -> ("error out"=w1456:errorcluster, "navX Device"=w1457:T12)  [unwired: 9 in]
          n673 = call "Z900_navX_Set_ZeroYaw.vi"("error in (no error)"=w1456, "navX Device"=w1457) -> ("error out"=w1454:errorcluster, "navX Device"=w1455:T12)  [unwired: 8 in]
          n674 = call <vilib>:"WPI_EncoderReset.vi"("error in (no error)"=w1465, "EncoderDevRef"=w1464) -> ("error out"=w1461:errorcluster, "EncoderDevRef"=w1462:T14)  [unwired: 8 in]
          n675 = call <vilib>:"WPI_EncoderReset.vi"("error in (no error)"=w1467, "EncoderDevRef"=w1466) -> ("error out"=w1460:errorcluster, "EncoderDevRef"=w1463:T14)  [unwired: 8 in]
          n676 = Array Size(array=w1472) -> (size(s)=w1476:i32[])
          n677 = call <vilib>:"WPI_RobotDriveRefNum Registry Get.vi"("refnum name"="RobotDrive") -> ("RobotDriveDevRef"=w1473:T5)  [unwired: 9 in, 1 out]
          n678 = Index Array(array=w1476, index=0) -> (element=w1468:i32)
          n679 = for {
            N: w1468 -> [_]
            tunnel: w1472 -> [w1494]
            tunnel: "PID gains R 3" -> [w1491]
            tunnel: "PID gains L 3" -> [w1490]
            tunnel: "Range 3" -> [w1489]
            tunnel: w1473 -> [w1488]
            tunnel: w1463 -> [w1487]
            tunnel: w1462 -> [w1486]
            tunnel: w1461 -> [w1485]
            tunnel: w1460 -> [w1484]
            tunnel: w1455 -> [w1481]
            tunnel: w1454 -> [w1480]
            i -> [w1493]
            n680 = Index Array(array=w1494, index (row)=w1493) -> (element=w1479:dbl[])  [unwired: 1 in]
            n681 = Index Array(array=w1479, index=0) -> (element=w1482:dbl)
            n682 = Index Array(array=w1479, index=1) -> (element=w1483:dbl)
            n683 = Index Array(array=w1479, index=2) -> (element=w1477:dbl)
            n684 = for {
              N: 10 -> [_]
              tunnel: w1491 -> [w1526]
              tunnel: w1490 -> [w1535]
              tunnel: w1489 -> [w1515]
              tunnel: w1488 -> [w1536]
              tunnel: w1487 -> [w1523]
              tunnel: w1486 -> [w1522]
              tunnel: w1485 -> [w1519]
              tunnel: w1484 -> [w1518]
              tunnel: w1482 -> [w1499]
              tunnel: w1483 -> [w1502]
              tunnel: w1481 -> [w1514]
              tunnel: w1480 -> [w1513]
              tunnel: w1477 -> [w1510]
              w1504 = 0.01
              w1524 = 0.0011393 ("x")
              n685 = call <vilib>:"WPI_EncoderGet.vi"("error in (no error)"=w1518, "EncoderDevRef"=w1523) -> ("Distance"=w1520:dbl)  [unwired: 4 in, 5 out]
              n686 = call <vilib>:"WPI_EncoderGet.vi"("error in (no error)"=w1519, "EncoderDevRef"=w1522) -> ("Distance"=w1521:dbl)  [unwired: 4 in, 5 out]
              n687 = Multiply(x=w1524, y=w1521) -> (x*y=w1525:dbl)
              n688 = Multiply(x=w1524, y=w1520) -> (x*y=w1534:dbl)
              n689 = call "Z900_navX_Get_YPRHfH.vi"("error in (no error)"=w1513, "navX Device"=w1514) -> ("YRPHfH"=w1512:T18)  [unwired: 6 in, 3 out]
              n690 = Unbundle By Name(w1512) -> ("Yaw"=w1511:dbl)
              n691 = call <vilib>:"WPI_SolenoidRefNum Registry Get.vi"("refnum name"="GearGate") -> ("error out"=w1533:errorcluster, "SolenoidDevRef"=w1532:T10)  [unwired: 9 in]
              n692 = call-poly <vilib>:"WPI_SolenoidSet.vi"("error in (no error)"=w1533, "Value"=WPI_SolenoidValue."On", "SolenoidDevRef"=w1532) -> ()  [unwired: 7 in, 2 out]
              n693 = Subtract(x=w1511, y=w1510) -> (x-y=w1509:dbl)
              n694 = Multiply(x=-1.0 ("Speed"), y=w1504) -> (x*y=w1506:dbl)
              n695 = Multiply(x=1.0, y=w1509) -> (x*y=w1507:dbl)
              n696 = Multiply(x=w1506, y=w1507) -> (x*y=w1498:dbl)
              n697 = Add(x=w1499, y=w1498) -> (x+y=w1500:dbl)
              n698 = call-poly <vilib>:"PID.vi"("output range"=w1515, "PID gains"=w1535, "process variable"=w1534, "setpoint"=w1500) -> ("output"=w1516:dbl)  [unwired: 6 in, 1 out]
              n699 = Multiply(x=w1507, y=w1504) -> (x*y=w1501:dbl)
              n700 = Add(x=w1502, y=w1501) -> (x+y=w1503:dbl)
              n701 = call-poly <vilib>:"PID.vi"("output range"=w1515, "PID gains"=w1526, "process variable"=w1525, "setpoint"=w1503) -> ("output"=w1517:dbl)  [unwired: 6 in, 1 out]
              n702 = call <vilib>:"WPI_RobotDriveTankDrive.vi"("Right axis value"=w1517, "Left axis value"=w1516, "RobotDriveDevRef"=w1536) -> ()  [unwired: 6 in, 3 out]
              n703 = call <vilib>:"WPI_SolenoidRefNum Registry Get.vi"("refnum name"="Banana") -> ("SolenoidDevRef"=w1529:T10)  [unwired: 9 in, 1 out]
              n704 = Wait (ms)(milliseconds to wait=10) -> ()  [unwired: 1 out]
              n705 = call-poly <vilib>:"WPI_SolenoidSet.vi"("Value"=WPI_SolenoidValue."On", "SolenoidDevRef"=w1529) -> ()  [unwired: 8 in, 2 out]
            }
          }
        }
        frame #2 {
          w1545 = 0.0 ("Left axis value")
          n706 = call <vilib>:"WPI_SolenoidRefNum Registry Get.vi"("refnum name"="Banana") -> ("SolenoidDevRef"=w1539:T10)  [unwired: 9 in, 1 out]
          n707 = call <vilib>:"WPI_RobotDriveRefNum Registry Get.vi"("refnum name"="RobotDrive") -> ("error out"=w1546:errorcluster, "RobotDriveDevRef"=w1547:T5)  [unwired: 9 in]
          n708 = call <vilib>:"WPI_SolenoidRefNum Registry Get.vi"("refnum name"="GearGate") -> ("error out"=w1543:errorcluster, "SolenoidDevRef"=w1542:T10)  [unwired: 9 in]
          n709 = call-poly <vilib>:"WPI_SolenoidSet.vi"("Value"=WPI_SolenoidValue."On", "SolenoidDevRef"=w1539) -> ()  [unwired: 8 in, 2 out]
          n710 = call <vilib>:"WPI_RobotDriveTankDrive.vi"("error in (no error)"=w1546, "Right axis value"=w1545, "Left axis value"=w1545, "RobotDriveDevRef"=w1547) -> ()  [unwired: 5 in, 3 out]
          n711 = call-poly <vilib>:"WPI_SolenoidSet.vi"("error in (no error)"=w1543, "Value"=WPI_SolenoidValue."On", "SolenoidDevRef"=w1542) -> ()  [unwired: 7 in, 2 out]
        }
        frame #3 {
          n712 = call-poly <vilib>:"NT Read Value.vi"("Name"="Drop Gear?") -> ("Boolean"=w1548:bool)  [unwired: 9 in, 1 out]
          n713 = call <vilib>:"WPI_SolenoidRefNum Registry Get.vi"("refnum name"="Banana") -> ("SolenoidDevRef"=w1552:T10)  [unwired: 9 in, 1 out]
          n714 = case shown="True" w1548 {
            tunnel: w1552 -> [_ w1554]
            tunnel: WPI_SolenoidValue."On" ("Value") -> [_ w1553]
            frame False {
            }
            frame True {
              n715 = for {
                N: 3 -> [_]
                n716 = flat-sequence {
                  frame #0 {
                    n717 = call <vilib>:"WPI_SolenoidRefNum Registry Get.vi"("refnum name"="Gears") -> ("error out"=w1564:errorcluster, "SolenoidDevRef"=w1563:T10)  [unwired: 9 in]
                    n718 = call <vilib>:"WPI_SolenoidRefNum Registry Get.vi"("refnum name"="GearGate") -> ("error out"=w1559:errorcluster, "SolenoidDevRef"=w1558:T10)  [unwired: 9 in]
                    n719 = call-poly <vilib>:"WPI_SolenoidSet.vi"("error in (no error)"=w1564, "Value"=WPI_SolenoidValue."On", "SolenoidDevRef"=w1563) -> ()  [unwired: 7 in, 2 out]
                    n720 = Wait (ms)(milliseconds to wait=166) -> ()  [unwired: 1 out]
                    n721 = call-poly <vilib>:"WPI_SolenoidSet.vi"("error in (no error)"=w1559, "Value"=WPI_SolenoidValue."On", "SolenoidDevRef"=w1558) -> ()  [unwired: 7 in, 2 out]
                  }
                  frame #1 {
                    n722 = call <vilib>:"WPI_SolenoidRefNum Registry Get.vi"("refnum name"="Gears") -> ("error out"=w1573:errorcluster, "SolenoidDevRef"=w1572:T10)  [unwired: 9 in]
                    n723 = call <vilib>:"WPI_SolenoidRefNum Registry Get.vi"("refnum name"="GearGate") -> ("error out"=w1568:errorcluster, "SolenoidDevRef"=w1567:T10)  [unwired: 9 in]
                    n724 = Wait (ms)(milliseconds to wait=166) -> ()  [unwired: 1 out]
                    n725 = call-poly <vilib>:"WPI_SolenoidSet.vi"("error in (no error)"=w1573, "Value"=WPI_SolenoidValue."Off", "SolenoidDevRef"=w1572) -> ()  [unwired: 7 in, 2 out]
                    n726 = call-poly <vilib>:"WPI_SolenoidSet.vi"("error in (no error)"=w1568, "Value"=WPI_SolenoidValue."On", "SolenoidDevRef"=w1567) -> ()  [unwired: 7 in, 2 out]
                  }
                }
              }
              n727 = call-poly <vilib>:"WPI_SolenoidSet.vi"("Value"=w1553, "SolenoidDevRef"=w1554) -> ()  [unwired: 8 in, 2 out]
            }
          }
        }
        frame #4 {
          w1576 = -0.7 ("Left axis value")
          n728 = call <vilib>:"WPI_RobotDriveRefNum Registry Get.vi"("refnum name"="RobotDrive") -> ("error out"=w1577:errorcluster, "RobotDriveDevRef"=w1578:T5)  [unwired: 9 in]
          n729 = call <vilib>:"WPI_RobotDriveTankDrive.vi"("error in (no error)"=w1577, "Right axis value"=w1576, "Left axis value"=w1576, "RobotDriveDevRef"=w1578) -> ()  [unwired: 5 in, 3 out]
          n730 = Wait (ms)(milliseconds to wait=1000) -> ()  [unwired: 1 out]
        }
        frame #5 {
          w1584 = 0.0 ("Left axis value")
          n731 = call <vilib>:"WPI_RobotDriveRefNum Registry Get.vi"("refnum name"="RobotDrive") -> ("error out"=w1585:errorcluster, "RobotDriveDevRef"=w1586:T5)  [unwired: 9 in]
          n732 = call <vilib>:"WPI_SolenoidRefNum Registry Get.vi"("refnum name"="GearGate") -> ("error out"=w1582:errorcluster, "SolenoidDevRef"=w1581:T10)  [unwired: 9 in]
          n733 = call <vilib>:"WPI_RobotDriveTankDrive.vi"("error in (no error)"=w1585, "Right axis value"=w1584, "Left axis value"=w1584, "RobotDriveDevRef"=w1586) -> ()  [unwired: 5 in, 3 out]
          n734 = call-poly <vilib>:"WPI_SolenoidSet.vi"("error in (no error)"=w1582, "Value"=WPI_SolenoidValue."Off", "SolenoidDevRef"=w1581) -> ()  [unwired: 7 in, 2 out]
        }
      }
    }
    frame "sideGearleftLoading" {
      n735 = flat-sequence {
        tunnel: [w1595] -> w1587
        tunnel: w1587 -> [w1619]
        frame #0 {
          n736 = call <vilib>:"WPI_SolenoidRefNum Registry Get.vi"("refnum name"="Banana") -> ("SolenoidDevRef"=w1590:T10)  [unwired: 9 in, 1 out]
          n737 = call-poly <vilib>:"WPI_SolenoidSet.vi"("Value"=WPI_SolenoidValue."On", "SolenoidDevRef"=w1590) -> ()  [unwired: 8 in, 2 out]
          n738 = call "ReadFile.vi"("Name"="/home/lvuser/LeftPegPathLoadingZone.txt") -> ("Array - Numeric"=w1595:dbl[][])
          n739 = call <vilib>:"WPI_SolenoidRefNum Registry Get.vi"("refnum name"="GearGate") -> ("error out"=w1594:errorcluster, "SolenoidDevRef"=w1593:T10)  [unwired: 9 in]
          n740 = call-poly <vilib>:"WPI_SolenoidSet.vi"("error in (no error)"=w1594, "Value"=WPI_SolenoidValue."On", "SolenoidDevRef"=w1593) -> ()  [unwired: 7 in, 2 out]
        }
        frame #1 {
          # "Position PID or Velocity PID"
          n741 = call <vilib>:"WPI_SolenoidRefNum Registry Get.vi"("refnum name"="Banana") -> ("SolenoidDevRef"=w1618:T10)  [unwired: 9 in, 1 out]
          n742 = call-poly <vilib>:"WPI_SolenoidSet.vi"("Value"=WPI_SolenoidValue."On", "SolenoidDevRef"=w1618) -> ()  [unwired: 8 in, 2 out]
          n743 = call <vilib>:"WPI_EncoderRefNum Registry Get.vi"("refnum name"="Encoder 0") -> ("error out"=w1612:errorcluster, "EncoderDevRef"=w1611:T14)  [unwired: 9 in]
          n744 = call <vilib>:"WPI_EncoderRefNum Registry Get.vi"("refnum name"="Encoder 1") -> ("error out"=w1614:errorcluster, "EncoderDevRef"=w1613:T14)  [unwired: 9 in]
          n745 = call "Z900_navX_RefNum_Get.vi"("refnum name"="navX") -> ("error out"=w1603:errorcluster, "navX Device"=w1604:T12)  [unwired: 9 in]
          n746 = call "Z900_navX_Set_ZeroYaw.vi"("error in (no error)"=w1603, "navX Device"=w1604) -> ("error out"=w1601:errorcluster, "navX Device"=w1602:T12)  [unwired: 8 in]
          n747 = call <vilib>:"WPI_EncoderReset.vi"("error in (no error)"=w1612, "EncoderDevRef"=w1611) -> ("error out"=w1608:errorcluster, "EncoderDevRef"=w1609:T14)  [unwired: 8 in]
          n748 = call <vilib>:"WPI_EncoderReset.vi"("error in (no error)"=w1614, "EncoderDevRef"=w1613) -> ("error out"=w1607:errorcluster, "EncoderDevRef"=w1610:T14)  [unwired: 8 in]
          n749 = Array Size(array=w1619) -> (size(s)=w1623:i32[])
          n750 = call <vilib>:"WPI_RobotDriveRefNum Registry Get.vi"("refnum name"="RobotDrive") -> ("RobotDriveDevRef"=w1620:T5)  [unwired: 9 in, 1 out]
          n751 = Index Array(array=w1623, index=0) -> (element=w1615:i32)
          n752 = for {
            N: w1615 -> [_]
            tunnel: w1619 -> [w1641]
            tunnel: "PID gains R 4" -> [w1638]
            tunnel: "PID gains L 4" -> [w1637]
            tunnel: "Range 4" -> [w1636]
            tunnel: w1620 -> [w1635]
            tunnel: w1610 -> [w1634]
            tunnel: w1609 -> [w1633]
            tunnel: w1608 -> [w1632]
            tunnel: w1607 -> [w1631]
            tunnel: w1602 -> [w1628]
            tunnel: w1601 -> [w1627]
            i -> [w1640]
            n753 = Index Array(array=w1641, index (row)=w1640) -> (element=w1626:dbl[])  [unwired: 1 in]
            n754 = Index Array(array=w1626, index=0) -> (element=w1629:dbl)
            n755 = Index Array(array=w1626, index=1) -> (element=w1630:dbl)
            n756 = Index Array(array=w1626, index=2) -> (element=w1624:dbl)
            n757 = for {
              N: 10 -> [_]
              tunnel: w1638 -> [w1673]
              tunnel: w1637 -> [w1682]
              tunnel: w1636 -> [w1662]
              tunnel: w1635 -> [w1683]
              tunnel: w1634 -> [w1670]
              tunnel: w1633 -> [w1669]
              tunnel: w1632 -> [w1666]
              tunnel: w1631 -> [w1665]
              tunnel: w1629 -> [w1646]
              tunnel: w1630 -> [w1649]
              tunnel: w1628 -> [w1661]
              tunnel: w1627 -> [w1660]
              tunnel: w1624 -> [w1657]
              w1651 = 0.01
              w1671 = 0.0011393 ("x")
              n758 = call <vilib>:"WPI_EncoderGet.vi"("error in (no error)"=w1665, "EncoderDevRef"=w1670) -> ("Distance"=w1667:dbl)  [unwired: 4 in, 5 out]
              n759 = call <vilib>:"WPI_EncoderGet.vi"("error in (no error)"=w1666, "EncoderDevRef"=w1669) -> ("Distance"=w1668:dbl)  [unwired: 4 in, 5 out]
              n760 = Multiply(x=w1671, y=w1668) -> (x*y=w1672:dbl)
              n761 = Multiply(x=w1671, y=w1667) -> (x*y=w1681:dbl)
              n762 = call "Z900_navX_Get_YPRHfH.vi"("error in (no error)"=w1660, "navX Device"=w1661) -> ("YRPHfH"=w1659:T18)  [unwired: 6 in, 3 out]
              n763 = Unbundle By Name(w1659) -> ("Yaw"=w1658:dbl)
              n764 = call <vilib>:"WPI_SolenoidRefNum Registry Get.vi"("refnum name"="GearGate") -> ("error out"=w1680:errorcluster, "SolenoidDevRef"=w1679:T10)  [unwired: 9 in]
              n765 = call-poly <vilib>:"WPI_SolenoidSet.vi"("error in (no error)"=w1680, "Value"=WPI_SolenoidValue."On", "SolenoidDevRef"=w1679) -> ()  [unwired: 7 in, 2 out]
              n766 = Subtract(x=w1658, y=w1657) -> (x-y=w1656:dbl)
              n767 = Multiply(x=-1.0 ("Speed"), y=w1651) -> (x*y=w1653:dbl)
              n768 = Multiply(x=1.0, y=w1656) -> (x*y=w1654:dbl)
              n769 = Multiply(x=w1653, y=w1654) -> (x*y=w1645:dbl)
              n770 = Add(x=w1646, y=w1645) -> (x+y=w1647:dbl)
              n771 = call-poly <vilib>:"PID.vi"("output range"=w1662, "PID gains"=w1682, "process variable"=w1681, "setpoint"=w1647) -> ("output"=w1663:dbl)  [unwired: 6 in, 1 out]
              n772 = Multiply(x=w1654, y=w1651) -> (x*y=w1648:dbl)
              n773 = Add(x=w1649, y=w1648) -> (x+y=w1650:dbl)
              n774 = call-poly <vilib>:"PID.vi"("output range"=w1662, "PID gains"=w1673, "process variable"=w1672, "setpoint"=w1650) -> ("output"=w1664:dbl)  [unwired: 6 in, 1 out]
              n775 = call <vilib>:"WPI_RobotDriveTankDrive.vi"("Right axis value"=w1664, "Left axis value"=w1663, "RobotDriveDevRef"=w1683) -> ()  [unwired: 6 in, 3 out]
              n776 = call <vilib>:"WPI_SolenoidRefNum Registry Get.vi"("refnum name"="Banana") -> ("SolenoidDevRef"=w1676:T10)  [unwired: 9 in, 1 out]
              n777 = Wait (ms)(milliseconds to wait=10) -> ()  [unwired: 1 out]
              n778 = call-poly <vilib>:"WPI_SolenoidSet.vi"("Value"=WPI_SolenoidValue."On", "SolenoidDevRef"=w1676) -> ()  [unwired: 8 in, 2 out]
            }
          }
        }
        frame #2 {
          w1692 = 0.0 ("Left axis value")
          n779 = call <vilib>:"WPI_SolenoidRefNum Registry Get.vi"("refnum name"="Banana") -> ("SolenoidDevRef"=w1686:T10)  [unwired: 9 in, 1 out]
          n780 = call <vilib>:"WPI_RobotDriveRefNum Registry Get.vi"("refnum name"="RobotDrive") -> ("error out"=w1693:errorcluster, "RobotDriveDevRef"=w1694:T5)  [unwired: 9 in]
          n781 = call <vilib>:"WPI_SolenoidRefNum Registry Get.vi"("refnum name"="GearGate") -> ("error out"=w1690:errorcluster, "SolenoidDevRef"=w1689:T10)  [unwired: 9 in]
          n782 = call-poly <vilib>:"WPI_SolenoidSet.vi"("Value"=WPI_SolenoidValue."On", "SolenoidDevRef"=w1686) -> ()  [unwired: 8 in, 2 out]
          n783 = call <vilib>:"WPI_RobotDriveTankDrive.vi"("error in (no error)"=w1693, "Right axis value"=w1692, "Left axis value"=w1692, "RobotDriveDevRef"=w1694) -> ()  [unwired: 5 in, 3 out]
          n784 = call-poly <vilib>:"WPI_SolenoidSet.vi"("error in (no error)"=w1690, "Value"=WPI_SolenoidValue."On", "SolenoidDevRef"=w1689) -> ()  [unwired: 7 in, 2 out]
        }
        frame #3 {
          n785 = call-poly <vilib>:"NT Read Value.vi"("Name"="Drop Gear?") -> ("Boolean"=w1695:bool)  [unwired: 9 in, 1 out]
          n786 = call <vilib>:"WPI_SolenoidRefNum Registry Get.vi"("refnum name"="Banana") -> ("SolenoidDevRef"=w1699:T10)  [unwired: 9 in, 1 out]
          n787 = case shown="True" w1695 {
            tunnel: w1699 -> [_ w1701]
            tunnel: WPI_SolenoidValue."On" ("Value") -> [_ w1700]
            frame False {
            }
            frame True {
              n788 = for {
                N: 3 -> [_]
                n789 = flat-sequence {
                  frame #0 {
                    n790 = call <vilib>:"WPI_SolenoidRefNum Registry Get.vi"("refnum name"="Gears") -> ("error out"=w1711:errorcluster, "SolenoidDevRef"=w1710:T10)  [unwired: 9 in]
                    n791 = call <vilib>:"WPI_SolenoidRefNum Registry Get.vi"("refnum name"="GearGate") -> ("error out"=w1706:errorcluster, "SolenoidDevRef"=w1705:T10)  [unwired: 9 in]
                    n792 = call-poly <vilib>:"WPI_SolenoidSet.vi"("error in (no error)"=w1711, "Value"=WPI_SolenoidValue."On", "SolenoidDevRef"=w1710) -> ()  [unwired: 7 in, 2 out]
                    n793 = Wait (ms)(milliseconds to wait=166) -> ()  [unwired: 1 out]
                    n794 = call-poly <vilib>:"WPI_SolenoidSet.vi"("error in (no error)"=w1706, "Value"=WPI_SolenoidValue."On", "SolenoidDevRef"=w1705) -> ()  [unwired: 7 in, 2 out]
                  }
                  frame #1 {
                    n795 = call <vilib>:"WPI_SolenoidRefNum Registry Get.vi"("refnum name"="Gears") -> ("error out"=w1720:errorcluster, "SolenoidDevRef"=w1719:T10)  [unwired: 9 in]
                    n796 = call <vilib>:"WPI_SolenoidRefNum Registry Get.vi"("refnum name"="GearGate") -> ("error out"=w1715:errorcluster, "SolenoidDevRef"=w1714:T10)  [unwired: 9 in]
                    n797 = Wait (ms)(milliseconds to wait=166) -> ()  [unwired: 1 out]
                    n798 = call-poly <vilib>:"WPI_SolenoidSet.vi"("error in (no error)"=w1720, "Value"=WPI_SolenoidValue."Off", "SolenoidDevRef"=w1719) -> ()  [unwired: 7 in, 2 out]
                    n799 = call-poly <vilib>:"WPI_SolenoidSet.vi"("error in (no error)"=w1715, "Value"=WPI_SolenoidValue."On", "SolenoidDevRef"=w1714) -> ()  [unwired: 7 in, 2 out]
                  }
                }
              }
              n800 = call-poly <vilib>:"WPI_SolenoidSet.vi"("Value"=w1700, "SolenoidDevRef"=w1701) -> ()  [unwired: 8 in, 2 out]
            }
          }
        }
        frame #4 {
          w1723 = -0.7 ("Left axis value")
          n801 = call <vilib>:"WPI_RobotDriveRefNum Registry Get.vi"("refnum name"="RobotDrive") -> ("error out"=w1724:errorcluster, "RobotDriveDevRef"=w1725:T5)  [unwired: 9 in]
          n802 = call <vilib>:"WPI_RobotDriveTankDrive.vi"("error in (no error)"=w1724, "Right axis value"=w1723, "Left axis value"=w1723, "RobotDriveDevRef"=w1725) -> ()  [unwired: 5 in, 3 out]
          n803 = Wait (ms)(milliseconds to wait=1000) -> ()  [unwired: 1 out]
        }
        frame #5 {
          w1731 = 0.0 ("Left axis value")
          n804 = call <vilib>:"WPI_RobotDriveRefNum Registry Get.vi"("refnum name"="RobotDrive") -> ("error out"=w1732:errorcluster, "RobotDriveDevRef"=w1733:T5)  [unwired: 9 in]
          n805 = call <vilib>:"WPI_SolenoidRefNum Registry Get.vi"("refnum name"="GearGate") -> ("error out"=w1729:errorcluster, "SolenoidDevRef"=w1728:T10)  [unwired: 9 in]
          n806 = call <vilib>:"WPI_RobotDriveTankDrive.vi"("error in (no error)"=w1732, "Right axis value"=w1731, "Left axis value"=w1731, "RobotDriveDevRef"=w1733) -> ()  [unwired: 5 in, 3 out]
          n807 = call-poly <vilib>:"WPI_SolenoidSet.vi"("error in (no error)"=w1729, "Value"=WPI_SolenoidValue."Off", "SolenoidDevRef"=w1728) -> ()  [unwired: 7 in, 2 out]
        }
      }
    }
    frame "sideGearRightLoading" {
      n808 = flat-sequence {
        tunnel: [w1742] -> w1734
        tunnel: w1734 -> [w1766]
        frame #0 {
          n809 = call <vilib>:"WPI_SolenoidRefNum Registry Get.vi"("refnum name"="Banana") -> ("SolenoidDevRef"=w1737:T10)  [unwired: 9 in, 1 out]
          n810 = call-poly <vilib>:"WPI_SolenoidSet.vi"("Value"=WPI_SolenoidValue."On", "SolenoidDevRef"=w1737) -> ()  [unwired: 8 in, 2 out]
          n811 = call "ReadFile.vi"("Name"="/home/lvuser/RightPegPathLoadingZone.txt") -> ("Array - Numeric"=w1742:dbl[][])
          n812 = call <vilib>:"WPI_SolenoidRefNum Registry Get.vi"("refnum name"="GearGate") -> ("error out"=w1741:errorcluster, "SolenoidDevRef"=w1740:T10)  [unwired: 9 in]
          n813 = call-poly <vilib>:"WPI_SolenoidSet.vi"("error in (no error)"=w1741, "Value"=WPI_SolenoidValue."On", "SolenoidDevRef"=w1740) -> ()  [unwired: 7 in, 2 out]
        }
        frame #1 {
          # "Position PID or Velocity PID"
          n814 = call <vilib>:"WPI_SolenoidRefNum Registry Get.vi"("refnum name"="Banana") -> ("SolenoidDevRef"=w1765:T10)  [unwired: 9 in, 1 out]
          n815 = call-poly <vilib>:"WPI_SolenoidSet.vi"("Value"=WPI_SolenoidValue."On", "SolenoidDevRef"=w1765) -> ()  [unwired: 8 in, 2 out]
          n816 = call <vilib>:"WPI_EncoderRefNum Registry Get.vi"("refnum name"="Encoder 0") -> ("error out"=w1759:errorcluster, "EncoderDevRef"=w1758:T14)  [unwired: 9 in]
          n817 = call <vilib>:"WPI_EncoderRefNum Registry Get.vi"("refnum name"="Encoder 1") -> ("error out"=w1761:errorcluster, "EncoderDevRef"=w1760:T14)  [unwired: 9 in]
          n818 = call "Z900_navX_RefNum_Get.vi"("refnum name"="navX") -> ("error out"=w1750:errorcluster, "navX Device"=w1751:T12)  [unwired: 9 in]
          n819 = call "Z900_navX_Set_ZeroYaw.vi"("error in (no error)"=w1750, "navX Device"=w1751) -> ("error out"=w1748:errorcluster, "navX Device"=w1749:T12)  [unwired: 8 in]
          n820 = call <vilib>:"WPI_EncoderReset.vi"("error in (no error)"=w1759, "EncoderDevRef"=w1758) -> ("error out"=w1755:errorcluster, "EncoderDevRef"=w1756:T14)  [unwired: 8 in]
          n821 = call <vilib>:"WPI_EncoderReset.vi"("error in (no error)"=w1761, "EncoderDevRef"=w1760) -> ("error out"=w1754:errorcluster, "EncoderDevRef"=w1757:T14)  [unwired: 8 in]
          n822 = Array Size(array=w1766) -> (size(s)=w1770:i32[])
          n823 = call <vilib>:"WPI_RobotDriveRefNum Registry Get.vi"("refnum name"="RobotDrive") -> ("RobotDriveDevRef"=w1767:T5)  [unwired: 9 in, 1 out]
          n824 = Index Array(array=w1770, index=0) -> (element=w1762:i32)
          n825 = for {
            N: w1762 -> [_]
            tunnel: w1766 -> [w1788]
            tunnel: "PID gains R 5" -> [w1785]
            tunnel: "PID gains L 5" -> [w1784]
            tunnel: "Range 5" -> [w1783]
            tunnel: w1767 -> [w1782]
            tunnel: w1757 -> [w1781]
            tunnel: w1756 -> [w1780]
            tunnel: w1755 -> [w1779]
            tunnel: w1754 -> [w1778]
            tunnel: w1749 -> [w1775]
            tunnel: w1748 -> [w1774]
            i -> [w1787]
            n826 = Index Array(array=w1788, index (row)=w1787) -> (element=w1773:dbl[])  [unwired: 1 in]
            n827 = Index Array(array=w1773, index=0) -> (element=w1776:dbl)
            n828 = Index Array(array=w1773, index=1) -> (element=w1777:dbl)
            n829 = Index Array(array=w1773, index=2) -> (element=w1771:dbl)
            n830 = for {
              N: 10 -> [_]
              tunnel: w1785 -> [w1820]
              tunnel: w1784 -> [w1829]
              tunnel: w1783 -> [w1809]
              tunnel: w1782 -> [w1830]
              tunnel: w1781 -> [w1817]
              tunnel: w1780 -> [w1816]
              tunnel: w1779 -> [w1813]
              tunnel: w1778 -> [w1812]
              tunnel: w1776 -> [w1793]
              tunnel: w1777 -> [w1796]
              tunnel: w1775 -> [w1808]
              tunnel: w1774 -> [w1807]
              tunnel: w1771 -> [w1804]
              w1798 = 0.01
              w1818 = 0.0011393 ("x")
              n831 = call <vilib>:"WPI_EncoderGet.vi"("error in (no error)"=w1812, "EncoderDevRef"=w1817) -> ("Distance"=w1814:dbl)  [unwired: 4 in, 5 out]
              n832 = call <vilib>:"WPI_EncoderGet.vi"("error in (no error)"=w1813, "EncoderDevRef"=w1816) -> ("Distance"=w1815:dbl)  [unwired: 4 in, 5 out]
              n833 = Multiply(x=w1818, y=w1815) -> (x*y=w1819:dbl)
              n834 = Multiply(x=w1818, y=w1814) -> (x*y=w1828:dbl)
              n835 = call "Z900_navX_Get_YPRHfH.vi"("error in (no error)"=w1807, "navX Device"=w1808) -> ("YRPHfH"=w1806:T18)  [unwired: 6 in, 3 out]
              n836 = Unbundle By Name(w1806) -> ("Yaw"=w1805:dbl)
              n837 = call <vilib>:"WPI_SolenoidRefNum Registry Get.vi"("refnum name"="GearGate") -> ("error out"=w1827:errorcluster, "SolenoidDevRef"=w1826:T10)  [unwired: 9 in]
              n838 = call-poly <vilib>:"WPI_SolenoidSet.vi"("error in (no error)"=w1827, "Value"=WPI_SolenoidValue."On", "SolenoidDevRef"=w1826) -> ()  [unwired: 7 in, 2 out]
              n839 = Subtract(x=w1805, y=w1804) -> (x-y=w1803:dbl)
              n840 = Multiply(x=-1.0 ("Speed"), y=w1798) -> (x*y=w1800:dbl)
              n841 = Multiply(x=1.0, y=w1803) -> (x*y=w1801:dbl)
              n842 = Multiply(x=w1800, y=w1801) -> (x*y=w1792:dbl)
              n843 = Add(x=w1793, y=w1792) -> (x+y=w1794:dbl)
              n844 = call-poly <vilib>:"PID.vi"("output range"=w1809, "PID gains"=w1829, "process variable"=w1828, "setpoint"=w1794) -> ("output"=w1810:dbl)  [unwired: 6 in, 1 out]
              n845 = Multiply(x=w1801, y=w1798) -> (x*y=w1795:dbl)
              n846 = Add(x=w1796, y=w1795) -> (x+y=w1797:dbl)
              n847 = call-poly <vilib>:"PID.vi"("output range"=w1809, "PID gains"=w1820, "process variable"=w1819, "setpoint"=w1797) -> ("output"=w1811:dbl)  [unwired: 6 in, 1 out]
              n848 = call <vilib>:"WPI_RobotDriveTankDrive.vi"("Right axis value"=w1811, "Left axis value"=w1810, "RobotDriveDevRef"=w1830) -> ()  [unwired: 6 in, 3 out]
              n849 = call <vilib>:"WPI_SolenoidRefNum Registry Get.vi"("refnum name"="Banana") -> ("SolenoidDevRef"=w1823:T10)  [unwired: 9 in, 1 out]
              n850 = Wait (ms)(milliseconds to wait=10) -> ()  [unwired: 1 out]
              n851 = call-poly <vilib>:"WPI_SolenoidSet.vi"("Value"=WPI_SolenoidValue."On", "SolenoidDevRef"=w1823) -> ()  [unwired: 8 in, 2 out]
            }
          }
        }
        frame #2 {
          w1839 = 0.0 ("Left axis value")
          n852 = call <vilib>:"WPI_SolenoidRefNum Registry Get.vi"("refnum name"="Banana") -> ("SolenoidDevRef"=w1833:T10)  [unwired: 9 in, 1 out]
          n853 = call <vilib>:"WPI_RobotDriveRefNum Registry Get.vi"("refnum name"="RobotDrive") -> ("error out"=w1840:errorcluster, "RobotDriveDevRef"=w1841:T5)  [unwired: 9 in]
          n854 = call <vilib>:"WPI_SolenoidRefNum Registry Get.vi"("refnum name"="GearGate") -> ("error out"=w1837:errorcluster, "SolenoidDevRef"=w1836:T10)  [unwired: 9 in]
          n855 = call-poly <vilib>:"WPI_SolenoidSet.vi"("Value"=WPI_SolenoidValue."On", "SolenoidDevRef"=w1833) -> ()  [unwired: 8 in, 2 out]
          n856 = call <vilib>:"WPI_RobotDriveTankDrive.vi"("error in (no error)"=w1840, "Right axis value"=w1839, "Left axis value"=w1839, "RobotDriveDevRef"=w1841) -> ()  [unwired: 5 in, 3 out]
          n857 = call-poly <vilib>:"WPI_SolenoidSet.vi"("error in (no error)"=w1837, "Value"=WPI_SolenoidValue."On", "SolenoidDevRef"=w1836) -> ()  [unwired: 7 in, 2 out]
        }
        frame #3 {
          n858 = call-poly <vilib>:"NT Read Value.vi"("Name"="Drop Gear?") -> ("Boolean"=w1842:bool)  [unwired: 9 in, 1 out]
          n859 = call <vilib>:"WPI_SolenoidRefNum Registry Get.vi"("refnum name"="Banana") -> ("SolenoidDevRef"=w1846:T10)  [unwired: 9 in, 1 out]
          n860 = case shown="True" w1842 {
            tunnel: w1846 -> [_ w1848]
            tunnel: WPI_SolenoidValue."On" ("Value") -> [_ w1847]
            frame False {
            }
            frame True {
              n861 = for {
                N: 3 -> [_]
                n862 = flat-sequence {
                  frame #0 {
                    n863 = call <vilib>:"WPI_SolenoidRefNum Registry Get.vi"("refnum name"="Gears") -> ("error out"=w1858:errorcluster, "SolenoidDevRef"=w1857:T10)  [unwired: 9 in]
                    n864 = call <vilib>:"WPI_SolenoidRefNum Registry Get.vi"("refnum name"="GearGate") -> ("error out"=w1853:errorcluster, "SolenoidDevRef"=w1852:T10)  [unwired: 9 in]
                    n865 = call-poly <vilib>:"WPI_SolenoidSet.vi"("error in (no error)"=w1858, "Value"=WPI_SolenoidValue."On", "SolenoidDevRef"=w1857) -> ()  [unwired: 7 in, 2 out]
                    n866 = Wait (ms)(milliseconds to wait=166) -> ()  [unwired: 1 out]
                    n867 = call-poly <vilib>:"WPI_SolenoidSet.vi"("error in (no error)"=w1853, "Value"=WPI_SolenoidValue."On", "SolenoidDevRef"=w1852) -> ()  [unwired: 7 in, 2 out]
                  }
                  frame #1 {
                    n868 = call <vilib>:"WPI_SolenoidRefNum Registry Get.vi"("refnum name"="Gears") -> ("error out"=w1867:errorcluster, "SolenoidDevRef"=w1866:T10)  [unwired: 9 in]
                    n869 = call <vilib>:"WPI_SolenoidRefNum Registry Get.vi"("refnum name"="GearGate") -> ("error out"=w1862:errorcluster, "SolenoidDevRef"=w1861:T10)  [unwired: 9 in]
                    n870 = Wait (ms)(milliseconds to wait=166) -> ()  [unwired: 1 out]
                    n871 = call-poly <vilib>:"WPI_SolenoidSet.vi"("error in (no error)"=w1867, "Value"=WPI_SolenoidValue."Off", "SolenoidDevRef"=w1866) -> ()  [unwired: 7 in, 2 out]
                    n872 = call-poly <vilib>:"WPI_SolenoidSet.vi"("error in (no error)"=w1862, "Value"=WPI_SolenoidValue."On", "SolenoidDevRef"=w1861) -> ()  [unwired: 7 in, 2 out]
                  }
                }
              }
              n873 = call-poly <vilib>:"WPI_SolenoidSet.vi"("Value"=w1847, "SolenoidDevRef"=w1848) -> ()  [unwired: 8 in, 2 out]
            }
          }
        }
        frame #4 {
          w1870 = -0.7 ("Left axis value")
          n874 = call <vilib>:"WPI_RobotDriveRefNum Registry Get.vi"("refnum name"="RobotDrive") -> ("error out"=w1871:errorcluster, "RobotDriveDevRef"=w1872:T5)  [unwired: 9 in]
          n875 = call <vilib>:"WPI_RobotDriveTankDrive.vi"("error in (no error)"=w1871, "Right axis value"=w1870, "Left axis value"=w1870, "RobotDriveDevRef"=w1872) -> ()  [unwired: 5 in, 3 out]
          n876 = Wait (ms)(milliseconds to wait=1000) -> ()  [unwired: 1 out]
        }
        frame #5 {
          w1878 = 0.0 ("Left axis value")
          n877 = call <vilib>:"WPI_RobotDriveRefNum Registry Get.vi"("refnum name"="RobotDrive") -> ("error out"=w1879:errorcluster, "RobotDriveDevRef"=w1880:T5)  [unwired: 9 in]
          n878 = call <vilib>:"WPI_SolenoidRefNum Registry Get.vi"("refnum name"="GearGate") -> ("error out"=w1876:errorcluster, "SolenoidDevRef"=w1875:T10)  [unwired: 9 in]
          n879 = call <vilib>:"WPI_RobotDriveTankDrive.vi"("error in (no error)"=w1879, "Right axis value"=w1878, "Left axis value"=w1878, "RobotDriveDevRef"=w1880) -> ()  [unwired: 5 in, 3 out]
          n880 = call-poly <vilib>:"WPI_SolenoidSet.vi"("error in (no error)"=w1876, "Value"=WPI_SolenoidValue."Off", "SolenoidDevRef"=w1875) -> ()  [unwired: 7 in, 2 out]
        }
      }
    }
    frame "Nothing" {
      n881 = flat-sequence {
        frame #0 {
          w1883 = 0.0 ("Left axis value")
          n882 = call <vilib>:"WPI_RobotDriveRefNum Registry Get.vi"("refnum name"="RobotDrive") -> ("error out"=w1884:errorcluster, "RobotDriveDevRef"=w1885:T5)  [unwired: 9 in]
          n883 = Wait (ms)(milliseconds to wait=15000) -> ()  [unwired: 1 out]
          n884 = call <vilib>:"WPI_RobotDriveTankDrive.vi"("error in (no error)"=w1884, "Right axis value"=w1883, "Left axis value"=w1883, "RobotDriveDevRef"=w1885) -> ()  [unwired: 5 in, 3 out]
        }
      }
    }
  }
  n885 = disable-structure shown="Disabled" {
    frame Disabled {
      n886 = call <vilib>:"WPI_SolenoidRefNum Registry Get.vi"("refnum name"="Banana") -> ("SolenoidDevRef"=w1887:T10)  [unwired: 9 in, 1 out]
      n887 = call-poly <vilib>:"WPI_SolenoidSet.vi"("Value"=WPI_SolenoidValue."On", "SolenoidDevRef"=w1887) -> ()  [unwired: 8 in, 2 out]
    }
    frame Enabled {
    }
  }
